vi "utility_panel_multi_axis.vi"() -> (19 "Error Out":errorcluster)   [LabVIEW 2014]
doc: "A Utility Panel that exercises all the primary features of the PMX-4EX-SA controller.\n\nProduced By:\n\n<B>Kod Integrations, LLC</B>\n4835 Marianne Drive\nMount Airy, MD 21771\nhttp://www.kodintegrations.com\nemail: info@kodintegrations.com\nphone: (240) 687-1288"
uses:
  common/controls/motor_status.ctl
  common/controls/complete_motor_state.ctl
  common/controls/single_axis_state.ctl
  common/controls/move_mode.ctl
  common/controls/step_n_loop_motor_status.ctl
  common/controls/jog_pos.ctl
  common/controls/jog_to_strict.ctl
  common/controls/homing_mode.ctl
  common/controls/linear_direction.ctl
  common/controls/axis.ctl
  common/controls/polarity_item.ctl
  common/controls/polarity.ctl
  common/controls/circular_direction.ctl
  common/controls/round_button.ctl
  common/controls/main_test_actions.ctl
  classes/Controller/_Controller.lvclass/_Controller.ctl
  classes/Controller/_Controller.lvclass
  common/controls/multi_axis_read_realtime_actions.ctl
  classes/MultiAxisController/_MultiAxisController.lvclass
  common/controls/counter_type.ctl
  common/controls/motor_enabled_state_axes_group.ctl
  common/controls/movement_item.ctl
  common/controls/digital_output.ctl
  common/controls/step_n_loop_params_write_logic.ctl
  common/controls/step_n_params.ctl
  libraries/common.lvlib
panel:
  in  "pulse_set_u":bool
  in  "pulse_set_z":bool
  in  "pulse_set_y":bool
  in  "pulse_set_x":bool
  in  "pulse_set_val_u":i32
  in  "pulse_set_val_z":i32
  in  "pulse_set_val_y":i32
  in  "pulse_set_val_x":i32
  in  "encoder_set_u":bool
  in  "encoder_set_z":bool
  in  "encoder_set_y":bool
  in  "encoder_set_x":bool
  in  "encoder_set_val_u":i32
  in  "encoder_set_val_z":i32
  in  "encoder_set_val_y":i32
  in  "encoder_set_val_x":i32
  out "U.pulse":i32
  out "Z.pulse":i32
  out "Y.pulse":i32
  out "X.pulse":i32
  in  "exit":bool
  out "response":string
  in  "raw_cmd":string
  in  "write_cmd":bool
  out "U.pos":i32
  out "Z.pos":i32
  out "Y.pos":i32
  out "X.pos":i32
  out "U.SNL_motion_state":T1
  out "U.encoder":i32
  out "U.motion_state":T2
  out "firmware_ver":string
  out "dev_id":string
  out "dev_name":string
  out "Z.SNL_motion_state":T1
  out "Y.SNL_motion_state":T1
  out "X.SNL_motion_state":T1
  out "Z.encoder":i32
  out "Y.encoder":i32
  out "X.encoder":i32
  out "X.motion_state":T2
  out "Y.motion_state":T2
  out "Z.motion_state":T2
  in  "Tab Control":T3(tab)
  in  "goto_interp":bool
  in  "goto_u":bool
  in  "goto_z":bool
  in  "goto_y":bool
  in  "goto_x":bool
  in  "stop_imm_u":bool
  in  "stop_slow_u":bool
  in  "stop_imm_z":bool
  in  "stop_slow_z":bool
  in  "stop_imm_y":bool
  in  "stop_slow_y":bool
  in  "stop_imm_x":bool
  in  "stop_slow_x":bool
  in  "home_dir_u":T4
  in  "home_dir_z":T4
  in  "home_dir_y":T4
  in  "home_dir_x":T4
  in  "jog_dir_u":T4
  in  "jog_dir_z":T4
  in  "jog_dir_y":T4
  in  "jog_dir_x":T4
  in  "mode_u":T5
  in  "home_u":bool
  in  "jog_to_u":T6
  in  "jog_u":T7
  in  "mode_z":T5
  in  "home_z":bool
  in  "jog_to_z":T6
  in  "jog_z":T7
  in  "mode_y":T5
  in  "home_y":bool
  in  "jog_to_y":T6
  in  "jog_y":T7
  in  "mode_x":T5
  in  "home_x":bool
  in  "enabled_u":bool
  in  "enabled_z":bool
  in  "enabled_y":bool
  in  "enabled_x":bool
  in  "jog_to_x":T6
  in  "X.pos_goto":i32
  in  "Y.pos_goto":i32
  in  "Z.pos_goto":i32
  in  "U.pos_goto":i32
  in  "jog_x":T7
  out "sspd_mode_curr":u8=1 min=1 max=7
  in  "t_set_position":bool
  in  "t_position":i32=1
  in  "t_axis":T8
  in  "sspd_set_speed":bool
  in  "sspd_speed":u32=1
  in  "sspd_set_mode":bool
  in  "sspd_mode":u8=1 min=1 max=7
  in  "stop_circ_slow":bool
  in  "stop_circ_imm":bool
  in  "move_circle":bool
  in  "move_arc":bool
  in  "x_coord - arc":i32
  in  "y_coord - arc":i32
  in  "direction - arc":T9
  in  "absolute_angle (degrees) - arc":dbl
  in  "relative_angle (degrees) - arc":dbl
  in  "direction - circle":T9
  in  "y_coord - circle":i32
  in  "x_coord - circle":i32
  in  "stop_arc_slow":bool
  in  "stop_arc_imm":bool
  in  "sspd_axis":T8
  out "step_n_err_range_curr":i32
  out "step_n_tolerance_curr":u32
  out "step_n_ratio_curr":dbl
  out "step_n_max_corr_curr":i32
  in  "set_step_n_params":bool
  in  "step_n_err_range":i32
  in  "step_n_tolerance":u32
  in  "step_n_ratio":dbl
  in  "set_n_correct_attempts":T10
  in  "set_n_err_range?":T10
  in  "set_n_tolerance?":T10
  in  "set_n_ratio?":T10
  in  "step_n_axis":T8
  in  "step_n_max_corr":i32
  in  "enable_disable_step_n":bool
  in  "dig_outs":T11
  out "digital_ins":T12
  out "analog_inputs":T13
  in  "get_non_vol_var":bool
  in  "get_vol_var":bool
  out "non_vol_var_read":string
  out "vol_var_read":string
  in  "set_non_vol_var":bool
  in  "set_vol_var":bool
  in  "non_vol_var_write":i32
  in  "vol_var_write":i32
  in  "non_vol_var_num":u16=50 min=50 max=99
  in  "vol_var_num":u16 max=49
  in  "set_pol_val":bool
  in  "polarity_val":bool
  in  "polarity_option":T14
  out "polarity_out":T15[](array[typedef])
  in  "polarity_axis":T8
  in  "set_device_name":bool
  in  "device_name_id_to_set":i32 min=0 max=99
  out "device_name_to_get":string
  in  "reset_pos":bool
  out "full_state":T16={"X"={"motion_state"=enum."CONST", "other_states"=[]}, "Y"={"motion_state"=enum."CONST", "other_states"=[]}, "Z"={"motion_state"=enum."CONST", "other_states"=[]}, "U"={"motion_state"=enum."CONST", "other_states"=[]}, "buffer_enabled?"=FALSE, "buffer_start"=0, "buffer_end"=0, "avail_buffer"=0, "move_mode"=enum."ABSOLUTE"}
  in  "Error In":errorcluster
  in  "set_speeds":bool
  in  "Z.low_speed":i32
  in  "Y.low_speed":i32
  in  "X.low_speed":i32
  in  "Z.high_speed":i32
  in  "Y.high_speed":i32
  in  "X.high_speed":i32
  out "exit?":bool
  # "Firmware:"
  # "Dev Name:"
  # "Dev ID:"
  # "Positioning and Status"
  # "Encoder\n(Set Value)"
  # "Encoder\n(Read Value)"
  # "Pulse\n(Set Value)"
  # "Pulse\n(Read Value)"
  # "Position"
  # "Current State"
  # "Step N Loop (SNL) State"
  # "(X)"
  # "(Y)"
  # "(Z)"
  # "(U)"
  # "`"
  # "enabled\nstate"
  # "\"Jog To\"\nvalue"
  # "Include?\n(Interpolate)"
  # "Jog\nDirection"
  # "Home\nDirection"
  # "Stop\nSlow"
  # "Stop\nNow!"
  # "axis"
  # "Jog To"
  # "Jog"
  # "Homing Mode"
  # "Home"
  # "(X)"
  # "(Y)"
  # "(Z)"
  # "(U)"
  # "Arc Movements:"
  # "Circular Movements:"
  # "On The Fly Speed (SSPD):"
  # "Axis"
  # "Mode"
  # "Mode (current)"
  # "Speed"
  # "Center X"
  # "Center X"
  # "Center Y"
  # "Center Y"
  # "(mode 1 to 7)"
  # "SET"
  # "SET"
  # "Absolute Angle"
  # "(degrees)"
  # "Direction"
  # "On The Fly Position (T):"
  # "Relative Angle"
  # "(degrees)"
  # "Axis"
  # "Position"
  # "Direction"
  # "SET"
  # "Axis"
  # "Write Values (for chosen Axis)\n(check those to write, then click APPLY)"
  # "Current Values (for chosen Axis)"
  # "Ratio"
  # "Tolerance"
  # "Error Range"
  # "Max Number of Correction Attempts"
  # "Digital Outputs:"
  # "Digital Inputs:"
  # "Analog Inputs:"
  # "Variable ID"
  # "Variable Value (for Write)"
  # "Variable Value (for Read)"
  # "Volatile Variables"
  # "(0-49)"
  # "Non Volatile Variables"
  # "(50-99)"
  # "Axis"
  # "Write Polarity Value"
  # "Current Values (for chosen Axis)"
  # "New Polarity \nValue"
  # "Polarity Type"
  # "Device Name"
  # "SET"
  # "(choose 0 to 99)"
  # "(actual)"
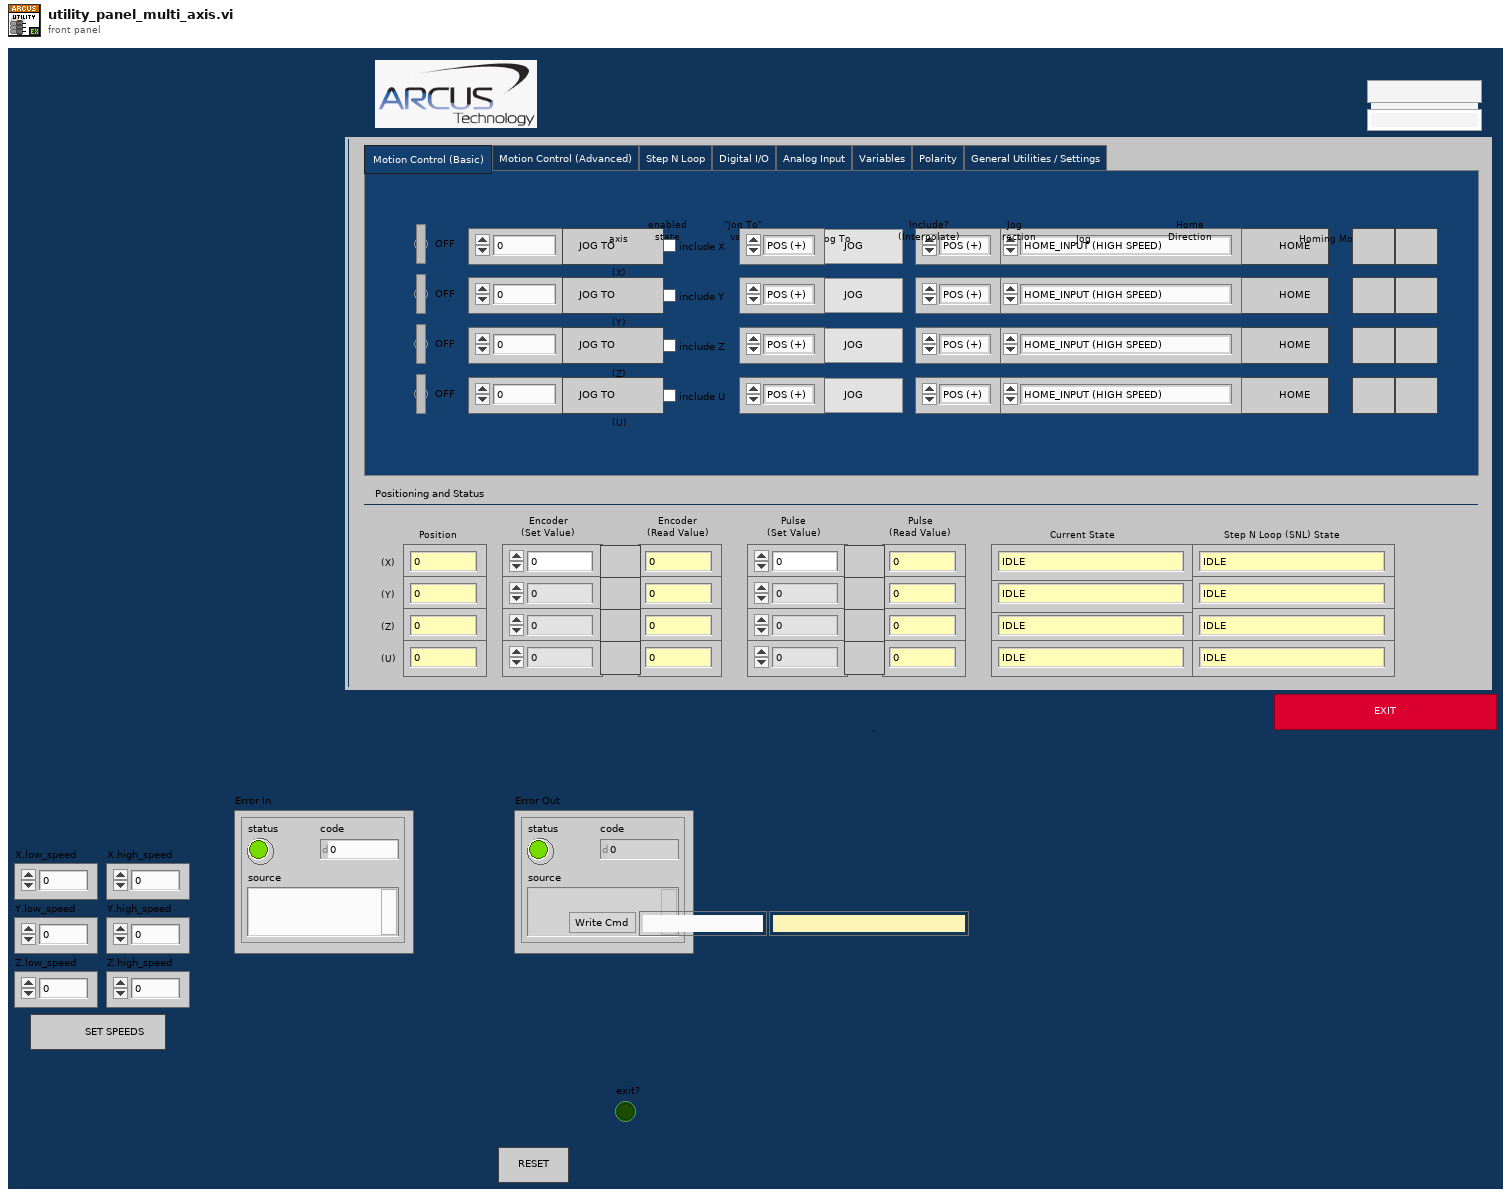
[diagram p1: front panel]
types:
  T1 = typedef "common.lvlib/step_n_loop_motor_status.ctl" = enum16{"IDLE", "MOVING", "CORRECTING", "STOPPING", "ABORTING", "JOGGING", "HOMING", "Z-HOMING", "CORRECT_RANGE_ERR", "CORRECT_ATTEMPT_ERR", "STALL_ERR", "LIMIT_ERR", "NA (SNL NOT ENABLED)", "LIMIT_HOMING"}
  T2 = typedef "common.lvlib/motor_status.ctl" = enum16{"IDLE", "CONST", "ACCEL", "DECEL", "HOME_SWITCH", "-LIMIT_SWITCH", "+LIMIT_SWITCH", "-LIMIT_ERR", "+LIMIT_ERR", "COMM_TIMEOUT", "ALARM_INPUT", "ALARM_ERROR", "TOC_TIMEOUT_STATUS", "LATCH_INPUT_STATUS", "Z_INDEX_STATUS"}
  T3 = enum32{"Motion Control (Basic) ", "Motion Control (Advanced)", "Step N Loop", "Digital I/O", "Analog Input", "Variables", "Polarity", "General Utilities / Settings"}
  T4 = typedef "common.lvlib/linear_direction.ctl" = enum16{"POS (+)", "NEG (-)"}
  T5 = typedef "common.lvlib/homing_mode.ctl" = enum16{"HOME_INPUT (HIGH SPEED)", "LIMIT_INPUT", "HOME_INPUT_&_Z-INDEX", "Z-INDEX", "HOME_INPUT (HIGH_&_LOW_SPEED)"}
  T6 = typedef "common.lvlib/jog_to_strict.ctl" = bool
  T7 = typedef "common.lvlib/jog_pos.ctl" = bool
  T8 = typedef "common.lvlib/axis.ctl" = enum16{"X", "Y", "Z", "U"}
  T9 = typedef "common.lvlib/circular_direction.ctl" = enum16{"CCW", "CW"}
  T10 = typedef "common.lvlib/round_button.ctl" = bool
  T11 = cluster{"Digital Output 1":bool, "Digital Output 2":bool, "Digital Output 3":bool, "Digital Output 4":bool, "Digital Output 5":bool, "Digital Output 6":bool, "Digital Output 7":bool, "Digital Output 8":bool}
  T12 = cluster{"Digital Input 1":bool, "Digital Input 2":bool, "Digital Input 3":bool, "Digital Input 4":bool, "Digital Input 5":bool, "Digital Input 6":bool, "Digital Input 7":bool, "Digital Input 8":bool}
  T13 = cluster{"Analog Input 1":dbl, "Analog Input 2":dbl, "Analog Input 3":dbl, "Analog Input 4":dbl, "Analog Input 5":dbl, "Analog Input 6":dbl, "Analog Input 7":dbl, "Analog Input 8":dbl}
  T14 = typedef "common.lvlib/polarity.ctl" = enum16{"DIRECTION", "LIMIT", "HOME", "DIG_OUT", "DIG_IN", "ENABLE_OUT", "JUMP_ERR", "LATCH", "Z-CHAN_INDEX", "ENCODER_DECODING:1X", "ENCODER_DECODING:2X", "ENCODER_DECODING:4X", "ALARM", "STANDALONE_ERR", "-", "<reserved/nc>"}
  T15 = typedef "common.lvlib/polarity_item.ctl" = cluster{"item":T14, "status":bool}
  T16 = typedef "common.lvlib/complete_motor_state.ctl" = cluster{"X":T17, "Y":T17, "Z":T17, "U":T17, "buffer_enabled?":bool, "buffer_start":i32, "buffer_end":i32, "avail_buffer":i32, "move_mode":T18}
  T17 = typedef "common.lvlib/single_axis_state.ctl" = cluster{"motion_state":T2, "other_states":T2[]}
  T18 = typedef "common.lvlib/move_mode.ctl" = enum16{"ABSOLUTE", "INCREMENTAL"}
  T19 = typedef "common.lvlib/main_test_actions.ctl" = enum16{"-------------------------", "about", "adjust_goto_buttons", "check_model", "close", "connect", "disable_all", "disable_step_n_loop", "enable_all", "enabled_state_change", "enable_step_n_loop", "exit", "get_device_id", "get_device_name", "get_digital_inputs", "get_digital_outputs", "get_firmware_ver", "get_high_speed", "get_high_speed_global", "get_low_speed", "get_low_speed_global", "get_non_volatile_var", "get_on_fly_speed_mode", "get_polarity", "get_product_id", "get_sspd_mode", "get_step_n_params", "get_volatile_var", "goto_x", "goto_y", "goto_z", "goto_u", "goto_interp", "home_x", "home_y", "home_z", "home_u", "init", "init_ui", "jog_x", "jog_y", "jog_z", "jog_u", "lock", "move_arc", "move_circular", "process_events", "run_standalone", "select_device", "stop_standalone", "set_device_name", "set_digital_outputs", "set_encoder_x", "set_encoder_y", "set_encoder_z", "set_encoder_u", "set_high_speed", "set_low_speed", "set_non_volatile_var", "set_on_fly_position", "set_on_fly_speed", "set_on_fly_speed_mode", "set_polarity", "set_pulse_x", "set_pulse_y", "set_pulse_z", "set_pulse_u", "set_step_n_params", "set_volatile_var", "stop_imm_x", "stop_imm_y", "stop_imm_z", "stop_imm_u", "stop_slow_x", "stop_slow_y", "stop_slow_z", "stop_slow_u", "store_perm", "unlock", "wait_til_idle", "zero_counter", "zero_position"}
  T20 = typedef "common.lvlib/models.ctl" = enum16{"<unrecognized>", "ACE-SDC", "ACE-SDE", "ACE-SXC", "ACE-SXE", "DMX-CAN", "DMX-J-SA", "DMX-K-SA", "DMX-UMD", "PMX-2ED-SA", "PMX-2EX-SA", "PMX-4CX-SA", "PMX-4EX-SA"}
  T21 = typedef "common.lvlib/motor_enabled_state_axes_group.ctl" = cluster{"x-axis":bool, "y-axis":bool, "z-axis":bool, "u-axis":bool}
  T22 = typedef "common.lvlib/movement_item.ctl" = cluster{"axis":T8, "target":i32}
  T23 = enum8{"Enabled", "Disabled", "Disabled and Grayed Out"}
  T24 = typedef "common.lvlib/multi_axis_read_realtime_actions.ctl" = enum16{"analog_inputs", "build_processes", "check_status", "encoder_value", "digital_inputs", "motion_state", "position_value", "pulse_value", "snl_motion_state"}
  T25 = typedef "common.lvlib/counter_type.ctl" = enum16{"ENCODER", "PULSE"}
  T26 = typedef "common.lvlib/digital_output_item.ctl" = cluster{"item":T27, "status":bool}
  T27 = typedef "common.lvlib/digital_output.ctl" = enum16{"DIG_OUT_1", "DIG_OUT_2", "DIG_OUT_3", "DIG_OUT_4", "DIG_OUT_5", "DIG_OUT_6", "DIG_OUT_7", "DIG_OUT_8"}
  T28 = cluster{"[0]":bool, "[1]":bool, "[2]":bool, "[3]":bool, "[4]":bool, "[5]":bool, "[6]":bool, "[7]":bool}
  T29 = typedef "common.lvlib/step_n_params.ctl" = cluster{"step_N_loop_ratio":dbl, "tolerance (encoder counts)":u32, "error_range":i32, "max_num_correction_attempts":i32, "enabled?":bool}
  T30 = typedef "common.lvlib/step_n_loop_params_write_logic.ctl" = cluster{"set_ratio?":bool, "set_tolerance?":bool, "set_err_range?":bool, "set_correct_attempts?":bool}
  T31 = typedef "common.lvlib/counter_values.ctl" = cluster{"X":i32, "Y":i32, "Z":i32, "U":i32}
  T32 = typedef "common.lvlib/digital_input_item.ctl" = cluster{"item":T33, "status":bool}
  T33 = typedef "common.lvlib/digital_input.ctl" = enum16{"DIG_IN_1", "DIG_IN_2", "DIG_IN_3", "DIG_IN_4", "DIG_IN_5", "DIG_IN_6", "DIG_IN_7", "DIG_IN_8", "NEG_LIMIT", "HOME", "POS_LIMIT"}
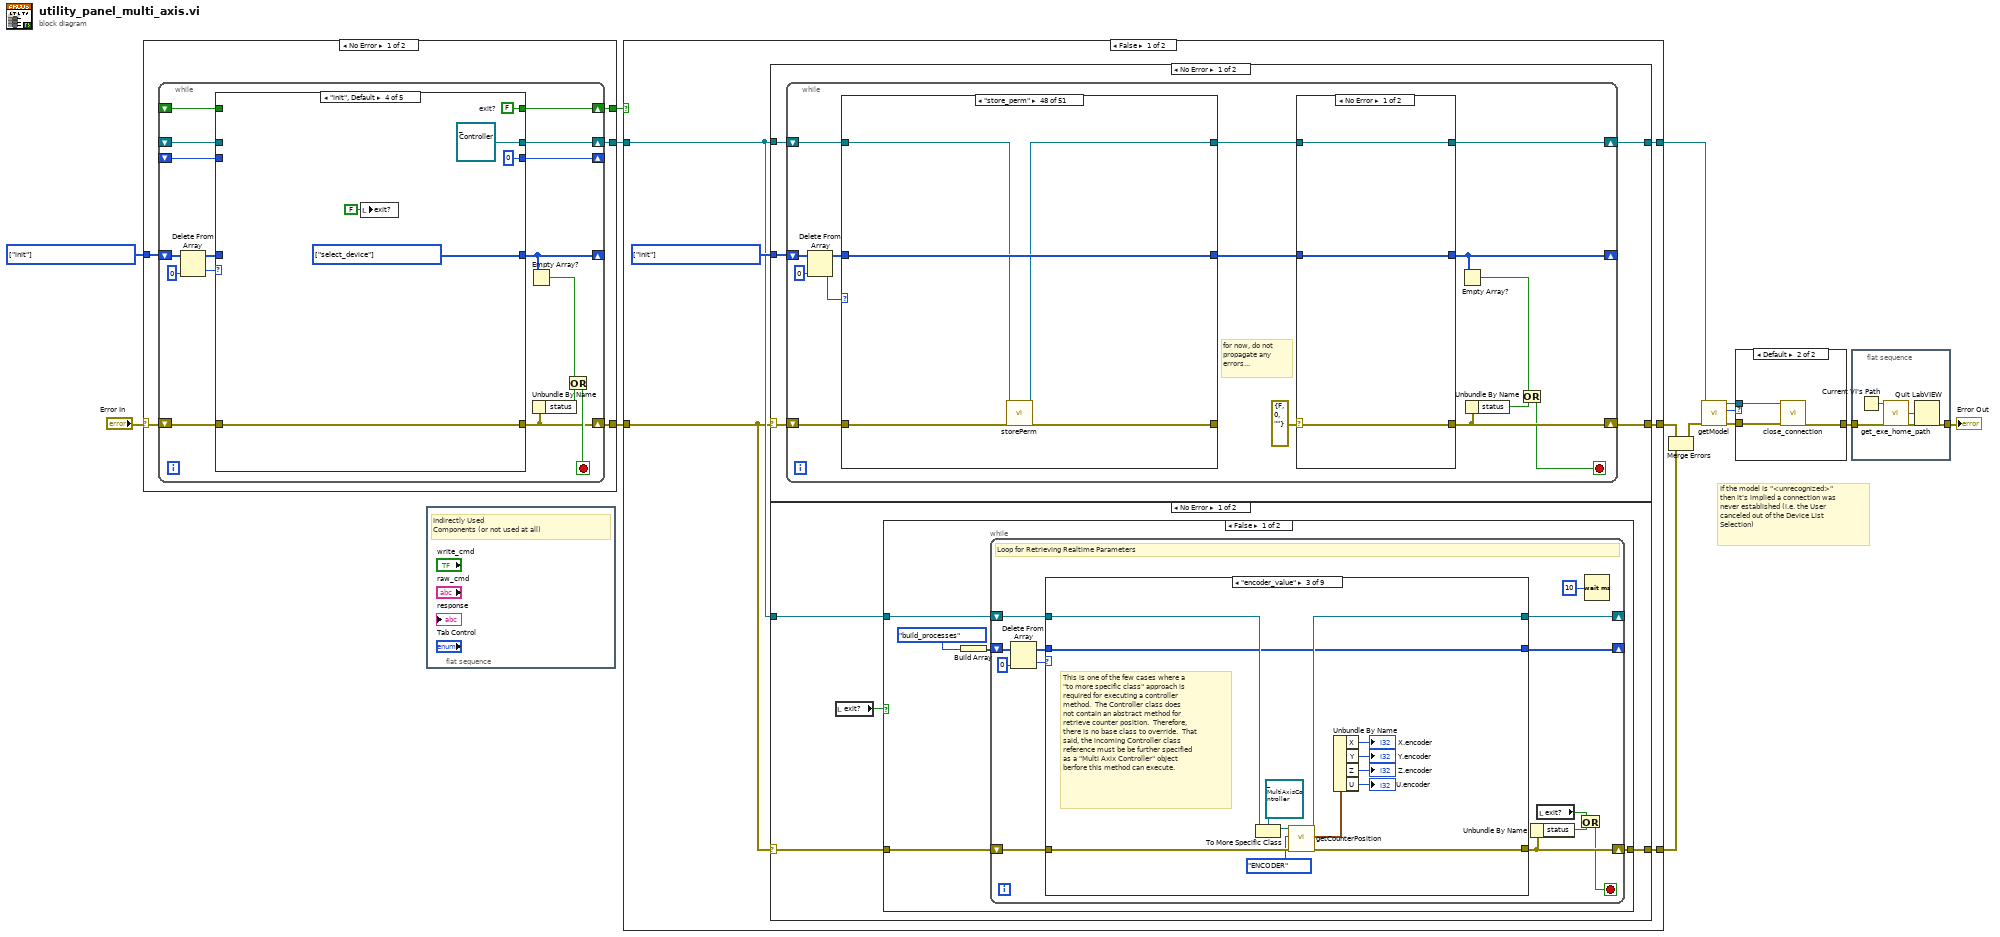
[diagram p0: block diagram]
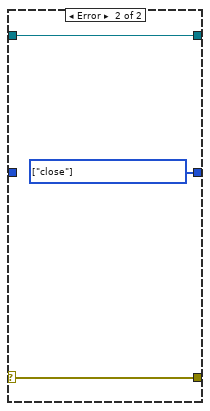
[diagram p3: hidden frame]
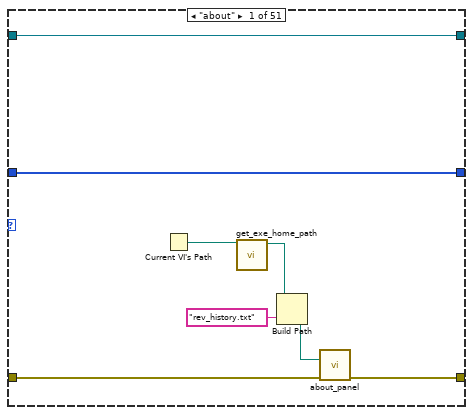
[diagram p4: hidden frame]
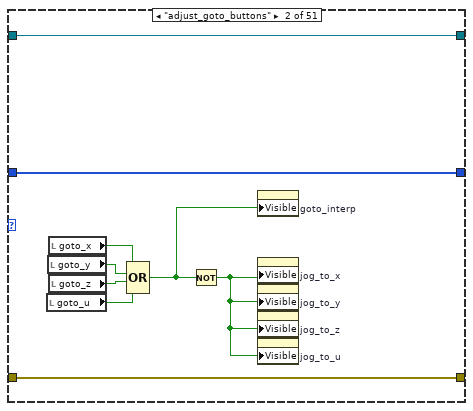
[diagram p5: hidden frame]
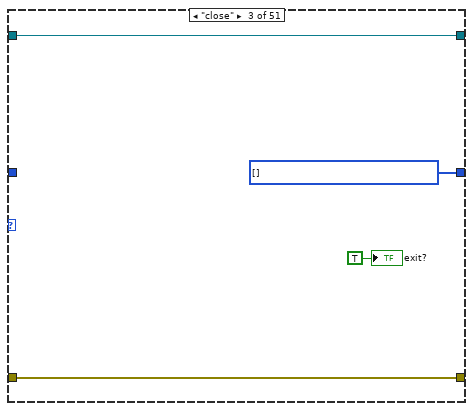
[diagram p6: hidden frame]
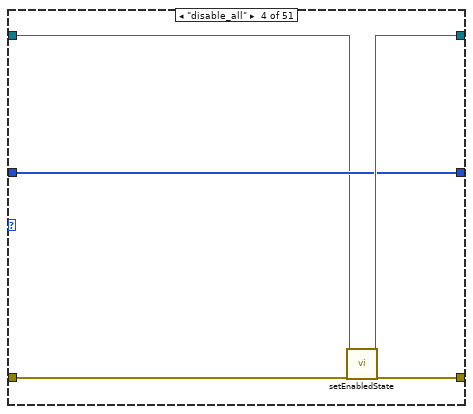
[diagram p7: hidden frame]
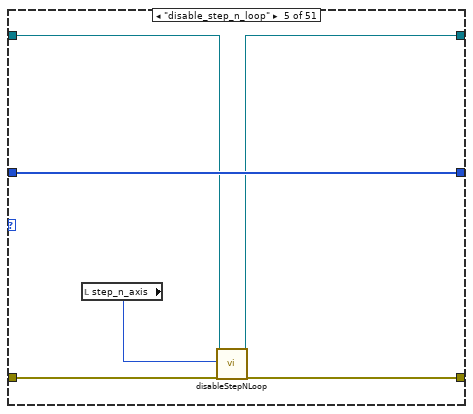
[diagram p8: hidden frame]
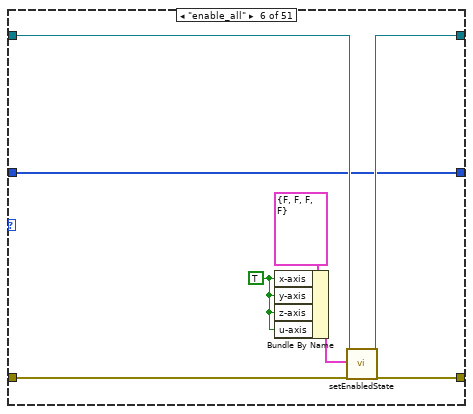
[diagram p9: hidden frame]
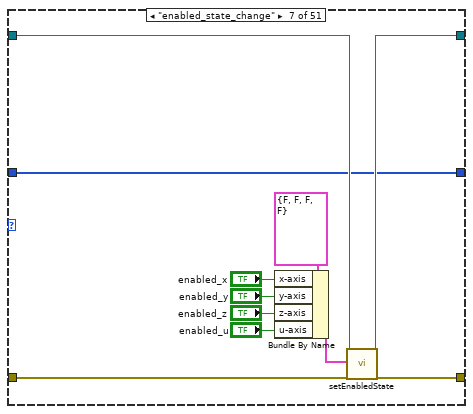
[diagram p10: hidden frame]
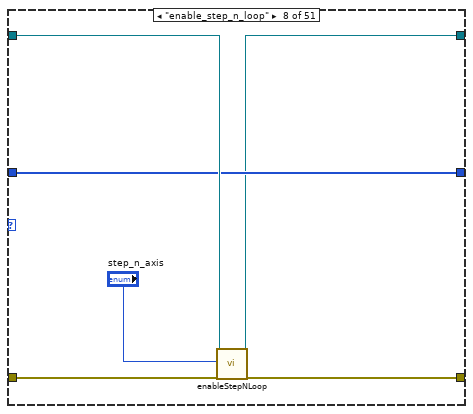
[diagram p11: hidden frame]
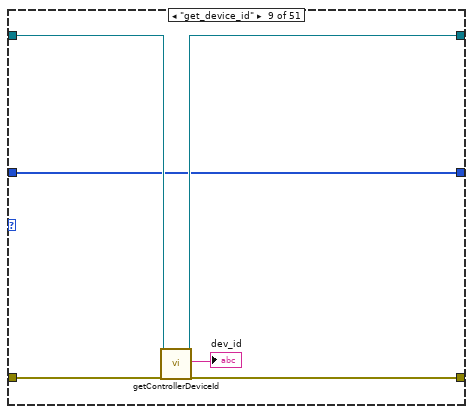
[diagram p12: hidden frame]
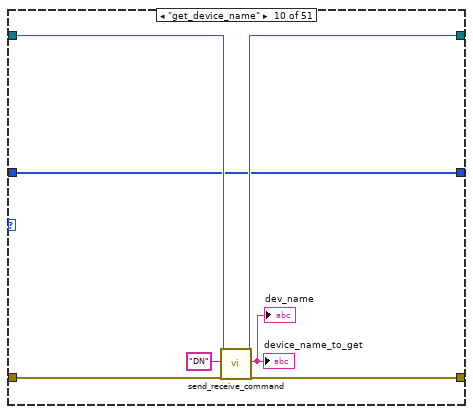
[diagram p13: hidden frame]
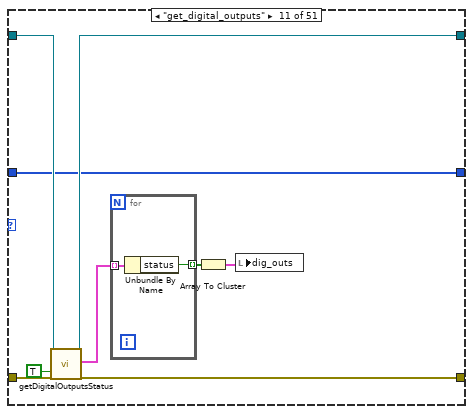
[diagram p14: hidden frame]
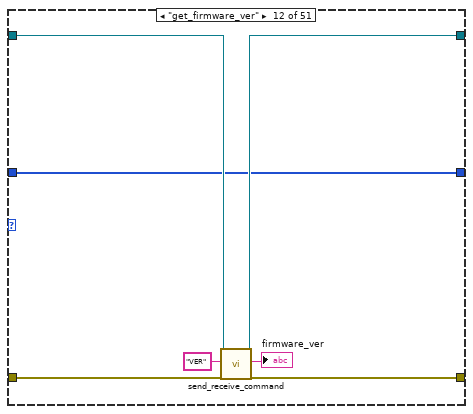
[diagram p15: hidden frame]
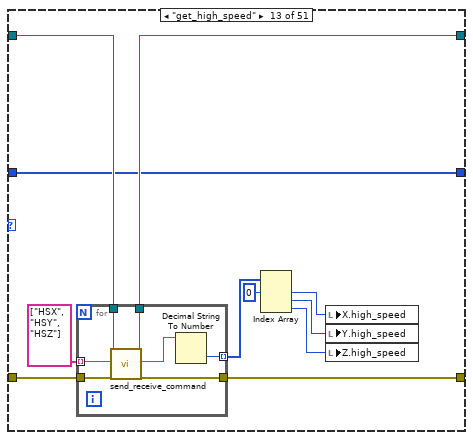
[diagram p16: hidden frame]
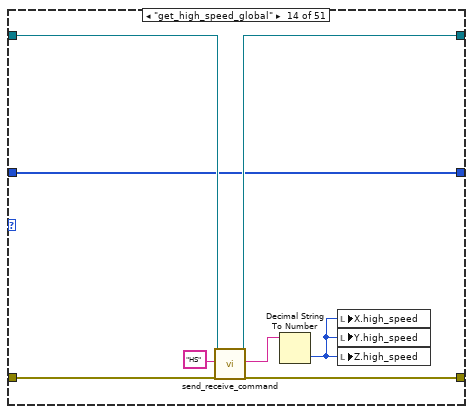
[diagram p17: hidden frame]
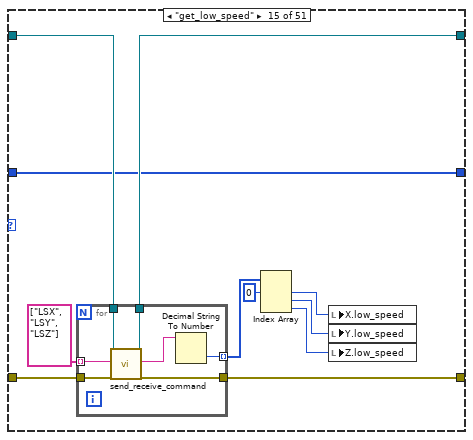
[diagram p18: hidden frame]
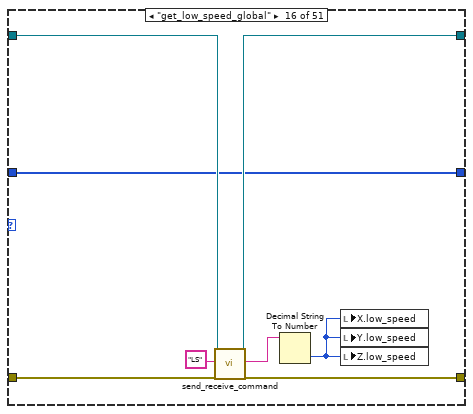
[diagram p19: hidden frame]
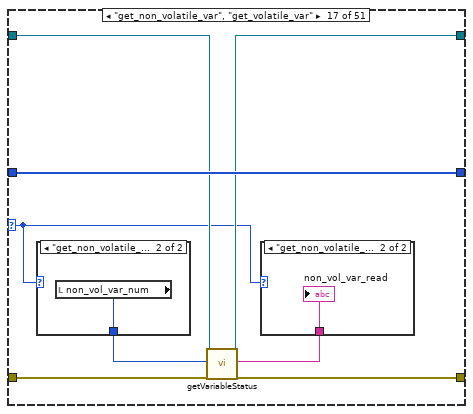
[diagram p20: hidden frame]
diagram:
  w12 = T19[] [enum."init"] items=["-------------------------", "about", "adjust_goto_buttons", "check_model", "close", "connect", "disable_all", "disable_step_n_loop", "enable_all", "enabled_state_change", "enable_step_n_loop", "exit", "get_device_id", "get_device_name", "get_digital_inputs", "get_digital_outputs", "get_firmware_ver", "get_high_speed", "get_high_speed_global", "get_low_speed", "get_low_speed_global", "get_non_volatile_var", "get_on_fly_speed_mode", "get_polarity", "get_product_id", "get_sspd_mode", "get_step_n_params", "get_volatile_var", "goto_x", "goto_y", "goto_z", "goto_u", "goto_interp", "home_x", "home_y", "home_z", "home_u", "init", "init_ui", "jog_x", "jog_y", "jog_z", "jog_u", "lock", "move_arc", "move_circular", "process_events", "run_standalone", "select_device", "stop_standalone", "set_device_name", "set_digital_outputs", "set_encoder_x", "set_encoder_y", "set_encoder_z", "set_encoder_u", "set_high_speed", "set_low_speed", "set_non_volatile_var", "set_on_fly_position", "set_on_fly_speed", "set_on_fly_speed_mode", "set_polarity", "set_pulse_x", "set_pulse_y", "set_pulse_z", "set_pulse_u", "set_step_n_params", "set_volatile_var", "stop_imm_x", "stop_imm_y", "stop_imm_z", "stop_imm_u", "stop_slow_x", "stop_slow_y", "stop_slow_z", "stop_slow_u", "store_perm", "unlock", "wait_til_idle", "zero_counter", "zero_position"]
  # "If the model is \"<unrecognized>\"\nthen it's implied a connection was\nnever established (i.e. the User\ncanceled out of the Device List\nSelection)"
  n1 = case shown="No Error" "Error In" {
    selector: "Error In" -> [w16 w84]
    tunnel: [w19 refnum<class "_Controller.lvclass"> refnum ("reference (out)")] -> w10
    tunnel: w12 -> [w18 _]
    tunnel: [w17 w84] -> w9
    tunnel: [w15 w82] -> w8
    frame No Error {
      n2 = while {
        shift-right: [w29] -> _
        shift-left: w18 -> [w35]
        shift-right: [w26] -> w17
        shift-left: w16 -> [w27]
        shift-right: [w24] -> w19
        shift-left: _ -> [w25]
        shift-right: [w23] -> _
        shift-left: _ -> [w22]
        shift-right: [w21] -> w15
        shift-left: _ -> [w20]
        stop <- w31 stop-if-true
        n3 = Delete From Array(array=w35, index=0) -> (deleted portion=w30:T19, array with subset deleted=w28:T19[])  [unwired: 1 in]
        n4 = case shown="\"init\", Default" w30 {
          tunnel: [w41 w54 w62 w69 w76] -> w29
          tunnel: w28 -> [w40 w54 _ _ _]
          tunnel: w27 -> [w43 w57 w60 w66 w77]
          tunnel: [w42 w56 w60 w66 w75] -> w26
          tunnel: w25 -> [w39 _ w63 _ w72]
          tunnel: [w38 w58 w63 refnum<class "_Controller.lvclass"> refnum ("reference (out)") w72] -> w24
          tunnel: [w37 w55 w61 0 ("index") w71] -> w23
          tunnel: w22 -> [w37 w55 w61 _ _]
          tunnel: [w36 w53 w59 w65 w70] -> w21
          tunnel: w20 -> [w36 w53 _ _ w70]
          frame "check_model" {
            n5 = call "getModel.vi"("error in (no error)"=w43, "reference (in)"=w39) -> ("error out"=w44:errorcluster, "model"=w45:T20, "reference (out)"=w38:refnum<class "_Controller.lvclass">)  [unwired: 7 in]
            n6 = case shown="Default" w45 {
              selector: w45 -> [w47 _]
              tunnel: [w50 w52] -> w42
              tunnel: w44 -> [w50 w52]
              tunnel: [w46 w51] -> w41
              tunnel: w40 -> [_ w51]
              frame Default {
                w46 = T19[] [enum."exit"] items=["-------------------------", "about", "adjust_goto_buttons", "check_model", "close", "connect", "disable_all", "disable_step_n_loop", "enable_all", "enabled_state_change", "enable_step_n_loop", "exit", "get_device_id", "get_device_name", "get_digital_inputs", "get_digital_outputs", "get_firmware_ver", "get_high_speed", "get_high_speed_global", "get_low_speed", "get_low_speed_global", "get_non_volatile_var", "get_on_fly_speed_mode", "get_polarity", "get_product_id", "get_sspd_mode", "get_step_n_params", "get_volatile_var", "goto_x", "goto_y", "goto_z", "goto_u", "goto_interp", "home_x", "home_y", "home_z", "home_u", "init", "init_ui", "jog_x", "jog_y", "jog_z", "jog_u", "lock", "move_arc", "move_circular", "process_events", "run_standalone", "select_device", "stop_standalone", "set_device_name", "set_digital_outputs", "set_encoder_x", "set_encoder_y", "set_encoder_z", "set_encoder_u", "set_high_speed", "set_low_speed", "set_non_volatile_var", "set_on_fly_position", "set_on_fly_speed", "set_on_fly_speed_mode", "set_polarity", "set_pulse_x", "set_pulse_y", "set_pulse_z", "set_pulse_u", "set_step_n_params", "set_volatile_var", "stop_imm_x", "stop_imm_y", "stop_imm_z", "stop_imm_u", "stop_slow_x", "stop_slow_y", "stop_slow_z", "stop_slow_u", "store_perm", "unlock", "wait_til_idle", "zero_counter", "zero_position"]
                n7 = Format Into String(format string="This Control Panel is intended for Multi Axis applications only, with primary focus on the PMX-4EX-SA.  The attached model '%s' is not 100 percent supported in this tool.  Please refer to the example section for a variety of sample codes to suit your needs.\n\nThe application will now close.", w47) -> (resulting string=w48:string)  [unwired: 2 in, 1 out]
                n8 = One Button Dialog(message=w48) -> ()  [unwired: 1 in, 1 out]
              }
              frame "PMX-4EX-SA" {
                # "fully supported"
              }
            }
          }
          frame "connect" {
            n9 = call "initialize.vi"("device_index (in) [0=def]"=w55, "error in (no error)"=w57) -> ("reference (out)"=w58:refnum<class "_Controller.lvclass">, "error out"=w56:errorcluster)  [unwired: 16 in]
          }
          frame "exit" {
            w59 = TRUE  # exit?
            w62 = T19[] [] items=["-------------------------", "about", "adjust_goto_buttons", "check_model", "close", "connect", "disable_all", "disable_step_n_loop", "enable_all", "enabled_state_change", "enable_step_n_loop", "exit", "get_device_id", "get_device_name", "get_digital_inputs", "get_digital_outputs", "get_firmware_ver", "get_high_speed", "get_high_speed_global", "get_low_speed", "get_low_speed_global", "get_non_volatile_var", "get_on_fly_speed_mode", "get_polarity", "get_product_id", "get_sspd_mode", "get_step_n_params", "get_volatile_var", "goto_x", "goto_y", "goto_z", "goto_u", "goto_interp", "home_x", "home_y", "home_z", "home_u", "init", "init_ui", "jog_x", "jog_y", "jog_z", "jog_u", "lock", "move_arc", "move_circular", "process_events", "run_standalone", "select_device", "stop_standalone", "set_device_name", "set_digital_outputs", "set_encoder_x", "set_encoder_y", "set_encoder_z", "set_encoder_u", "set_high_speed", "set_low_speed", "set_non_volatile_var", "set_on_fly_position", "set_on_fly_speed", "set_on_fly_speed_mode", "set_polarity", "set_pulse_x", "set_pulse_y", "set_pulse_z", "set_pulse_u", "set_step_n_params", "set_volatile_var", "stop_imm_x", "stop_imm_y", "stop_imm_z", "stop_imm_u", "stop_slow_x", "stop_slow_y", "stop_slow_z", "stop_slow_u", "store_perm", "unlock", "wait_til_idle", "zero_counter", "zero_position"]
          }
          frame "init", Default {
            w65 = FALSE  # exit?
            w69 = T19[] [enum."select_device"] items=["-------------------------", "about", "adjust_goto_buttons", "check_model", "close", "connect", "disable_all", "disable_step_n_loop", "enable_all", "enabled_state_change", "enable_step_n_loop", "exit", "get_device_id", "get_device_name", "get_digital_inputs", "get_digital_outputs", "get_firmware_ver", "get_high_speed", "get_high_speed_global", "get_low_speed", "get_low_speed_global", "get_non_volatile_var", "get_on_fly_speed_mode", "get_polarity", "get_product_id", "get_sspd_mode", "get_step_n_params", "get_volatile_var", "goto_x", "goto_y", "goto_z", "goto_u", "goto_interp", "home_x", "home_y", "home_z", "home_u", "init", "init_ui", "jog_x", "jog_y", "jog_z", "jog_u", "lock", "move_arc", "move_circular", "process_events", "run_standalone", "select_device", "stop_standalone", "set_device_name", "set_digital_outputs", "set_encoder_x", "set_encoder_y", "set_encoder_z", "set_encoder_u", "set_high_speed", "set_low_speed", "set_non_volatile_var", "set_on_fly_position", "set_on_fly_speed", "set_on_fly_speed_mode", "set_polarity", "set_pulse_x", "set_pulse_y", "set_pulse_z", "set_pulse_u", "set_step_n_params", "set_volatile_var", "stop_imm_x", "stop_imm_y", "stop_imm_z", "stop_imm_u", "stop_slow_x", "stop_slow_y", "stop_slow_z", "stop_slow_u", "store_perm", "unlock", "wait_til_idle", "zero_counter", "zero_position"]
            n10 = local write "exit?"(FALSE ("exit?")) -> ()
          }
          frame "select_device" {
            n11 = call "device_selector_panel.vi"("error in (no error)"=w77) -> ("index"=w71:i32, "cancel?"=w73:bool, "error out"=w74:errorcluster)  [unwired: 10 in, 2 out]
            n12 = case shown="True" w73 {
              tunnel: [w79 w81] -> w76
              tunnel: w74 -> [w78 w80]
              tunnel: [w78 w80] -> w75
              frame False {
                w79 = T19[] [enum."connect", enum."check_model"] items=["-------------------------", "about", "adjust_goto_buttons", "check_model", "close", "connect", "disable_all", "disable_step_n_loop", "enable_all", "enabled_state_change", "enable_step_n_loop", "exit", "get_device_id", "get_device_name", "get_digital_inputs", "get_digital_outputs", "get_firmware_ver", "get_high_speed", "get_high_speed_global", "get_low_speed", "get_low_speed_global", "get_non_volatile_var", "get_on_fly_speed_mode", "get_polarity", "get_product_id", "get_sspd_mode", "get_step_n_params", "get_volatile_var", "goto_x", "goto_y", "goto_z", "goto_u", "goto_interp", "home_x", "home_y", "home_z", "home_u", "init", "init_ui", "jog_x", "jog_y", "jog_z", "jog_u", "lock", "move_arc", "move_circular", "process_events", "run_standalone", "select_device", "stop_standalone", "set_device_name", "set_digital_outputs", "set_encoder_x", "set_encoder_y", "set_encoder_z", "set_encoder_u", "set_high_speed", "set_low_speed", "set_non_volatile_var", "set_on_fly_position", "set_on_fly_speed", "set_on_fly_speed_mode", "set_polarity", "set_pulse_x", "set_pulse_y", "set_pulse_z", "set_pulse_u", "set_step_n_params", "set_volatile_var", "stop_imm_x", "stop_imm_y", "stop_imm_z", "stop_imm_u", "stop_slow_x", "stop_slow_y", "stop_slow_z", "stop_slow_u", "store_perm", "unlock", "wait_til_idle", "zero_counter", "zero_position"]
              }
              frame True {
                w81 = T19[] [enum."exit"] items=["-------------------------", "about", "adjust_goto_buttons", "check_model", "close", "connect", "disable_all", "disable_step_n_loop", "enable_all", "enabled_state_change", "enable_step_n_loop", "exit", "get_device_id", "get_device_name", "get_digital_inputs", "get_digital_outputs", "get_firmware_ver", "get_high_speed", "get_high_speed_global", "get_low_speed", "get_low_speed_global", "get_non_volatile_var", "get_on_fly_speed_mode", "get_polarity", "get_product_id", "get_sspd_mode", "get_step_n_params", "get_volatile_var", "goto_x", "goto_y", "goto_z", "goto_u", "goto_interp", "home_x", "home_y", "home_z", "home_u", "init", "init_ui", "jog_x", "jog_y", "jog_z", "jog_u", "lock", "move_arc", "move_circular", "process_events", "run_standalone", "select_device", "stop_standalone", "set_device_name", "set_digital_outputs", "set_encoder_x", "set_encoder_y", "set_encoder_z", "set_encoder_u", "set_high_speed", "set_low_speed", "set_non_volatile_var", "set_on_fly_position", "set_on_fly_speed", "set_on_fly_speed_mode", "set_polarity", "set_pulse_x", "set_pulse_y", "set_pulse_z", "set_pulse_u", "set_step_n_params", "set_volatile_var", "stop_imm_x", "stop_imm_y", "stop_imm_z", "stop_imm_u", "stop_slow_x", "stop_slow_y", "stop_slow_z", "stop_slow_u", "store_perm", "unlock", "wait_til_idle", "zero_counter", "zero_position"]
              }
            }
          }
        }
        n13 = Empty Array?(array=w29) -> (empty?=w33:bool)
        n14 = Unbundle By Name(w26) -> ("status"=w32:bool)
        n15 = Or(x=w33, y=w32) -> (x .or. y?=w31:bool)
      }
    }
    frame Error {
      w82 = TRUE  # exit?
    }
  }
  n16 = flat-sequence {
    frame #0 {
      # "Indirectly Used \nComponents (or not used at all)"
    }
  }
  n17 = case shown="False" w8 {
    tunnel: [w90 w984] -> w6
    tunnel: [w89 w983] -> w14
    tunnel: [w88 w983] -> w13
    tunnel: w10 -> [w86 w984]
    tunnel: w9 -> [w85 w983]
    frame False {
      w87 = T19[] [enum."init"] items=["-------------------------", "about", "adjust_goto_buttons", "check_model", "close", "connect", "disable_all", "disable_step_n_loop", "enable_all", "enabled_state_change", "enable_step_n_loop", "exit", "get_device_id", "get_device_name", "get_digital_inputs", "get_digital_outputs", "get_firmware_ver", "get_high_speed", "get_high_speed_global", "get_low_speed", "get_low_speed_global", "get_non_volatile_var", "get_on_fly_speed_mode", "get_polarity", "get_product_id", "get_sspd_mode", "get_step_n_params", "get_volatile_var", "goto_x", "goto_y", "goto_z", "goto_u", "goto_interp", "home_x", "home_y", "home_z", "home_u", "init", "init_ui", "jog_x", "jog_y", "jog_z", "jog_u", "lock", "move_arc", "move_circular", "process_events", "run_standalone", "select_device", "stop_standalone", "set_device_name", "set_digital_outputs", "set_encoder_x", "set_encoder_y", "set_encoder_z", "set_encoder_u", "set_high_speed", "set_low_speed", "set_non_volatile_var", "set_on_fly_position", "set_on_fly_speed", "set_on_fly_speed_mode", "set_polarity", "set_pulse_x", "set_pulse_y", "set_pulse_z", "set_pulse_u", "set_step_n_params", "set_volatile_var", "stop_imm_x", "stop_imm_y", "stop_imm_z", "stop_imm_u", "stop_slow_x", "stop_slow_y", "stop_slow_z", "stop_slow_u", "store_perm", "unlock", "wait_til_idle", "zero_counter", "zero_position"]
      n18 = case shown="No Error" w85 {
        selector: w85 -> [w91 w827]
        tunnel: [w95 w826] -> w90
        tunnel: w86 -> [w94 w826]
        tunnel: w87 -> [w93 _]
        tunnel: [w92 w827] -> w89
        frame No Error {
          n19 = while {
            shift-right: [w102] -> _
            shift-left: w93 -> [w110]
            shift-right: [w100] -> w92
            shift-left: w91 -> [w106]
            shift-right: [w101] -> w95
            shift-left: w94 -> [w105]
            stop <- w97 stop-if-true
            # "for now, do not\npropagate any\nerrors..."
            n20 = Delete From Array(array=w110, index=0) -> (deleted portion=w108:T19, array with subset deleted=w107:T19[])  [unwired: 1 in]
            n21 = case shown="\"store_perm\"" w108 {
              selector: w108 -> [_ _ _ _ _ _ _ _ _ _ _ _ _ _ _ _ w258 _ _ _ _ w309 _ w355 _ _ w386 _ _ _ _ _ _ _ w617 _ _ _ _ _ _ _ w712 _ _ w757 w768 _ _ _ _]
              tunnel: [w119 w133 w135 w142 w145 w155 w166 w170 w176 w182 w192 w199 w213 w228 w239 w254 w261 w274 w284 w288 w301 w312 w339 w357 w375 w383 w388 w407 w418 w428 w560 w568 w581 w608 w619 w642 w659 w670 w680 w687 w694 w700 w714 w744 w748 w759 w770 w780 w785 w807 w818] -> w103
              tunnel: [w118 w132 w137 w139 w148 w150 w161 w171 w175 w181 w188 w198 w205 w226 w231 w252 w264 w273 w281 w287 w302 w314 w325 w356 w374 w379 w387 w406 w417 w426 w562 w566 w580 w602 w618 w638 w652 w676 w677 w686 w693 w702 w713 w743 w755 w758 w769 w782 w783 w805 w816] -> w104
              tunnel: w107 -> [w118 w132 _ w139 w148 w150 w161 w171 w175 w181 w188 w198 w205 w226 w231 w252 w264 w273 w281 w287 w302 w314 w325 w356 _ w380 w387 w406 w417 w425 w562 w566 w580 w602 w618 w638 w652 w676 w677 w686 w693 w702 w713 w743 w755 w758 w769 w782 w783 w805 w816]
              tunnel: w106 -> [w121 w131 w136 w141 w147 w154 w165 w173 w179 w185 w195 w203 w215 w230 w241 w256 w263 w278 w285 w291 w304 w311 w338 w360 w373 w382 w391 w412 w423 w427 w564 w570 w579 w607 w622 w644 w661 w675 w683 w690 w698 w709 w717 w747 w754 w762 w773 w779 w787 w809 w820]
              tunnel: [w120 w131 w136 w140 w143 w153 w164 w169 w178 w184 w194 w202 w212 w227 w238 w253 w260 w277 w283 w290 w300 w310 w337 w359 w373 w382 w390 w405 w416 w424 w559 w567 w582 w606 w621 w641 w658 w669 w682 w689 w697 w701 w716 w746 w749 w761 w772 w778 w784 w806 w817] -> _
              tunnel: w105 -> [w119 w133 w135 w138 w146 w156 w167 w172 w177 w183 w193 w200 w214 w229 w240 w255 w262 w275 w286 w289 w303 w313 w340 w358 w375 w383 w389 w411 w422 w428 w563 w569 w576 w609 w620 w643 w660 w671 w681 w688 w695 w710 w715 w745 w752 w760 w771 w781 w786 w808 w819]
              frame "about" {
                n22 = Current VI's Path() -> (path=w117:path)
                n23 = call "get_exe_home_path.vi"("home_path"=w117) -> ("actual_home_path"=w122:path)  [unwired: 6 in, 1 out]
                n24 = Build Path(base path=w122, name or relative path="rev_history.txt") -> (appended path=w123:path)
                n25 = call "about_panel.vi"("rev_history_filepath"=w123, "error in (no error)"=w121) -> ("error out"=w120:errorcluster)  [unwired: 13 in]
              }
              frame "adjust_goto_buttons" {
                n26 = local read "goto_u"() -> (w129:bool)
                n27 = local read "goto_y"() -> (w128:bool)
                n28 = local read "goto_x"() -> (w130:bool)
                n29 = local read "goto_z"() -> (w127:bool)
                n30 = Compound Arithmetic op=OR(w130, w128, w127, w129) -> (w126:bool)
                n31 = Not(x=w126) -> (.not. x?=w125:bool)
                n32 = property on="goto_interp" class="Bool"("Visible"=w126) -> ()  [unwired: 2 in, 2 out]
                n33 = property on="jog_to_x" class="Bool"("Visible"=w125) -> ()  [unwired: 2 in, 2 out]
                n34 = property on="jog_to_y" class="Bool"("Visible"=w125) -> ()  [unwired: 2 in, 2 out]
                n35 = property on="jog_to_z" class="Bool"("Visible"=w125) -> ()  [unwired: 2 in, 2 out]
                n36 = property on="jog_to_u" class="Bool"("Visible"=w125) -> ()  [unwired: 2 in, 2 out]
              }
              frame "close" {
                w137 = T19[] [] items=["-------------------------", "about", "adjust_goto_buttons", "check_model", "close", "connect", "disable_all", "disable_step_n_loop", "enable_all", "enabled_state_change", "enable_step_n_loop", "exit", "get_device_id", "get_device_name", "get_digital_inputs", "get_digital_outputs", "get_firmware_ver", "get_high_speed", "get_high_speed_global", "get_low_speed", "get_low_speed_global", "get_non_volatile_var", "get_on_fly_speed_mode", "get_polarity", "get_product_id", "get_sspd_mode", "get_step_n_params", "get_volatile_var", "goto_x", "goto_y", "goto_z", "goto_u", "goto_interp", "home_x", "home_y", "home_z", "home_u", "init", "init_ui", "jog_x", "jog_y", "jog_z", "jog_u", "lock", "move_arc", "move_circular", "process_events", "run_standalone", "select_device", "stop_standalone", "set_device_name", "set_digital_outputs", "set_encoder_x", "set_encoder_y", "set_encoder_z", "set_encoder_u", "set_high_speed", "set_low_speed", "set_non_volatile_var", "set_on_fly_position", "set_on_fly_speed", "set_on_fly_speed_mode", "set_polarity", "set_pulse_x", "set_pulse_y", "set_pulse_z", "set_pulse_u", "set_step_n_params", "set_volatile_var", "stop_imm_x", "stop_imm_y", "stop_imm_z", "stop_imm_u", "stop_slow_x", "stop_slow_y", "stop_slow_z", "stop_slow_u", "store_perm", "unlock", "wait_til_idle", "zero_counter", "zero_position"]
                "exit?" <- TRUE ("exit?")
              }
              frame "disable_all" {
                n37 = call-dynamic "setEnabledState.vi"("Controller in"=w138, "error in (no error)"=w141) -> ("Controller out"=w142:refnum<class "_Controller.lvclass">, "error out"=w140:errorcluster)  [unwired: 14 in, 2 out]
              }
              frame "disable_step_n_loop" {
                n38 = local read "step_n_axis"() -> (w144:T8)
                n39 = call-dynamic "disableStepNLoop.vi"("Controller in"=w146, "axis (for multi-axis applications only - otherwise ignored)"=w144, "error in (no error)"=w147) -> ("Controller out"=w145:refnum<class "_Controller.lvclass">, "error out"=w143:errorcluster)  [unwired: 13 in, 2 out]
              }
              frame "enable_all" {
                w149 = TRUE ("x-axis")
                n40 = Bundle By Name(cluster=T21 {"x-axis"=FALSE, "y-axis"=FALSE, "z-axis"=FALSE, "u-axis"=FALSE} ("axes_states (for multi-axis applications only)"), "x-axis"=w149, "y-axis"=w149, "z-axis"=w149, "u-axis"=w149) -> (w151:T21)
                n41 = call-dynamic "setEnabledState.vi"("Controller in"=w156, "axes_states (for multi-axis applications only) - (def = DISABLED)"=w151, "error in (no error)"=w154) -> ("Controller out"=w155:refnum<class "_Controller.lvclass">, "error out"=w153:errorcluster)  [unwired: 13 in, 2 out]
              }
              frame "enabled_state_change" {
                n42 = Bundle By Name(cluster=T21 {"x-axis"=FALSE, "y-axis"=FALSE, "z-axis"=FALSE, "u-axis"=FALSE} ("axes_states (for multi-axis applications only)"), "x-axis"="enabled_x", "y-axis"="enabled_y", "z-axis"="enabled_z", "u-axis"="enabled_u") -> (w162:T21)
                n43 = call-dynamic "setEnabledState.vi"("Controller in"=w167, "axes_states (for multi-axis applications only) - (def = DISABLED)"=w162, "error in (no error)"=w165) -> ("Controller out"=w166:refnum<class "_Controller.lvclass">, "error out"=w164:errorcluster)  [unwired: 13 in, 2 out]
              }
              frame "enable_step_n_loop" {
                n44 = call-dynamic "enableStepNLoop.vi"("Controller in"=w172, "axis (for multi-axis applications only - otherwise ignored)"="step_n_axis", "error in (no error)"=w173) -> ("Controller out"=w170:refnum<class "_Controller.lvclass">, "error out"=w169:errorcluster)  [unwired: 13 in, 2 out]
              }
              frame "get_device_id" {
                n45 = call "getControllerDeviceId.vi"("reference (in)"=w177, "error in (no error)"=w179) -> ("reference (out)"=w176:refnum<class "_Controller.lvclass">, "device_id (out)"=→"dev_id":string, "error out"=w178:errorcluster)  [unwired: 15 in]
              }
              frame "get_device_name" {
                n46 = call "send_receive_command.vi"("reference (in)"=w183, "ASCII Command (in)"="DN", "error in (no error)"=w185) -> ("reference (out)"=w182:refnum<class "_Controller.lvclass">, "response (out)"=→"device_name_to_get" →"dev_name":string, "error out"=w184:errorcluster)  [unwired: 12 in, 2 out]
              }
              frame "get_digital_outputs" {
                n47 = call "getDigitalOutputsStatus.vi"("Controller in"=w193, "get_all? (def=F)"=TRUE, "error in (no error)"=w195) -> ("Controller out"=w192:refnum<class "_Controller.lvclass">, "do_items"=w191:T26[], "error out"=w194:errorcluster)  [unwired: 12 in, 2 out]
                n48 = for {
                  tunnel: w191 -> [w197] mode=indexing
                  tunnel: [w196] -> w190 mode=indexing
                  n49 = Unbundle By Name(w197) -> ("status"=w196:bool)
                }
                n50 = Array To Cluster(array=w190) -> (cluster=w189:T28)
                n51 = local write "dig_outs"(w189) -> ()
              }
              frame "get_firmware_ver" {
                n52 = call "send_receive_command.vi"("reference (in)"=w200, "ASCII Command (in)"="VER", "error in (no error)"=w203) -> ("reference (out)"=w199:refnum<class "_Controller.lvclass">, "response (out)"=→"firmware_ver":string, "error out"=w202:errorcluster)  [unwired: 12 in, 2 out]
              }
              frame "get_high_speed" {
                n53 = for {
                  tunnel: w215 -> [w222]
                  tunnel: w214 -> [w221]
                  tunnel: [w220] -> w213
                  tunnel: [w219] -> w212
                  tunnel: string[] ["HSX", "HSY", "HSZ"] -> [w218] mode=indexing
                  tunnel: [w216] -> w209 mode=indexing
                  n54 = call "send_receive_command.vi"("reference (in)"=w221, "ASCII Command (in)"=w218, "error in (no error)"=w222) -> ("reference (out)"=w220:refnum<class "_Controller.lvclass">, "response (out)"=w217:string, "error out"=w219:errorcluster)  [unwired: 12 in, 2 out]
                  n55 = Decimal String To Number(string=w217) -> (number=w216:i32)  [unwired: 2 in, 1 out]
                }
                n56 = Index Array(array=w209, index #1=0 ("index")) -> (element #1=w208:i32, element #2=w207:i32, element #3=w206:i32)  [unwired: 2 in]
                n57 = local write "X.high_speed"(w208) -> ()
                n58 = local write "Y.high_speed"(w207) -> ()
                n59 = local write "Z.high_speed"(w206) -> ()
              }
              frame "get_high_speed_global" {
                n60 = call "send_receive_command.vi"("reference (in)"=w229, "ASCII Command (in)"="HS", "error in (no error)"=w230) -> ("reference (out)"=w228:refnum<class "_Controller.lvclass">, "response (out)"=w225:string, "error out"=w227:errorcluster)  [unwired: 12 in, 2 out]
                n61 = Decimal String To Number(string=w225) -> (number=w224:i32)  [unwired: 2 in, 1 out]
                n62 = local write "X.high_speed"(w224) -> ()
                n63 = local write "Y.high_speed"(w224) -> ()
                n64 = local write "Z.high_speed"(w224) -> ()
              }
              frame "get_low_speed" {
                n65 = for {
                  tunnel: w241 -> [w248]
                  tunnel: w240 -> [w247]
                  tunnel: [w246] -> w239
                  tunnel: [w245] -> w238
                  tunnel: string[] ["LSX", "LSY", "LSZ"] -> [w244] mode=indexing
                  tunnel: [w242] -> w235 mode=indexing
                  n66 = call "send_receive_command.vi"("reference (in)"=w247, "ASCII Command (in)"=w244, "error in (no error)"=w248) -> ("reference (out)"=w246:refnum<class "_Controller.lvclass">, "response (out)"=w243:string, "error out"=w245:errorcluster)  [unwired: 12 in, 2 out]
                  n67 = Decimal String To Number(string=w243) -> (number=w242:i32)  [unwired: 2 in, 1 out]
                }
                n68 = Index Array(array=w235, index #1=0 ("index")) -> (element #1=w234:i32, element #2=w233:i32, element #3=w232:i32)  [unwired: 2 in]
                n69 = local write "X.low_speed"(w234) -> ()
                n70 = local write "Y.low_speed"(w233) -> ()
                n71 = local write "Z.low_speed"(w232) -> ()
              }
              frame "get_low_speed_global" {
                n72 = call "send_receive_command.vi"("reference (in)"=w255, "ASCII Command (in)"="LS", "error in (no error)"=w256) -> ("reference (out)"=w254:refnum<class "_Controller.lvclass">, "response (out)"=w251:string, "error out"=w253:errorcluster)  [unwired: 12 in, 2 out]
                n73 = Decimal String To Number(string=w251) -> (number=w250:i32)  [unwired: 2 in, 1 out]
                n74 = local write "X.low_speed"(w250) -> ()
                n75 = local write "Y.low_speed"(w250) -> ()
                n76 = local write "Z.low_speed"(w250) -> ()
              }
              frame "get_non_volatile_var", "get_volatile_var" {
                n77 = case shown="\"get_non_volatile_var\"" w258 {
                  tunnel: [w267 w268] -> w259
                  frame "get_volatile_var", Default {
                    n78 = local read "vol_var_num"() -> (w267:u16)
                  }
                  frame "get_non_volatile_var" {
                    n79 = local read "non_vol_var_num"() -> (w268:u16)
                  }
                }
                n80 = call-dynamic "getVariableStatus.vi"("Controller in"=w262, "var_number"=w259, "error in (no error)"=w263) -> ("Controller out"=w261:refnum<class "_Controller.lvclass">, "var_value"=w257:string, "error out"=w260:errorcluster)  [unwired: 14 in]
                n81 = case shown="\"get_non_volatile_var\"" w258 {
                  tunnel: w257 -> [w265 w266]
                  frame "get_volatile_var", Default {
                    "vol_var_read" <- w265
                  }
                  frame "get_non_volatile_var" {
                    "non_vol_var_read" <- w266
                  }
                }
              }
              frame "get_on_fly_speed_mode" {
                n82 = local read "sspd_axis"() -> (w272:T8)
                n83 = Format Into String(format string="SSPDM%s", w272) -> (resulting string=w276:string)  [unwired: 2 in, 1 out]
                n84 = call "send_receive_command.vi"("reference (in)"=w275, "ASCII Command (in)"=w276, "error in (no error)"=w278) -> ("reference (out)"=w274:refnum<class "_Controller.lvclass">, "response (out)"=w271:string, "error out"=w277:errorcluster)  [unwired: 12 in, 2 out]
                n85 = Decimal String To Number(string=w271) -> (number=w269:i32)  [unwired: 2 in, 1 out]
                n86 = To Unsigned Byte Integer(number=w269) -> (unsigned 8bit integer=→"sspd_mode_curr":u8)
              }
              frame "get_polarity" {
                n87 = local read "polarity_axis"() -> (w282:T8)
                n88 = call-dynamic "getPolarity.vi"("Controller in"=w286, "axis (def=X)"=w282, "error in (no error)"=w285) -> ("Controller out"=w284:refnum<class "_Controller.lvclass">, "polarity_items (out)"=→"polarity_out":T15[], "error out"=w283:errorcluster)  [unwired: 14 in]
              }
              frame "get_product_id" {
                n89 = call "send_receive_command.vi"("reference (in)"=w289, "ASCII Command (in)"="ID", "error in (no error)"=w291) -> ("reference (out)"=w288:refnum<class "_Controller.lvclass">, "error out"=w290:errorcluster)  [unwired: 12 in, 3 out]
              }
              frame "get_step_n_params" {
                n90 = local read "step_n_axis"() -> (w299:T8)
                n91 = call-dynamic "getStepNLoopParams.vi"("Controller in"=w303, "axis (only applicable to multi-axis applications)"=w299, "error in (no error)"=w304) -> ("Controller out"=w301:refnum<class "_Controller.lvclass">, "step_n_params"=w298:T29, "error out"=w300:errorcluster)  [unwired: 14 in]
                n92 = Unbundle By Name(w298) -> ("step_N_loop_ratio"=→"step_n_ratio_curr":dbl, "tolerance (encoder counts)"=→"step_n_tolerance_curr":u32, "error_range"=→"step_n_err_range_curr":i32, "max_num_correction_attempts"=→"step_n_max_corr_curr":i32, "enabled?"=w293:bool)
                n93 = local write "enable_disable_step_n"(w293) -> ()
              }
              frame "goto_x".."goto_u" {
                n94 = case shown="\"goto_x\", Default" w309 {
                  tunnel: [T22 {"axis"=enum."X", "target"=0} ("item") T22 {"axis"=enum."Y", "target"=0} ("item") T22 {"axis"=enum."Z", "target"=0} ("item") T22 {"axis"=enum."U", "target"=0} ("item")] -> w308
                  tunnel: [w315 w317 w319 w321] -> w307
                  frame "goto_x", Default {
                    n95 = local read "X.pos_goto"() -> (w315:i32)
                  }
                  frame "goto_y" {
                    n96 = local read "Y.pos_goto"() -> (w317:i32)
                  }
                  frame "goto_z" {
                    n97 = local read "Z.pos_goto"() -> (w319:i32)
                  }
                  frame "goto_u" {
                    n98 = local read "U.pos_goto"() -> (w321:i32)
                  }
                }
                n99 = Bundle By Name(cluster=w308, "target"=w307) -> (w306:T22)
                n100 = Build Array(w306) -> (w305:T22[])
                n101 = call-dynamic "moveToPosition.vi"("Controller in"=w313, "target(s) (in)"=w305, "error in (no error)"=w311) -> ("Controller out"=w312:refnum<class "_Controller.lvclass">, "error out"=w310:errorcluster)  [unwired: 13 in, 2 out]
              }
              frame "goto_interp" {
                n102 = Build Array("X.pos_goto", "Y.pos_goto", "Z.pos_goto", "U.pos_goto") -> (w328:i32[])
                n103 = Build Array("goto_x", "goto_y", "goto_z", "goto_u") -> (w329:bool[])
                n104 = for {
                  shift-right: [w341] -> w326
                  shift-left: T22[] [] ("target(s) (in)") -> [w342]
                  tunnel: w329 -> [w345] mode=indexing
                  tunnel: w328 -> [w344] mode=indexing
                  tunnel: T22[] [{"axis"=enum."X", "target"=0}, {"axis"=enum."Y", "target"=0}, {"axis"=enum."Z", "target"=0}, {"axis"=enum."U", "target"=0}] ("target(s) (in)") -> [w343] mode=indexing
                  n105 = case shown="True" w345 {
                    tunnel: w344 -> [_ w350]
                    tunnel: w343 -> [_ w351]
                    tunnel: w342 -> [w346 w349]
                    tunnel: [w346 w347] -> w341
                    frame False {
                    }
                    frame True {
                      n106 = Bundle By Name(cluster=w351, "target"=w350) -> (w348:T22)
                      n107 = Build Array (concatenate)(w349, w348) -> (w347:T22[])
                    }
                  }
                }
                n108 = call-dynamic "moveToPosition.vi"("Controller in"=w340, "target(s) (in)"=w326, "error in (no error)"=w338) -> ("Controller out"=w339:refnum<class "_Controller.lvclass">, "error out"=w337:errorcluster)  [unwired: 13 in, 2 out]
              }
              frame "home_x".."home_u" {
                n109 = case shown="\"home_x\", Default" w355 {
                  tunnel: [axis."X" ("axis (for multi-axis applications only)") axis."Y" ("axis (for multi-axis applications only)") axis."Z" ("axis (for multi-axis applications only)") axis."U" ("axis (for multi-axis applications only)")] -> w354
                  tunnel: ["home_dir_x" "home_dir_y" "home_dir_z" "home_dir_u"] -> w353
                  tunnel: ["mode_x" "mode_y" "mode_z" "mode_u"] -> w352
                  frame "home_x", Default {
                  }
                  frame "home_y" {
                  }
                  frame "home_z" {
                  }
                  frame "home_u" {
                  }
                }
                n110 = call-dynamic "goToHome.vi"("Controller in"=w358, "axis (for multi-axis applications only)"=w354, "dir"=w353, "mode (for multi-axis applications only)"=w352, "error in (no error)"=w360) -> ("Controller out"=w357:refnum<class "_Controller.lvclass">, "error out"=w359:errorcluster)  [unwired: 11 in, 2 out]
              }
              frame "init", Default {
                w374 = T19[] [enum."init_ui", enum."get_firmware_ver", enum."get_device_id", enum."get_device_name", enum."get_polarity", enum."process_events"] items=["-------------------------", "about", "adjust_goto_buttons", "check_model", "close", "connect", "disable_all", "disable_step_n_loop", "enable_all", "enabled_state_change", "enable_step_n_loop", "exit", "get_device_id", "get_device_name", "get_digital_inputs", "get_digital_outputs", "get_firmware_ver", "get_high_speed", "get_high_speed_global", "get_low_speed", "get_low_speed_global", "get_non_volatile_var", "get_on_fly_speed_mode", "get_polarity", "get_product_id", "get_sspd_mode", "get_step_n_params", "get_volatile_var", "goto_x", "goto_y", "goto_z", "goto_u", "goto_interp", "home_x", "home_y", "home_z", "home_u", "init", "init_ui", "jog_x", "jog_y", "jog_z", "jog_u", "lock", "move_arc", "move_circular", "process_events", "run_standalone", "select_device", "stop_standalone", "set_device_name", "set_digital_outputs", "set_encoder_x", "set_encoder_y", "set_encoder_z", "set_encoder_u", "set_high_speed", "set_low_speed", "set_non_volatile_var", "set_on_fly_position", "set_on_fly_speed", "set_on_fly_speed_mode", "set_polarity", "set_pulse_x", "set_pulse_y", "set_pulse_z", "set_pulse_u", "set_step_n_params", "set_volatile_var", "stop_imm_x", "stop_imm_y", "stop_imm_z", "stop_imm_u", "stop_slow_x", "stop_slow_y", "stop_slow_z", "stop_slow_u", "store_perm", "unlock", "wait_til_idle", "zero_counter", "zero_position"]
              }
              frame "init_ui" {
                w381 = T19[] [enum."enabled_state_change", enum."adjust_goto_buttons"] items=["-------------------------", "about", "adjust_goto_buttons", "check_model", "close", "connect", "disable_all", "disable_step_n_loop", "enable_all", "enabled_state_change", "enable_step_n_loop", "exit", "get_device_id", "get_device_name", "get_digital_inputs", "get_digital_outputs", "get_firmware_ver", "get_high_speed", "get_high_speed_global", "get_low_speed", "get_low_speed_global", "get_non_volatile_var", "get_on_fly_speed_mode", "get_polarity", "get_product_id", "get_sspd_mode", "get_step_n_params", "get_volatile_var", "goto_x", "goto_y", "goto_z", "goto_u", "goto_interp", "home_x", "home_y", "home_z", "home_u", "init", "init_ui", "jog_x", "jog_y", "jog_z", "jog_u", "lock", "move_arc", "move_circular", "process_events", "run_standalone", "select_device", "stop_standalone", "set_device_name", "set_digital_outputs", "set_encoder_x", "set_encoder_y", "set_encoder_z", "set_encoder_u", "set_high_speed", "set_low_speed", "set_non_volatile_var", "set_on_fly_position", "set_on_fly_speed", "set_on_fly_speed_mode", "set_polarity", "set_pulse_x", "set_pulse_y", "set_pulse_z", "set_pulse_u", "set_step_n_params", "set_volatile_var", "stop_imm_x", "stop_imm_y", "stop_imm_z", "stop_imm_u", "stop_slow_x", "stop_slow_y", "stop_slow_z", "stop_slow_u", "store_perm", "unlock", "wait_til_idle", "zero_counter", "zero_position"]
                w376 = FALSE ("enabled_x")
                n111 = local write "enabled_x"(w376) -> ()
                n112 = local write "enabled_y"(w376) -> ()
                n113 = local write "enabled_z"(w376) -> ()
                n114 = local write "enabled_u"(w376) -> ()
                n115 = local write "goto_x"(w376) -> ()
                n116 = local write "goto_y"(w376) -> ()
                n117 = local write "goto_z"(w376) -> ()
                n118 = local write "goto_u"(w376) -> ()
                n119 = property on="goto_interp" class="Bool"("Visible"=w376) -> ()  [unwired: 2 in, 2 out]
                n120 = property on="Tab Control" class="TabCtl (strict)"("DisabledEnum"=T23."Enabled" ("Disabled"), "Value"=T3."Motion Control (Basic) " ("Tab Control")) -> ()  [unwired: 2 in, 2 out]
                n121 = Build Array (concatenate)(w381, w380) -> (w379:T19[])
              }
              frame "jog_x".."jog_u" {
                n122 = case shown="\"jog_x\", Default" w386 {
                  tunnel: [axis."X" ("axis (for multi-axis applications only)") axis."Y" ("axis (for multi-axis applications only)") axis."Z" ("axis (for multi-axis applications only)") axis."U" ("axis (for multi-axis applications only)")] -> w385
                  tunnel: ["jog_dir_x" "jog_dir_y" "jog_dir_z" "jog_dir_u"] -> w384
                  frame "jog_x", Default {
                  }
                  frame "jog_y" {
                  }
                  frame "jog_z" {
                  }
                  frame "jog_u" {
                  }
                }
                n123 = call-dynamic "jogMotor.vi"("Controller in"=w389, "axis (for multi-axis applications only)"=w385, "dir"=w384, "error in (no error)"=w391) -> ("Controller out"=w388:refnum<class "_Controller.lvclass">, "error out"=w390:errorcluster)  [unwired: 12 in, 2 out]
              }
              frame "move_arc" {
                n124 = To More Specific Class(target class=refnum<class "_MultiAxisController.lvclass"> refnum ("classes.lvlib:_MultiAxisController.lvclass"), reference=w411, error in=w412) -> (specific class reference=w408:refnum<class "_MultiAxisController.lvclass">, error out=w409:errorcluster)
                n125 = call-dynamic "moveArc.vi"("MultiAxisController in"=w408, "x_coord"="x_coord - arc", "y_coord"="y_coord - arc", "direction"="direction - arc", "error in (no error)"=w409, "absolute_angle (degrees)"="absolute_angle (degrees) - arc", "relative_angle (degrees)"="relative_angle (degrees) - arc") -> ("MultiAxisController out"=w407:refnum<class "_MultiAxisController.lvclass">, "error out"=w405:errorcluster)  [unwired: 9 in, 2 out]
              }
              frame "move_circular" {
                n126 = To More Specific Class(target class=refnum<class "_MultiAxisController.lvclass"> refnum ("classes.lvlib:_MultiAxisController.lvclass"), reference=w422, error in=w423) -> (specific class reference=w419:refnum<class "_MultiAxisController.lvclass">, error out=w420:errorcluster)
                n127 = call-dynamic "moveCircular.vi"("MultiAxisController in"=w419, "x_coord"="x_coord - circle", "y_coord"="y_coord - circle", "direction"="direction - circle", "error in (no error)"=w420) -> ("MultiAxisController out"=w418:refnum<class "_MultiAxisController.lvclass">, "error out"=w416:errorcluster)  [unwired: 11 in, 2 out]
              }
              frame "process_events" {
                n128 = event shown="[52] Menu Selection (User)" {
                  selector: _ -> [_ _ _ _ _ _ _ _ _ _ _ _ _ _ _ _ _ _ _ _ _ _ _ _ _ _ _ _ _ _ _ _ _ _ _ _ _ _ _ _ _ _ _ _ _ _ _ _ _ _ _ _ _]
                  dyn-events: _ -> [_ _ _ _ _ _ _ _ _ _ _ _ _ _ _ _ _ _ _ _ _ _ _ _ _ _ _ _ _ _ _ _ _ _ _ _ _ _ _ _ _ _ _ _ _ _ _ _ _ _ _ _ _]
                  timeout: _ -> [_ _ _ _ _ _ _ _ _ _ _ _ _ _ _ _ _ _ _ _ _ _ _ _ _ _ _ _ _ _ _ _ _ _ _ _ _ _ _ _ _ _ _ _ _ _ _ _ _ _ _ _ _]
                  tunnel: w427 -> [w429 w431 w433 w435 w437 w439 w441 w443 w445 w447 w449 w451 w453 w455 w457 w459 w461 w463 w465 w467 w469 w471 w473 w475 w477 w479 w481 w483 w485 w487 w489 w491 w493 w495 w497 w499 w501 w503 w505 w507 w509 w511 w514 w519 w531 w536 w538 w540 w542 w544 w546 w548 w554]
                  tunnel: [w430 w432 w434 w436 w438 w440 w442 w444 w446 w448 w450 w452 w454 w456 w458 w460 w462 w464 w466 w468 w470 w472 w474 w476 w478 w480 w482 w484 w486 w488 w490 w492 w494 w496 w498 w500 w502 w504 w506 w508 w510 w512 w515 w520 w532 w537 w539 w541 w543 w545 w547 w549 w550] -> w426
                  tunnel: w425 -> [w430 _ _ _ _ _ _ _ _ _ _ _ _ _ _ _ _ _ _ _ _ _ _ _ _ _ _ _ _ _ _ _ _ _ _ _ _ _ _ _ _ _ _ _ _ _ _ _ _ _ _ _ _]
                  tunnel: [w429 w431 w433 w435 w437 w439 w441 w443 w445 w447 w449 w451 w453 w455 w457 w459 w461 w463 w465 w467 w469 w471 w473 w475 w477 w479 w481 w483 w485 w487 w489 w491 w493 w495 w497 w499 w501 w503 w505 w507 w509 w511 w514 w519 w531 w536 w538 w540 w542 w544 w546 w548 w553] -> w424
                  event Timeout {
                    n129 = event-data() -> ()  [unwired: 1 in, 3 out]
                  }
                  event "set_speeds": Value Change {
                    w432 = T19[] [enum."set_low_speed", enum."set_high_speed", enum."process_events"] items=["-------------------------", "about", "adjust_goto_buttons", "check_model", "close", "connect", "disable_all", "disable_step_n_loop", "enable_all", "enabled_state_change", "enable_step_n_loop", "exit", "get_device_id", "get_device_name", "get_digital_inputs", "get_digital_outputs", "get_firmware_ver", "get_high_speed", "get_high_speed_global", "get_low_speed", "get_low_speed_global", "get_non_volatile_var", "get_on_fly_speed_mode", "get_polarity", "get_product_id", "get_sspd_mode", "get_step_n_params", "get_volatile_var", "goto_x", "goto_y", "goto_z", "goto_u", "goto_interp", "home_x", "home_y", "home_z", "home_u", "init", "init_ui", "jog_x", "jog_y", "jog_z", "jog_u", "lock", "move_arc", "move_circular", "process_events", "run_standalone", "select_device", "stop_standalone", "set_device_name", "set_digital_outputs", "set_encoder_x", "set_encoder_y", "set_encoder_z", "set_encoder_u", "set_high_speed", "set_low_speed", "set_non_volatile_var", "set_on_fly_position", "set_on_fly_speed", "set_on_fly_speed_mode", "set_polarity", "set_pulse_x", "set_pulse_y", "set_pulse_z", "set_pulse_u", "set_step_n_params", "set_volatile_var", "stop_imm_x", "stop_imm_y", "stop_imm_z", "stop_imm_u", "stop_slow_x", "stop_slow_y", "stop_slow_z", "stop_slow_u", "store_perm", "unlock", "wait_til_idle", "zero_counter", "zero_position"]
                    n130 = event-data() -> ()  [unwired: 1 in, 6 out]
                  }
                  event "reset_pos": Value Change {
                    w434 = T19[] [enum."zero_position", enum."process_events"] items=["-------------------------", "about", "adjust_goto_buttons", "check_model", "close", "connect", "disable_all", "disable_step_n_loop", "enable_all", "enabled_state_change", "enable_step_n_loop", "exit", "get_device_id", "get_device_name", "get_digital_inputs", "get_digital_outputs", "get_firmware_ver", "get_high_speed", "get_high_speed_global", "get_low_speed", "get_low_speed_global", "get_non_volatile_var", "get_on_fly_speed_mode", "get_polarity", "get_product_id", "get_sspd_mode", "get_step_n_params", "get_volatile_var", "goto_x", "goto_y", "goto_z", "goto_u", "goto_interp", "home_x", "home_y", "home_z", "home_u", "init", "init_ui", "jog_x", "jog_y", "jog_z", "jog_u", "lock", "move_arc", "move_circular", "process_events", "run_standalone", "select_device", "stop_standalone", "set_device_name", "set_digital_outputs", "set_encoder_x", "set_encoder_y", "set_encoder_z", "set_encoder_u", "set_high_speed", "set_low_speed", "set_non_volatile_var", "set_on_fly_position", "set_on_fly_speed", "set_on_fly_speed_mode", "set_polarity", "set_pulse_x", "set_pulse_y", "set_pulse_z", "set_pulse_u", "set_step_n_params", "set_volatile_var", "stop_imm_x", "stop_imm_y", "stop_imm_z", "stop_imm_u", "stop_slow_x", "stop_slow_y", "stop_slow_z", "stop_slow_u", "store_perm", "unlock", "wait_til_idle", "zero_counter", "zero_position"]
                    n131 = event-data() -> ()  [unwired: 1 in, 6 out]
                  }
                  event "exit": Value Change {
                    w436 = T19[] [enum."disable_all", enum."close"] items=["-------------------------", "about", "adjust_goto_buttons", "check_model", "close", "connect", "disable_all", "disable_step_n_loop", "enable_all", "enabled_state_change", "enable_step_n_loop", "exit", "get_device_id", "get_device_name", "get_digital_inputs", "get_digital_outputs", "get_firmware_ver", "get_high_speed", "get_high_speed_global", "get_low_speed", "get_low_speed_global", "get_non_volatile_var", "get_on_fly_speed_mode", "get_polarity", "get_product_id", "get_sspd_mode", "get_step_n_params", "get_volatile_var", "goto_x", "goto_y", "goto_z", "goto_u", "goto_interp", "home_x", "home_y", "home_z", "home_u", "init", "init_ui", "jog_x", "jog_y", "jog_z", "jog_u", "lock", "move_arc", "move_circular", "process_events", "run_standalone", "select_device", "stop_standalone", "set_device_name", "set_digital_outputs", "set_encoder_x", "set_encoder_y", "set_encoder_z", "set_encoder_u", "set_high_speed", "set_low_speed", "set_non_volatile_var", "set_on_fly_position", "set_on_fly_speed", "set_on_fly_speed_mode", "set_polarity", "set_pulse_x", "set_pulse_y", "set_pulse_z", "set_pulse_u", "set_step_n_params", "set_volatile_var", "stop_imm_x", "stop_imm_y", "stop_imm_z", "stop_imm_u", "stop_slow_x", "stop_slow_y", "stop_slow_z", "stop_slow_u", "store_perm", "unlock", "wait_til_idle", "zero_counter", "zero_position"]
                    n132 = event-data() -> ()  [unwired: 1 in, 6 out]
                  }
                  event Value Change {
                    w438 = T19[] [enum."goto_x", enum."process_events"] items=["-------------------------", "about", "adjust_goto_buttons", "check_model", "close", "connect", "disable_all", "disable_step_n_loop", "enable_all", "enabled_state_change", "enable_step_n_loop", "exit", "get_device_id", "get_device_name", "get_digital_inputs", "get_digital_outputs", "get_firmware_ver", "get_high_speed", "get_high_speed_global", "get_low_speed", "get_low_speed_global", "get_non_volatile_var", "get_on_fly_speed_mode", "get_polarity", "get_product_id", "get_sspd_mode", "get_step_n_params", "get_volatile_var", "goto_x", "goto_y", "goto_z", "goto_u", "goto_interp", "home_x", "home_y", "home_z", "home_u", "init", "init_ui", "jog_x", "jog_y", "jog_z", "jog_u", "lock", "move_arc", "move_circular", "process_events", "run_standalone", "select_device", "stop_standalone", "set_device_name", "set_digital_outputs", "set_encoder_x", "set_encoder_y", "set_encoder_z", "set_encoder_u", "set_high_speed", "set_low_speed", "set_non_volatile_var", "set_on_fly_position", "set_on_fly_speed", "set_on_fly_speed_mode", "set_polarity", "set_pulse_x", "set_pulse_y", "set_pulse_z", "set_pulse_u", "set_step_n_params", "set_volatile_var", "stop_imm_x", "stop_imm_y", "stop_imm_z", "stop_imm_u", "stop_slow_x", "stop_slow_y", "stop_slow_z", "stop_slow_u", "store_perm", "unlock", "wait_til_idle", "zero_counter", "zero_position"]
                    n133 = event-data() -> ()  [unwired: 1 in, 6 out]
                  }
                  event "enabled_x", "enabled_y", "enabled_z", "enabled_u": Value Change {
                    w440 = T19[] [enum."enabled_state_change", enum."process_events"] items=["-------------------------", "about", "adjust_goto_buttons", "check_model", "close", "connect", "disable_all", "disable_step_n_loop", "enable_all", "enabled_state_change", "enable_step_n_loop", "exit", "get_device_id", "get_device_name", "get_digital_inputs", "get_digital_outputs", "get_firmware_ver", "get_high_speed", "get_high_speed_global", "get_low_speed", "get_low_speed_global", "get_non_volatile_var", "get_on_fly_speed_mode", "get_polarity", "get_product_id", "get_sspd_mode", "get_step_n_params", "get_volatile_var", "goto_x", "goto_y", "goto_z", "goto_u", "goto_interp", "home_x", "home_y", "home_z", "home_u", "init", "init_ui", "jog_x", "jog_y", "jog_z", "jog_u", "lock", "move_arc", "move_circular", "process_events", "run_standalone", "select_device", "stop_standalone", "set_device_name", "set_digital_outputs", "set_encoder_x", "set_encoder_y", "set_encoder_z", "set_encoder_u", "set_high_speed", "set_low_speed", "set_non_volatile_var", "set_on_fly_position", "set_on_fly_speed", "set_on_fly_speed_mode", "set_polarity", "set_pulse_x", "set_pulse_y", "set_pulse_z", "set_pulse_u", "set_step_n_params", "set_volatile_var", "stop_imm_x", "stop_imm_y", "stop_imm_z", "stop_imm_u", "stop_slow_x", "stop_slow_y", "stop_slow_z", "stop_slow_u", "store_perm", "unlock", "wait_til_idle", "zero_counter", "zero_position"]
                    n134 = event-data() -> ()  [unwired: 1 in, 6 out]
                  }
                  event "set_vol_var": Value Change {
                    w442 = T19[] [enum."set_volatile_var", enum."process_events"] items=["-------------------------", "about", "adjust_goto_buttons", "check_model", "close", "connect", "disable_all", "disable_step_n_loop", "enable_all", "enabled_state_change", "enable_step_n_loop", "exit", "get_device_id", "get_device_name", "get_digital_inputs", "get_digital_outputs", "get_firmware_ver", "get_high_speed", "get_high_speed_global", "get_low_speed", "get_low_speed_global", "get_non_volatile_var", "get_on_fly_speed_mode", "get_polarity", "get_product_id", "get_sspd_mode", "get_step_n_params", "get_volatile_var", "goto_x", "goto_y", "goto_z", "goto_u", "goto_interp", "home_x", "home_y", "home_z", "home_u", "init", "init_ui", "jog_x", "jog_y", "jog_z", "jog_u", "lock", "move_arc", "move_circular", "process_events", "run_standalone", "select_device", "stop_standalone", "set_device_name", "set_digital_outputs", "set_encoder_x", "set_encoder_y", "set_encoder_z", "set_encoder_u", "set_high_speed", "set_low_speed", "set_non_volatile_var", "set_on_fly_position", "set_on_fly_speed", "set_on_fly_speed_mode", "set_polarity", "set_pulse_x", "set_pulse_y", "set_pulse_z", "set_pulse_u", "set_step_n_params", "set_volatile_var", "stop_imm_x", "stop_imm_y", "stop_imm_z", "stop_imm_u", "stop_slow_x", "stop_slow_y", "stop_slow_z", "stop_slow_u", "store_perm", "unlock", "wait_til_idle", "zero_counter", "zero_position"]
                    n135 = event-data() -> ()  [unwired: 1 in, 6 out]
                  }
                  event "set_non_vol_var": Value Change {
                    w444 = T19[] [enum."set_non_volatile_var", enum."store_perm", enum."process_events"] items=["-------------------------", "about", "adjust_goto_buttons", "check_model", "close", "connect", "disable_all", "disable_step_n_loop", "enable_all", "enabled_state_change", "enable_step_n_loop", "exit", "get_device_id", "get_device_name", "get_digital_inputs", "get_digital_outputs", "get_firmware_ver", "get_high_speed", "get_high_speed_global", "get_low_speed", "get_low_speed_global", "get_non_volatile_var", "get_on_fly_speed_mode", "get_polarity", "get_product_id", "get_sspd_mode", "get_step_n_params", "get_volatile_var", "goto_x", "goto_y", "goto_z", "goto_u", "goto_interp", "home_x", "home_y", "home_z", "home_u", "init", "init_ui", "jog_x", "jog_y", "jog_z", "jog_u", "lock", "move_arc", "move_circular", "process_events", "run_standalone", "select_device", "stop_standalone", "set_device_name", "set_digital_outputs", "set_encoder_x", "set_encoder_y", "set_encoder_z", "set_encoder_u", "set_high_speed", "set_low_speed", "set_non_volatile_var", "set_on_fly_position", "set_on_fly_speed", "set_on_fly_speed_mode", "set_polarity", "set_pulse_x", "set_pulse_y", "set_pulse_z", "set_pulse_u", "set_step_n_params", "set_volatile_var", "stop_imm_x", "stop_imm_y", "stop_imm_z", "stop_imm_u", "stop_slow_x", "stop_slow_y", "stop_slow_z", "stop_slow_u", "store_perm", "unlock", "wait_til_idle", "zero_counter", "zero_position"]
                    n136 = event-data() -> ()  [unwired: 1 in, 6 out]
                  }
                  event "get_non_vol_var": Value Change {
                    w446 = T19[] [enum."get_non_volatile_var", enum."process_events"] items=["-------------------------", "about", "adjust_goto_buttons", "check_model", "close", "connect", "disable_all", "disable_step_n_loop", "enable_all", "enabled_state_change", "enable_step_n_loop", "exit", "get_device_id", "get_device_name", "get_digital_inputs", "get_digital_outputs", "get_firmware_ver", "get_high_speed", "get_high_speed_global", "get_low_speed", "get_low_speed_global", "get_non_volatile_var", "get_on_fly_speed_mode", "get_polarity", "get_product_id", "get_sspd_mode", "get_step_n_params", "get_volatile_var", "goto_x", "goto_y", "goto_z", "goto_u", "goto_interp", "home_x", "home_y", "home_z", "home_u", "init", "init_ui", "jog_x", "jog_y", "jog_z", "jog_u", "lock", "move_arc", "move_circular", "process_events", "run_standalone", "select_device", "stop_standalone", "set_device_name", "set_digital_outputs", "set_encoder_x", "set_encoder_y", "set_encoder_z", "set_encoder_u", "set_high_speed", "set_low_speed", "set_non_volatile_var", "set_on_fly_position", "set_on_fly_speed", "set_on_fly_speed_mode", "set_polarity", "set_pulse_x", "set_pulse_y", "set_pulse_z", "set_pulse_u", "set_step_n_params", "set_volatile_var", "stop_imm_x", "stop_imm_y", "stop_imm_z", "stop_imm_u", "stop_slow_x", "stop_slow_y", "stop_slow_z", "stop_slow_u", "store_perm", "unlock", "wait_til_idle", "zero_counter", "zero_position"]
                    n137 = event-data() -> ()  [unwired: 1 in, 6 out]
                  }
                  event "get_vol_var": Value Change {
                    w448 = T19[] [enum."get_volatile_var", enum."process_events"] items=["-------------------------", "about", "adjust_goto_buttons", "check_model", "close", "connect", "disable_all", "disable_step_n_loop", "enable_all", "enabled_state_change", "enable_step_n_loop", "exit", "get_device_id", "get_device_name", "get_digital_inputs", "get_digital_outputs", "get_firmware_ver", "get_high_speed", "get_high_speed_global", "get_low_speed", "get_low_speed_global", "get_non_volatile_var", "get_on_fly_speed_mode", "get_polarity", "get_product_id", "get_sspd_mode", "get_step_n_params", "get_volatile_var", "goto_x", "goto_y", "goto_z", "goto_u", "goto_interp", "home_x", "home_y", "home_z", "home_u", "init", "init_ui", "jog_x", "jog_y", "jog_z", "jog_u", "lock", "move_arc", "move_circular", "process_events", "run_standalone", "select_device", "stop_standalone", "set_device_name", "set_digital_outputs", "set_encoder_x", "set_encoder_y", "set_encoder_z", "set_encoder_u", "set_high_speed", "set_low_speed", "set_non_volatile_var", "set_on_fly_position", "set_on_fly_speed", "set_on_fly_speed_mode", "set_polarity", "set_pulse_x", "set_pulse_y", "set_pulse_z", "set_pulse_u", "set_step_n_params", "set_volatile_var", "stop_imm_x", "stop_imm_y", "stop_imm_z", "stop_imm_u", "stop_slow_x", "stop_slow_y", "stop_slow_z", "stop_slow_u", "store_perm", "unlock", "wait_til_idle", "zero_counter", "zero_position"]
                    n138 = event-data() -> ()  [unwired: 1 in, 6 out]
                  }
                  event Value Change {
                    w450 = T19[] [enum."goto_y", enum."process_events"] items=["-------------------------", "about", "adjust_goto_buttons", "check_model", "close", "connect", "disable_all", "disable_step_n_loop", "enable_all", "enabled_state_change", "enable_step_n_loop", "exit", "get_device_id", "get_device_name", "get_digital_inputs", "get_digital_outputs", "get_firmware_ver", "get_high_speed", "get_high_speed_global", "get_low_speed", "get_low_speed_global", "get_non_volatile_var", "get_on_fly_speed_mode", "get_polarity", "get_product_id", "get_sspd_mode", "get_step_n_params", "get_volatile_var", "goto_x", "goto_y", "goto_z", "goto_u", "goto_interp", "home_x", "home_y", "home_z", "home_u", "init", "init_ui", "jog_x", "jog_y", "jog_z", "jog_u", "lock", "move_arc", "move_circular", "process_events", "run_standalone", "select_device", "stop_standalone", "set_device_name", "set_digital_outputs", "set_encoder_x", "set_encoder_y", "set_encoder_z", "set_encoder_u", "set_high_speed", "set_low_speed", "set_non_volatile_var", "set_on_fly_position", "set_on_fly_speed", "set_on_fly_speed_mode", "set_polarity", "set_pulse_x", "set_pulse_y", "set_pulse_z", "set_pulse_u", "set_step_n_params", "set_volatile_var", "stop_imm_x", "stop_imm_y", "stop_imm_z", "stop_imm_u", "stop_slow_x", "stop_slow_y", "stop_slow_z", "stop_slow_u", "store_perm", "unlock", "wait_til_idle", "zero_counter", "zero_position"]
                    n139 = event-data() -> ()  [unwired: 1 in, 6 out]
                  }
                  event Value Change {
                    w452 = T19[] [enum."goto_z", enum."process_events"] items=["-------------------------", "about", "adjust_goto_buttons", "check_model", "close", "connect", "disable_all", "disable_step_n_loop", "enable_all", "enabled_state_change", "enable_step_n_loop", "exit", "get_device_id", "get_device_name", "get_digital_inputs", "get_digital_outputs", "get_firmware_ver", "get_high_speed", "get_high_speed_global", "get_low_speed", "get_low_speed_global", "get_non_volatile_var", "get_on_fly_speed_mode", "get_polarity", "get_product_id", "get_sspd_mode", "get_step_n_params", "get_volatile_var", "goto_x", "goto_y", "goto_z", "goto_u", "goto_interp", "home_x", "home_y", "home_z", "home_u", "init", "init_ui", "jog_x", "jog_y", "jog_z", "jog_u", "lock", "move_arc", "move_circular", "process_events", "run_standalone", "select_device", "stop_standalone", "set_device_name", "set_digital_outputs", "set_encoder_x", "set_encoder_y", "set_encoder_z", "set_encoder_u", "set_high_speed", "set_low_speed", "set_non_volatile_var", "set_on_fly_position", "set_on_fly_speed", "set_on_fly_speed_mode", "set_polarity", "set_pulse_x", "set_pulse_y", "set_pulse_z", "set_pulse_u", "set_step_n_params", "set_volatile_var", "stop_imm_x", "stop_imm_y", "stop_imm_z", "stop_imm_u", "stop_slow_x", "stop_slow_y", "stop_slow_z", "stop_slow_u", "store_perm", "unlock", "wait_til_idle", "zero_counter", "zero_position"]
                    n140 = event-data() -> ()  [unwired: 1 in, 6 out]
                  }
                  event Value Change {
                    w454 = T19[] [enum."goto_u", enum."process_events"] items=["-------------------------", "about", "adjust_goto_buttons", "check_model", "close", "connect", "disable_all", "disable_step_n_loop", "enable_all", "enabled_state_change", "enable_step_n_loop", "exit", "get_device_id", "get_device_name", "get_digital_inputs", "get_digital_outputs", "get_firmware_ver", "get_high_speed", "get_high_speed_global", "get_low_speed", "get_low_speed_global", "get_non_volatile_var", "get_on_fly_speed_mode", "get_polarity", "get_product_id", "get_sspd_mode", "get_step_n_params", "get_volatile_var", "goto_x", "goto_y", "goto_z", "goto_u", "goto_interp", "home_x", "home_y", "home_z", "home_u", "init", "init_ui", "jog_x", "jog_y", "jog_z", "jog_u", "lock", "move_arc", "move_circular", "process_events", "run_standalone", "select_device", "stop_standalone", "set_device_name", "set_digital_outputs", "set_encoder_x", "set_encoder_y", "set_encoder_z", "set_encoder_u", "set_high_speed", "set_low_speed", "set_non_volatile_var", "set_on_fly_position", "set_on_fly_speed", "set_on_fly_speed_mode", "set_polarity", "set_pulse_x", "set_pulse_y", "set_pulse_z", "set_pulse_u", "set_step_n_params", "set_volatile_var", "stop_imm_x", "stop_imm_y", "stop_imm_z", "stop_imm_u", "stop_slow_x", "stop_slow_y", "stop_slow_z", "stop_slow_u", "store_perm", "unlock", "wait_til_idle", "zero_counter", "zero_position"]
                    n141 = event-data() -> ()  [unwired: 1 in, 6 out]
                  }
                  event Value Change {
                    w456 = T19[] [enum."jog_x", enum."process_events"] items=["-------------------------", "about", "adjust_goto_buttons", "check_model", "close", "connect", "disable_all", "disable_step_n_loop", "enable_all", "enabled_state_change", "enable_step_n_loop", "exit", "get_device_id", "get_device_name", "get_digital_inputs", "get_digital_outputs", "get_firmware_ver", "get_high_speed", "get_high_speed_global", "get_low_speed", "get_low_speed_global", "get_non_volatile_var", "get_on_fly_speed_mode", "get_polarity", "get_product_id", "get_sspd_mode", "get_step_n_params", "get_volatile_var", "goto_x", "goto_y", "goto_z", "goto_u", "goto_interp", "home_x", "home_y", "home_z", "home_u", "init", "init_ui", "jog_x", "jog_y", "jog_z", "jog_u", "lock", "move_arc", "move_circular", "process_events", "run_standalone", "select_device", "stop_standalone", "set_device_name", "set_digital_outputs", "set_encoder_x", "set_encoder_y", "set_encoder_z", "set_encoder_u", "set_high_speed", "set_low_speed", "set_non_volatile_var", "set_on_fly_position", "set_on_fly_speed", "set_on_fly_speed_mode", "set_polarity", "set_pulse_x", "set_pulse_y", "set_pulse_z", "set_pulse_u", "set_step_n_params", "set_volatile_var", "stop_imm_x", "stop_imm_y", "stop_imm_z", "stop_imm_u", "stop_slow_x", "stop_slow_y", "stop_slow_z", "stop_slow_u", "store_perm", "unlock", "wait_til_idle", "zero_counter", "zero_position"]
                    n142 = event-data() -> ()  [unwired: 1 in, 6 out]
                  }
                  event Value Change {
                    w458 = T19[] [enum."jog_y", enum."process_events"] items=["-------------------------", "about", "adjust_goto_buttons", "check_model", "close", "connect", "disable_all", "disable_step_n_loop", "enable_all", "enabled_state_change", "enable_step_n_loop", "exit", "get_device_id", "get_device_name", "get_digital_inputs", "get_digital_outputs", "get_firmware_ver", "get_high_speed", "get_high_speed_global", "get_low_speed", "get_low_speed_global", "get_non_volatile_var", "get_on_fly_speed_mode", "get_polarity", "get_product_id", "get_sspd_mode", "get_step_n_params", "get_volatile_var", "goto_x", "goto_y", "goto_z", "goto_u", "goto_interp", "home_x", "home_y", "home_z", "home_u", "init", "init_ui", "jog_x", "jog_y", "jog_z", "jog_u", "lock", "move_arc", "move_circular", "process_events", "run_standalone", "select_device", "stop_standalone", "set_device_name", "set_digital_outputs", "set_encoder_x", "set_encoder_y", "set_encoder_z", "set_encoder_u", "set_high_speed", "set_low_speed", "set_non_volatile_var", "set_on_fly_position", "set_on_fly_speed", "set_on_fly_speed_mode", "set_polarity", "set_pulse_x", "set_pulse_y", "set_pulse_z", "set_pulse_u", "set_step_n_params", "set_volatile_var", "stop_imm_x", "stop_imm_y", "stop_imm_z", "stop_imm_u", "stop_slow_x", "stop_slow_y", "stop_slow_z", "stop_slow_u", "store_perm", "unlock", "wait_til_idle", "zero_counter", "zero_position"]
                    n143 = event-data() -> ()  [unwired: 1 in, 6 out]
                  }
                  event Value Change {
                    w460 = T19[] [enum."jog_z", enum."process_events"] items=["-------------------------", "about", "adjust_goto_buttons", "check_model", "close", "connect", "disable_all", "disable_step_n_loop", "enable_all", "enabled_state_change", "enable_step_n_loop", "exit", "get_device_id", "get_device_name", "get_digital_inputs", "get_digital_outputs", "get_firmware_ver", "get_high_speed", "get_high_speed_global", "get_low_speed", "get_low_speed_global", "get_non_volatile_var", "get_on_fly_speed_mode", "get_polarity", "get_product_id", "get_sspd_mode", "get_step_n_params", "get_volatile_var", "goto_x", "goto_y", "goto_z", "goto_u", "goto_interp", "home_x", "home_y", "home_z", "home_u", "init", "init_ui", "jog_x", "jog_y", "jog_z", "jog_u", "lock", "move_arc", "move_circular", "process_events", "run_standalone", "select_device", "stop_standalone", "set_device_name", "set_digital_outputs", "set_encoder_x", "set_encoder_y", "set_encoder_z", "set_encoder_u", "set_high_speed", "set_low_speed", "set_non_volatile_var", "set_on_fly_position", "set_on_fly_speed", "set_on_fly_speed_mode", "set_polarity", "set_pulse_x", "set_pulse_y", "set_pulse_z", "set_pulse_u", "set_step_n_params", "set_volatile_var", "stop_imm_x", "stop_imm_y", "stop_imm_z", "stop_imm_u", "stop_slow_x", "stop_slow_y", "stop_slow_z", "stop_slow_u", "store_perm", "unlock", "wait_til_idle", "zero_counter", "zero_position"]
                    n144 = event-data() -> ()  [unwired: 1 in, 6 out]
                  }
                  event Value Change {
                    w462 = T19[] [enum."jog_u", enum."process_events"] items=["-------------------------", "about", "adjust_goto_buttons", "check_model", "close", "connect", "disable_all", "disable_step_n_loop", "enable_all", "enabled_state_change", "enable_step_n_loop", "exit", "get_device_id", "get_device_name", "get_digital_inputs", "get_digital_outputs", "get_firmware_ver", "get_high_speed", "get_high_speed_global", "get_low_speed", "get_low_speed_global", "get_non_volatile_var", "get_on_fly_speed_mode", "get_polarity", "get_product_id", "get_sspd_mode", "get_step_n_params", "get_volatile_var", "goto_x", "goto_y", "goto_z", "goto_u", "goto_interp", "home_x", "home_y", "home_z", "home_u", "init", "init_ui", "jog_x", "jog_y", "jog_z", "jog_u", "lock", "move_arc", "move_circular", "process_events", "run_standalone", "select_device", "stop_standalone", "set_device_name", "set_digital_outputs", "set_encoder_x", "set_encoder_y", "set_encoder_z", "set_encoder_u", "set_high_speed", "set_low_speed", "set_non_volatile_var", "set_on_fly_position", "set_on_fly_speed", "set_on_fly_speed_mode", "set_polarity", "set_pulse_x", "set_pulse_y", "set_pulse_z", "set_pulse_u", "set_step_n_params", "set_volatile_var", "stop_imm_x", "stop_imm_y", "stop_imm_z", "stop_imm_u", "stop_slow_x", "stop_slow_y", "stop_slow_z", "stop_slow_u", "store_perm", "unlock", "wait_til_idle", "zero_counter", "zero_position"]
                    n145 = event-data() -> ()  [unwired: 1 in, 6 out]
                  }
                  event "home_x": Value Change {
                    w464 = T19[] [enum."home_x", enum."process_events"] items=["-------------------------", "about", "adjust_goto_buttons", "check_model", "close", "connect", "disable_all", "disable_step_n_loop", "enable_all", "enabled_state_change", "enable_step_n_loop", "exit", "get_device_id", "get_device_name", "get_digital_inputs", "get_digital_outputs", "get_firmware_ver", "get_high_speed", "get_high_speed_global", "get_low_speed", "get_low_speed_global", "get_non_volatile_var", "get_on_fly_speed_mode", "get_polarity", "get_product_id", "get_sspd_mode", "get_step_n_params", "get_volatile_var", "goto_x", "goto_y", "goto_z", "goto_u", "goto_interp", "home_x", "home_y", "home_z", "home_u", "init", "init_ui", "jog_x", "jog_y", "jog_z", "jog_u", "lock", "move_arc", "move_circular", "process_events", "run_standalone", "select_device", "stop_standalone", "set_device_name", "set_digital_outputs", "set_encoder_x", "set_encoder_y", "set_encoder_z", "set_encoder_u", "set_high_speed", "set_low_speed", "set_non_volatile_var", "set_on_fly_position", "set_on_fly_speed", "set_on_fly_speed_mode", "set_polarity", "set_pulse_x", "set_pulse_y", "set_pulse_z", "set_pulse_u", "set_step_n_params", "set_volatile_var", "stop_imm_x", "stop_imm_y", "stop_imm_z", "stop_imm_u", "stop_slow_x", "stop_slow_y", "stop_slow_z", "stop_slow_u", "store_perm", "unlock", "wait_til_idle", "zero_counter", "zero_position"]
                    n146 = event-data() -> ()  [unwired: 1 in, 6 out]
                  }
                  event "home_y": Value Change {
                    w466 = T19[] [enum."home_y", enum."process_events"] items=["-------------------------", "about", "adjust_goto_buttons", "check_model", "close", "connect", "disable_all", "disable_step_n_loop", "enable_all", "enabled_state_change", "enable_step_n_loop", "exit", "get_device_id", "get_device_name", "get_digital_inputs", "get_digital_outputs", "get_firmware_ver", "get_high_speed", "get_high_speed_global", "get_low_speed", "get_low_speed_global", "get_non_volatile_var", "get_on_fly_speed_mode", "get_polarity", "get_product_id", "get_sspd_mode", "get_step_n_params", "get_volatile_var", "goto_x", "goto_y", "goto_z", "goto_u", "goto_interp", "home_x", "home_y", "home_z", "home_u", "init", "init_ui", "jog_x", "jog_y", "jog_z", "jog_u", "lock", "move_arc", "move_circular", "process_events", "run_standalone", "select_device", "stop_standalone", "set_device_name", "set_digital_outputs", "set_encoder_x", "set_encoder_y", "set_encoder_z", "set_encoder_u", "set_high_speed", "set_low_speed", "set_non_volatile_var", "set_on_fly_position", "set_on_fly_speed", "set_on_fly_speed_mode", "set_polarity", "set_pulse_x", "set_pulse_y", "set_pulse_z", "set_pulse_u", "set_step_n_params", "set_volatile_var", "stop_imm_x", "stop_imm_y", "stop_imm_z", "stop_imm_u", "stop_slow_x", "stop_slow_y", "stop_slow_z", "stop_slow_u", "store_perm", "unlock", "wait_til_idle", "zero_counter", "zero_position"]
                    n147 = event-data() -> ()  [unwired: 1 in, 6 out]
                  }
                  event "home_z": Value Change {
                    w468 = T19[] [enum."home_z", enum."process_events"] items=["-------------------------", "about", "adjust_goto_buttons", "check_model", "close", "connect", "disable_all", "disable_step_n_loop", "enable_all", "enabled_state_change", "enable_step_n_loop", "exit", "get_device_id", "get_device_name", "get_digital_inputs", "get_digital_outputs", "get_firmware_ver", "get_high_speed", "get_high_speed_global", "get_low_speed", "get_low_speed_global", "get_non_volatile_var", "get_on_fly_speed_mode", "get_polarity", "get_product_id", "get_sspd_mode", "get_step_n_params", "get_volatile_var", "goto_x", "goto_y", "goto_z", "goto_u", "goto_interp", "home_x", "home_y", "home_z", "home_u", "init", "init_ui", "jog_x", "jog_y", "jog_z", "jog_u", "lock", "move_arc", "move_circular", "process_events", "run_standalone", "select_device", "stop_standalone", "set_device_name", "set_digital_outputs", "set_encoder_x", "set_encoder_y", "set_encoder_z", "set_encoder_u", "set_high_speed", "set_low_speed", "set_non_volatile_var", "set_on_fly_position", "set_on_fly_speed", "set_on_fly_speed_mode", "set_polarity", "set_pulse_x", "set_pulse_y", "set_pulse_z", "set_pulse_u", "set_step_n_params", "set_volatile_var", "stop_imm_x", "stop_imm_y", "stop_imm_z", "stop_imm_u", "stop_slow_x", "stop_slow_y", "stop_slow_z", "stop_slow_u", "store_perm", "unlock", "wait_til_idle", "zero_counter", "zero_position"]
                    n148 = event-data() -> ()  [unwired: 1 in, 6 out]
                  }
                  event "home_u": Value Change {
                    w470 = T19[] [enum."home_u", enum."process_events"] items=["-------------------------", "about", "adjust_goto_buttons", "check_model", "close", "connect", "disable_all", "disable_step_n_loop", "enable_all", "enabled_state_change", "enable_step_n_loop", "exit", "get_device_id", "get_device_name", "get_digital_inputs", "get_digital_outputs", "get_firmware_ver", "get_high_speed", "get_high_speed_global", "get_low_speed", "get_low_speed_global", "get_non_volatile_var", "get_on_fly_speed_mode", "get_polarity", "get_product_id", "get_sspd_mode", "get_step_n_params", "get_volatile_var", "goto_x", "goto_y", "goto_z", "goto_u", "goto_interp", "home_x", "home_y", "home_z", "home_u", "init", "init_ui", "jog_x", "jog_y", "jog_z", "jog_u", "lock", "move_arc", "move_circular", "process_events", "run_standalone", "select_device", "stop_standalone", "set_device_name", "set_digital_outputs", "set_encoder_x", "set_encoder_y", "set_encoder_z", "set_encoder_u", "set_high_speed", "set_low_speed", "set_non_volatile_var", "set_on_fly_position", "set_on_fly_speed", "set_on_fly_speed_mode", "set_polarity", "set_pulse_x", "set_pulse_y", "set_pulse_z", "set_pulse_u", "set_step_n_params", "set_volatile_var", "stop_imm_x", "stop_imm_y", "stop_imm_z", "stop_imm_u", "stop_slow_x", "stop_slow_y", "stop_slow_z", "stop_slow_u", "store_perm", "unlock", "wait_til_idle", "zero_counter", "zero_position"]
                    n149 = event-data() -> ()  [unwired: 1 in, 6 out]
                  }
                  event "stop_imm_x", "stop_arc_imm", "stop_circ_imm": Value Change {
                    w472 = T19[] [enum."stop_imm_x", enum."process_events"] items=["-------------------------", "about", "adjust_goto_buttons", "check_model", "close", "connect", "disable_all", "disable_step_n_loop", "enable_all", "enabled_state_change", "enable_step_n_loop", "exit", "get_device_id", "get_device_name", "get_digital_inputs", "get_digital_outputs", "get_firmware_ver", "get_high_speed", "get_high_speed_global", "get_low_speed", "get_low_speed_global", "get_non_volatile_var", "get_on_fly_speed_mode", "get_polarity", "get_product_id", "get_sspd_mode", "get_step_n_params", "get_volatile_var", "goto_x", "goto_y", "goto_z", "goto_u", "goto_interp", "home_x", "home_y", "home_z", "home_u", "init", "init_ui", "jog_x", "jog_y", "jog_z", "jog_u", "lock", "move_arc", "move_circular", "process_events", "run_standalone", "select_device", "stop_standalone", "set_device_name", "set_digital_outputs", "set_encoder_x", "set_encoder_y", "set_encoder_z", "set_encoder_u", "set_high_speed", "set_low_speed", "set_non_volatile_var", "set_on_fly_position", "set_on_fly_speed", "set_on_fly_speed_mode", "set_polarity", "set_pulse_x", "set_pulse_y", "set_pulse_z", "set_pulse_u", "set_step_n_params", "set_volatile_var", "stop_imm_x", "stop_imm_y", "stop_imm_z", "stop_imm_u", "stop_slow_x", "stop_slow_y", "stop_slow_z", "stop_slow_u", "store_perm", "unlock", "wait_til_idle", "zero_counter", "zero_position"]
                    n150 = event-data() -> ()  [unwired: 1 in, 6 out]
                  }
                  event "stop_imm_y": Value Change {
                    w474 = T19[] [enum."stop_imm_y", enum."process_events"] items=["-------------------------", "about", "adjust_goto_buttons", "check_model", "close", "connect", "disable_all", "disable_step_n_loop", "enable_all", "enabled_state_change", "enable_step_n_loop", "exit", "get_device_id", "get_device_name", "get_digital_inputs", "get_digital_outputs", "get_firmware_ver", "get_high_speed", "get_high_speed_global", "get_low_speed", "get_low_speed_global", "get_non_volatile_var", "get_on_fly_speed_mode", "get_polarity", "get_product_id", "get_sspd_mode", "get_step_n_params", "get_volatile_var", "goto_x", "goto_y", "goto_z", "goto_u", "goto_interp", "home_x", "home_y", "home_z", "home_u", "init", "init_ui", "jog_x", "jog_y", "jog_z", "jog_u", "lock", "move_arc", "move_circular", "process_events", "run_standalone", "select_device", "stop_standalone", "set_device_name", "set_digital_outputs", "set_encoder_x", "set_encoder_y", "set_encoder_z", "set_encoder_u", "set_high_speed", "set_low_speed", "set_non_volatile_var", "set_on_fly_position", "set_on_fly_speed", "set_on_fly_speed_mode", "set_polarity", "set_pulse_x", "set_pulse_y", "set_pulse_z", "set_pulse_u", "set_step_n_params", "set_volatile_var", "stop_imm_x", "stop_imm_y", "stop_imm_z", "stop_imm_u", "stop_slow_x", "stop_slow_y", "stop_slow_z", "stop_slow_u", "store_perm", "unlock", "wait_til_idle", "zero_counter", "zero_position"]
                    n151 = event-data() -> ()  [unwired: 1 in, 6 out]
                  }
                  event "stop_imm_z": Value Change {
                    w476 = T19[] [enum."stop_imm_z", enum."process_events"] items=["-------------------------", "about", "adjust_goto_buttons", "check_model", "close", "connect", "disable_all", "disable_step_n_loop", "enable_all", "enabled_state_change", "enable_step_n_loop", "exit", "get_device_id", "get_device_name", "get_digital_inputs", "get_digital_outputs", "get_firmware_ver", "get_high_speed", "get_high_speed_global", "get_low_speed", "get_low_speed_global", "get_non_volatile_var", "get_on_fly_speed_mode", "get_polarity", "get_product_id", "get_sspd_mode", "get_step_n_params", "get_volatile_var", "goto_x", "goto_y", "goto_z", "goto_u", "goto_interp", "home_x", "home_y", "home_z", "home_u", "init", "init_ui", "jog_x", "jog_y", "jog_z", "jog_u", "lock", "move_arc", "move_circular", "process_events", "run_standalone", "select_device", "stop_standalone", "set_device_name", "set_digital_outputs", "set_encoder_x", "set_encoder_y", "set_encoder_z", "set_encoder_u", "set_high_speed", "set_low_speed", "set_non_volatile_var", "set_on_fly_position", "set_on_fly_speed", "set_on_fly_speed_mode", "set_polarity", "set_pulse_x", "set_pulse_y", "set_pulse_z", "set_pulse_u", "set_step_n_params", "set_volatile_var", "stop_imm_x", "stop_imm_y", "stop_imm_z", "stop_imm_u", "stop_slow_x", "stop_slow_y", "stop_slow_z", "stop_slow_u", "store_perm", "unlock", "wait_til_idle", "zero_counter", "zero_position"]
                    n152 = event-data() -> ()  [unwired: 1 in, 6 out]
                  }
                  event "stop_imm_u": Value Change {
                    w478 = T19[] [enum."stop_imm_u", enum."process_events"] items=["-------------------------", "about", "adjust_goto_buttons", "check_model", "close", "connect", "disable_all", "disable_step_n_loop", "enable_all", "enabled_state_change", "enable_step_n_loop", "exit", "get_device_id", "get_device_name", "get_digital_inputs", "get_digital_outputs", "get_firmware_ver", "get_high_speed", "get_high_speed_global", "get_low_speed", "get_low_speed_global", "get_non_volatile_var", "get_on_fly_speed_mode", "get_polarity", "get_product_id", "get_sspd_mode", "get_step_n_params", "get_volatile_var", "goto_x", "goto_y", "goto_z", "goto_u", "goto_interp", "home_x", "home_y", "home_z", "home_u", "init", "init_ui", "jog_x", "jog_y", "jog_z", "jog_u", "lock", "move_arc", "move_circular", "process_events", "run_standalone", "select_device", "stop_standalone", "set_device_name", "set_digital_outputs", "set_encoder_x", "set_encoder_y", "set_encoder_z", "set_encoder_u", "set_high_speed", "set_low_speed", "set_non_volatile_var", "set_on_fly_position", "set_on_fly_speed", "set_on_fly_speed_mode", "set_polarity", "set_pulse_x", "set_pulse_y", "set_pulse_z", "set_pulse_u", "set_step_n_params", "set_volatile_var", "stop_imm_x", "stop_imm_y", "stop_imm_z", "stop_imm_u", "stop_slow_x", "stop_slow_y", "stop_slow_z", "stop_slow_u", "store_perm", "unlock", "wait_til_idle", "zero_counter", "zero_position"]
                    n153 = event-data() -> ()  [unwired: 1 in, 6 out]
                  }
                  event "stop_slow_x", "stop_arc_slow", "stop_circ_slow": Value Change {
                    w480 = T19[] [enum."stop_slow_x", enum."process_events"] items=["-------------------------", "about", "adjust_goto_buttons", "check_model", "close", "connect", "disable_all", "disable_step_n_loop", "enable_all", "enabled_state_change", "enable_step_n_loop", "exit", "get_device_id", "get_device_name", "get_digital_inputs", "get_digital_outputs", "get_firmware_ver", "get_high_speed", "get_high_speed_global", "get_low_speed", "get_low_speed_global", "get_non_volatile_var", "get_on_fly_speed_mode", "get_polarity", "get_product_id", "get_sspd_mode", "get_step_n_params", "get_volatile_var", "goto_x", "goto_y", "goto_z", "goto_u", "goto_interp", "home_x", "home_y", "home_z", "home_u", "init", "init_ui", "jog_x", "jog_y", "jog_z", "jog_u", "lock", "move_arc", "move_circular", "process_events", "run_standalone", "select_device", "stop_standalone", "set_device_name", "set_digital_outputs", "set_encoder_x", "set_encoder_y", "set_encoder_z", "set_encoder_u", "set_high_speed", "set_low_speed", "set_non_volatile_var", "set_on_fly_position", "set_on_fly_speed", "set_on_fly_speed_mode", "set_polarity", "set_pulse_x", "set_pulse_y", "set_pulse_z", "set_pulse_u", "set_step_n_params", "set_volatile_var", "stop_imm_x", "stop_imm_y", "stop_imm_z", "stop_imm_u", "stop_slow_x", "stop_slow_y", "stop_slow_z", "stop_slow_u", "store_perm", "unlock", "wait_til_idle", "zero_counter", "zero_position"]
                    n154 = event-data() -> ()  [unwired: 1 in, 6 out]
                  }
                  event "stop_slow_y": Value Change {
                    w482 = T19[] [enum."stop_slow_y", enum."process_events"] items=["-------------------------", "about", "adjust_goto_buttons", "check_model", "close", "connect", "disable_all", "disable_step_n_loop", "enable_all", "enabled_state_change", "enable_step_n_loop", "exit", "get_device_id", "get_device_name", "get_digital_inputs", "get_digital_outputs", "get_firmware_ver", "get_high_speed", "get_high_speed_global", "get_low_speed", "get_low_speed_global", "get_non_volatile_var", "get_on_fly_speed_mode", "get_polarity", "get_product_id", "get_sspd_mode", "get_step_n_params", "get_volatile_var", "goto_x", "goto_y", "goto_z", "goto_u", "goto_interp", "home_x", "home_y", "home_z", "home_u", "init", "init_ui", "jog_x", "jog_y", "jog_z", "jog_u", "lock", "move_arc", "move_circular", "process_events", "run_standalone", "select_device", "stop_standalone", "set_device_name", "set_digital_outputs", "set_encoder_x", "set_encoder_y", "set_encoder_z", "set_encoder_u", "set_high_speed", "set_low_speed", "set_non_volatile_var", "set_on_fly_position", "set_on_fly_speed", "set_on_fly_speed_mode", "set_polarity", "set_pulse_x", "set_pulse_y", "set_pulse_z", "set_pulse_u", "set_step_n_params", "set_volatile_var", "stop_imm_x", "stop_imm_y", "stop_imm_z", "stop_imm_u", "stop_slow_x", "stop_slow_y", "stop_slow_z", "stop_slow_u", "store_perm", "unlock", "wait_til_idle", "zero_counter", "zero_position"]
                    n155 = event-data() -> ()  [unwired: 1 in, 6 out]
                  }
                  event "stop_slow_z": Value Change {
                    w484 = T19[] [enum."stop_slow_z", enum."process_events"] items=["-------------------------", "about", "adjust_goto_buttons", "check_model", "close", "connect", "disable_all", "disable_step_n_loop", "enable_all", "enabled_state_change", "enable_step_n_loop", "exit", "get_device_id", "get_device_name", "get_digital_inputs", "get_digital_outputs", "get_firmware_ver", "get_high_speed", "get_high_speed_global", "get_low_speed", "get_low_speed_global", "get_non_volatile_var", "get_on_fly_speed_mode", "get_polarity", "get_product_id", "get_sspd_mode", "get_step_n_params", "get_volatile_var", "goto_x", "goto_y", "goto_z", "goto_u", "goto_interp", "home_x", "home_y", "home_z", "home_u", "init", "init_ui", "jog_x", "jog_y", "jog_z", "jog_u", "lock", "move_arc", "move_circular", "process_events", "run_standalone", "select_device", "stop_standalone", "set_device_name", "set_digital_outputs", "set_encoder_x", "set_encoder_y", "set_encoder_z", "set_encoder_u", "set_high_speed", "set_low_speed", "set_non_volatile_var", "set_on_fly_position", "set_on_fly_speed", "set_on_fly_speed_mode", "set_polarity", "set_pulse_x", "set_pulse_y", "set_pulse_z", "set_pulse_u", "set_step_n_params", "set_volatile_var", "stop_imm_x", "stop_imm_y", "stop_imm_z", "stop_imm_u", "stop_slow_x", "stop_slow_y", "stop_slow_z", "stop_slow_u", "store_perm", "unlock", "wait_til_idle", "zero_counter", "zero_position"]
                    n156 = event-data() -> ()  [unwired: 1 in, 6 out]
                  }
                  event "stop_slow_u": Value Change {
                    w486 = T19[] [enum."stop_slow_u", enum."process_events"] items=["-------------------------", "about", "adjust_goto_buttons", "check_model", "close", "connect", "disable_all", "disable_step_n_loop", "enable_all", "enabled_state_change", "enable_step_n_loop", "exit", "get_device_id", "get_device_name", "get_digital_inputs", "get_digital_outputs", "get_firmware_ver", "get_high_speed", "get_high_speed_global", "get_low_speed", "get_low_speed_global", "get_non_volatile_var", "get_on_fly_speed_mode", "get_polarity", "get_product_id", "get_sspd_mode", "get_step_n_params", "get_volatile_var", "goto_x", "goto_y", "goto_z", "goto_u", "goto_interp", "home_x", "home_y", "home_z", "home_u", "init", "init_ui", "jog_x", "jog_y", "jog_z", "jog_u", "lock", "move_arc", "move_circular", "process_events", "run_standalone", "select_device", "stop_standalone", "set_device_name", "set_digital_outputs", "set_encoder_x", "set_encoder_y", "set_encoder_z", "set_encoder_u", "set_high_speed", "set_low_speed", "set_non_volatile_var", "set_on_fly_position", "set_on_fly_speed", "set_on_fly_speed_mode", "set_polarity", "set_pulse_x", "set_pulse_y", "set_pulse_z", "set_pulse_u", "set_step_n_params", "set_volatile_var", "stop_imm_x", "stop_imm_y", "stop_imm_z", "stop_imm_u", "stop_slow_x", "stop_slow_y", "stop_slow_z", "stop_slow_u", "store_perm", "unlock", "wait_til_idle", "zero_counter", "zero_position"]
                    n157 = event-data() -> ()  [unwired: 1 in, 6 out]
                  }
                  event "pulse_set_x": Value Change {
                    w488 = T19[] [enum."set_pulse_x", enum."process_events"] items=["-------------------------", "about", "adjust_goto_buttons", "check_model", "close", "connect", "disable_all", "disable_step_n_loop", "enable_all", "enabled_state_change", "enable_step_n_loop", "exit", "get_device_id", "get_device_name", "get_digital_inputs", "get_digital_outputs", "get_firmware_ver", "get_high_speed", "get_high_speed_global", "get_low_speed", "get_low_speed_global", "get_non_volatile_var", "get_on_fly_speed_mode", "get_polarity", "get_product_id", "get_sspd_mode", "get_step_n_params", "get_volatile_var", "goto_x", "goto_y", "goto_z", "goto_u", "goto_interp", "home_x", "home_y", "home_z", "home_u", "init", "init_ui", "jog_x", "jog_y", "jog_z", "jog_u", "lock", "move_arc", "move_circular", "process_events", "run_standalone", "select_device", "stop_standalone", "set_device_name", "set_digital_outputs", "set_encoder_x", "set_encoder_y", "set_encoder_z", "set_encoder_u", "set_high_speed", "set_low_speed", "set_non_volatile_var", "set_on_fly_position", "set_on_fly_speed", "set_on_fly_speed_mode", "set_polarity", "set_pulse_x", "set_pulse_y", "set_pulse_z", "set_pulse_u", "set_step_n_params", "set_volatile_var", "stop_imm_x", "stop_imm_y", "stop_imm_z", "stop_imm_u", "stop_slow_x", "stop_slow_y", "stop_slow_z", "stop_slow_u", "store_perm", "unlock", "wait_til_idle", "zero_counter", "zero_position"]
                    n158 = event-data() -> ()  [unwired: 1 in, 6 out]
                  }
                  event "pulse_set_y": Value Change {
                    w490 = T19[] [enum."set_pulse_y", enum."process_events"] items=["-------------------------", "about", "adjust_goto_buttons", "check_model", "close", "connect", "disable_all", "disable_step_n_loop", "enable_all", "enabled_state_change", "enable_step_n_loop", "exit", "get_device_id", "get_device_name", "get_digital_inputs", "get_digital_outputs", "get_firmware_ver", "get_high_speed", "get_high_speed_global", "get_low_speed", "get_low_speed_global", "get_non_volatile_var", "get_on_fly_speed_mode", "get_polarity", "get_product_id", "get_sspd_mode", "get_step_n_params", "get_volatile_var", "goto_x", "goto_y", "goto_z", "goto_u", "goto_interp", "home_x", "home_y", "home_z", "home_u", "init", "init_ui", "jog_x", "jog_y", "jog_z", "jog_u", "lock", "move_arc", "move_circular", "process_events", "run_standalone", "select_device", "stop_standalone", "set_device_name", "set_digital_outputs", "set_encoder_x", "set_encoder_y", "set_encoder_z", "set_encoder_u", "set_high_speed", "set_low_speed", "set_non_volatile_var", "set_on_fly_position", "set_on_fly_speed", "set_on_fly_speed_mode", "set_polarity", "set_pulse_x", "set_pulse_y", "set_pulse_z", "set_pulse_u", "set_step_n_params", "set_volatile_var", "stop_imm_x", "stop_imm_y", "stop_imm_z", "stop_imm_u", "stop_slow_x", "stop_slow_y", "stop_slow_z", "stop_slow_u", "store_perm", "unlock", "wait_til_idle", "zero_counter", "zero_position"]
                    n159 = event-data() -> ()  [unwired: 1 in, 6 out]
                  }
                  event "pulse_set_z": Value Change {
                    w492 = T19[] [enum."set_pulse_z", enum."process_events"] items=["-------------------------", "about", "adjust_goto_buttons", "check_model", "close", "connect", "disable_all", "disable_step_n_loop", "enable_all", "enabled_state_change", "enable_step_n_loop", "exit", "get_device_id", "get_device_name", "get_digital_inputs", "get_digital_outputs", "get_firmware_ver", "get_high_speed", "get_high_speed_global", "get_low_speed", "get_low_speed_global", "get_non_volatile_var", "get_on_fly_speed_mode", "get_polarity", "get_product_id", "get_sspd_mode", "get_step_n_params", "get_volatile_var", "goto_x", "goto_y", "goto_z", "goto_u", "goto_interp", "home_x", "home_y", "home_z", "home_u", "init", "init_ui", "jog_x", "jog_y", "jog_z", "jog_u", "lock", "move_arc", "move_circular", "process_events", "run_standalone", "select_device", "stop_standalone", "set_device_name", "set_digital_outputs", "set_encoder_x", "set_encoder_y", "set_encoder_z", "set_encoder_u", "set_high_speed", "set_low_speed", "set_non_volatile_var", "set_on_fly_position", "set_on_fly_speed", "set_on_fly_speed_mode", "set_polarity", "set_pulse_x", "set_pulse_y", "set_pulse_z", "set_pulse_u", "set_step_n_params", "set_volatile_var", "stop_imm_x", "stop_imm_y", "stop_imm_z", "stop_imm_u", "stop_slow_x", "stop_slow_y", "stop_slow_z", "stop_slow_u", "store_perm", "unlock", "wait_til_idle", "zero_counter", "zero_position"]
                    n160 = event-data() -> ()  [unwired: 1 in, 6 out]
                  }
                  event "pulse_set_u": Value Change {
                    w494 = T19[] [enum."set_pulse_u", enum."process_events"] items=["-------------------------", "about", "adjust_goto_buttons", "check_model", "close", "connect", "disable_all", "disable_step_n_loop", "enable_all", "enabled_state_change", "enable_step_n_loop", "exit", "get_device_id", "get_device_name", "get_digital_inputs", "get_digital_outputs", "get_firmware_ver", "get_high_speed", "get_high_speed_global", "get_low_speed", "get_low_speed_global", "get_non_volatile_var", "get_on_fly_speed_mode", "get_polarity", "get_product_id", "get_sspd_mode", "get_step_n_params", "get_volatile_var", "goto_x", "goto_y", "goto_z", "goto_u", "goto_interp", "home_x", "home_y", "home_z", "home_u", "init", "init_ui", "jog_x", "jog_y", "jog_z", "jog_u", "lock", "move_arc", "move_circular", "process_events", "run_standalone", "select_device", "stop_standalone", "set_device_name", "set_digital_outputs", "set_encoder_x", "set_encoder_y", "set_encoder_z", "set_encoder_u", "set_high_speed", "set_low_speed", "set_non_volatile_var", "set_on_fly_position", "set_on_fly_speed", "set_on_fly_speed_mode", "set_polarity", "set_pulse_x", "set_pulse_y", "set_pulse_z", "set_pulse_u", "set_step_n_params", "set_volatile_var", "stop_imm_x", "stop_imm_y", "stop_imm_z", "stop_imm_u", "stop_slow_x", "stop_slow_y", "stop_slow_z", "stop_slow_u", "store_perm", "unlock", "wait_til_idle", "zero_counter", "zero_position"]
                    n161 = event-data() -> ()  [unwired: 1 in, 6 out]
                  }
                  event "encoder_set_x": Value Change {
                    w496 = T19[] [enum."set_encoder_x", enum."process_events"] items=["-------------------------", "about", "adjust_goto_buttons", "check_model", "close", "connect", "disable_all", "disable_step_n_loop", "enable_all", "enabled_state_change", "enable_step_n_loop", "exit", "get_device_id", "get_device_name", "get_digital_inputs", "get_digital_outputs", "get_firmware_ver", "get_high_speed", "get_high_speed_global", "get_low_speed", "get_low_speed_global", "get_non_volatile_var", "get_on_fly_speed_mode", "get_polarity", "get_product_id", "get_sspd_mode", "get_step_n_params", "get_volatile_var", "goto_x", "goto_y", "goto_z", "goto_u", "goto_interp", "home_x", "home_y", "home_z", "home_u", "init", "init_ui", "jog_x", "jog_y", "jog_z", "jog_u", "lock", "move_arc", "move_circular", "process_events", "run_standalone", "select_device", "stop_standalone", "set_device_name", "set_digital_outputs", "set_encoder_x", "set_encoder_y", "set_encoder_z", "set_encoder_u", "set_high_speed", "set_low_speed", "set_non_volatile_var", "set_on_fly_position", "set_on_fly_speed", "set_on_fly_speed_mode", "set_polarity", "set_pulse_x", "set_pulse_y", "set_pulse_z", "set_pulse_u", "set_step_n_params", "set_volatile_var", "stop_imm_x", "stop_imm_y", "stop_imm_z", "stop_imm_u", "stop_slow_x", "stop_slow_y", "stop_slow_z", "stop_slow_u", "store_perm", "unlock", "wait_til_idle", "zero_counter", "zero_position"]
                    n162 = event-data() -> ()  [unwired: 1 in, 6 out]
                  }
                  event "encoder_set_y": Value Change {
                    w498 = T19[] [enum."set_encoder_y", enum."process_events"] items=["-------------------------", "about", "adjust_goto_buttons", "check_model", "close", "connect", "disable_all", "disable_step_n_loop", "enable_all", "enabled_state_change", "enable_step_n_loop", "exit", "get_device_id", "get_device_name", "get_digital_inputs", "get_digital_outputs", "get_firmware_ver", "get_high_speed", "get_high_speed_global", "get_low_speed", "get_low_speed_global", "get_non_volatile_var", "get_on_fly_speed_mode", "get_polarity", "get_product_id", "get_sspd_mode", "get_step_n_params", "get_volatile_var", "goto_x", "goto_y", "goto_z", "goto_u", "goto_interp", "home_x", "home_y", "home_z", "home_u", "init", "init_ui", "jog_x", "jog_y", "jog_z", "jog_u", "lock", "move_arc", "move_circular", "process_events", "run_standalone", "select_device", "stop_standalone", "set_device_name", "set_digital_outputs", "set_encoder_x", "set_encoder_y", "set_encoder_z", "set_encoder_u", "set_high_speed", "set_low_speed", "set_non_volatile_var", "set_on_fly_position", "set_on_fly_speed", "set_on_fly_speed_mode", "set_polarity", "set_pulse_x", "set_pulse_y", "set_pulse_z", "set_pulse_u", "set_step_n_params", "set_volatile_var", "stop_imm_x", "stop_imm_y", "stop_imm_z", "stop_imm_u", "stop_slow_x", "stop_slow_y", "stop_slow_z", "stop_slow_u", "store_perm", "unlock", "wait_til_idle", "zero_counter", "zero_position"]
                    n163 = event-data() -> ()  [unwired: 1 in, 6 out]
                  }
                  event "encoder_set_z": Value Change {
                    w500 = T19[] [enum."set_encoder_z", enum."process_events"] items=["-------------------------", "about", "adjust_goto_buttons", "check_model", "close", "connect", "disable_all", "disable_step_n_loop", "enable_all", "enabled_state_change", "enable_step_n_loop", "exit", "get_device_id", "get_device_name", "get_digital_inputs", "get_digital_outputs", "get_firmware_ver", "get_high_speed", "get_high_speed_global", "get_low_speed", "get_low_speed_global", "get_non_volatile_var", "get_on_fly_speed_mode", "get_polarity", "get_product_id", "get_sspd_mode", "get_step_n_params", "get_volatile_var", "goto_x", "goto_y", "goto_z", "goto_u", "goto_interp", "home_x", "home_y", "home_z", "home_u", "init", "init_ui", "jog_x", "jog_y", "jog_z", "jog_u", "lock", "move_arc", "move_circular", "process_events", "run_standalone", "select_device", "stop_standalone", "set_device_name", "set_digital_outputs", "set_encoder_x", "set_encoder_y", "set_encoder_z", "set_encoder_u", "set_high_speed", "set_low_speed", "set_non_volatile_var", "set_on_fly_position", "set_on_fly_speed", "set_on_fly_speed_mode", "set_polarity", "set_pulse_x", "set_pulse_y", "set_pulse_z", "set_pulse_u", "set_step_n_params", "set_volatile_var", "stop_imm_x", "stop_imm_y", "stop_imm_z", "stop_imm_u", "stop_slow_x", "stop_slow_y", "stop_slow_z", "stop_slow_u", "store_perm", "unlock", "wait_til_idle", "zero_counter", "zero_position"]
                    n164 = event-data() -> ()  [unwired: 1 in, 6 out]
                  }
                  event "encoder_set_u": Value Change {
                    w502 = T19[] [enum."set_encoder_u", enum."process_events"] items=["-------------------------", "about", "adjust_goto_buttons", "check_model", "close", "connect", "disable_all", "disable_step_n_loop", "enable_all", "enabled_state_change", "enable_step_n_loop", "exit", "get_device_id", "get_device_name", "get_digital_inputs", "get_digital_outputs", "get_firmware_ver", "get_high_speed", "get_high_speed_global", "get_low_speed", "get_low_speed_global", "get_non_volatile_var", "get_on_fly_speed_mode", "get_polarity", "get_product_id", "get_sspd_mode", "get_step_n_params", "get_volatile_var", "goto_x", "goto_y", "goto_z", "goto_u", "goto_interp", "home_x", "home_y", "home_z", "home_u", "init", "init_ui", "jog_x", "jog_y", "jog_z", "jog_u", "lock", "move_arc", "move_circular", "process_events", "run_standalone", "select_device", "stop_standalone", "set_device_name", "set_digital_outputs", "set_encoder_x", "set_encoder_y", "set_encoder_z", "set_encoder_u", "set_high_speed", "set_low_speed", "set_non_volatile_var", "set_on_fly_position", "set_on_fly_speed", "set_on_fly_speed_mode", "set_polarity", "set_pulse_x", "set_pulse_y", "set_pulse_z", "set_pulse_u", "set_step_n_params", "set_volatile_var", "stop_imm_x", "stop_imm_y", "stop_imm_z", "stop_imm_u", "stop_slow_x", "stop_slow_y", "stop_slow_z", "stop_slow_u", "store_perm", "unlock", "wait_til_idle", "zero_counter", "zero_position"]
                    n165 = event-data() -> ()  [unwired: 1 in, 6 out]
                  }
                  event "set_device_name": Value Change {
                    w504 = T19[] [enum."set_device_name", enum."store_perm", enum."get_device_name", enum."process_events"] items=["-------------------------", "about", "adjust_goto_buttons", "check_model", "close", "connect", "disable_all", "disable_step_n_loop", "enable_all", "enabled_state_change", "enable_step_n_loop", "exit", "get_device_id", "get_device_name", "get_digital_inputs", "get_digital_outputs", "get_firmware_ver", "get_high_speed", "get_high_speed_global", "get_low_speed", "get_low_speed_global", "get_non_volatile_var", "get_on_fly_speed_mode", "get_polarity", "get_product_id", "get_sspd_mode", "get_step_n_params", "get_volatile_var", "goto_x", "goto_y", "goto_z", "goto_u", "goto_interp", "home_x", "home_y", "home_z", "home_u", "init", "init_ui", "jog_x", "jog_y", "jog_z", "jog_u", "lock", "move_arc", "move_circular", "process_events", "run_standalone", "select_device", "stop_standalone", "set_device_name", "set_digital_outputs", "set_encoder_x", "set_encoder_y", "set_encoder_z", "set_encoder_u", "set_high_speed", "set_low_speed", "set_non_volatile_var", "set_on_fly_position", "set_on_fly_speed", "set_on_fly_speed_mode", "set_polarity", "set_pulse_x", "set_pulse_y", "set_pulse_z", "set_pulse_u", "set_step_n_params", "set_volatile_var", "stop_imm_x", "stop_imm_y", "stop_imm_z", "stop_imm_u", "stop_slow_x", "stop_slow_y", "stop_slow_z", "stop_slow_u", "store_perm", "unlock", "wait_til_idle", "zero_counter", "zero_position"]
                    n166 = event-data() -> ()  [unwired: 1 in, 6 out]
                  }
                  event "set_pol_val": Value Change {
                    w506 = T19[] [enum."set_polarity", enum."store_perm", enum."get_polarity", enum."process_events"] items=["-------------------------", "about", "adjust_goto_buttons", "check_model", "close", "connect", "disable_all", "disable_step_n_loop", "enable_all", "enabled_state_change", "enable_step_n_loop", "exit", "get_device_id", "get_device_name", "get_digital_inputs", "get_digital_outputs", "get_firmware_ver", "get_high_speed", "get_high_speed_global", "get_low_speed", "get_low_speed_global", "get_non_volatile_var", "get_on_fly_speed_mode", "get_polarity", "get_product_id", "get_sspd_mode", "get_step_n_params", "get_volatile_var", "goto_x", "goto_y", "goto_z", "goto_u", "goto_interp", "home_x", "home_y", "home_z", "home_u", "init", "init_ui", "jog_x", "jog_y", "jog_z", "jog_u", "lock", "move_arc", "move_circular", "process_events", "run_standalone", "select_device", "stop_standalone", "set_device_name", "set_digital_outputs", "set_encoder_x", "set_encoder_y", "set_encoder_z", "set_encoder_u", "set_high_speed", "set_low_speed", "set_non_volatile_var", "set_on_fly_position", "set_on_fly_speed", "set_on_fly_speed_mode", "set_polarity", "set_pulse_x", "set_pulse_y", "set_pulse_z", "set_pulse_u", "set_step_n_params", "set_volatile_var", "stop_imm_x", "stop_imm_y", "stop_imm_z", "stop_imm_u", "stop_slow_x", "stop_slow_y", "stop_slow_z", "stop_slow_u", "store_perm", "unlock", "wait_til_idle", "zero_counter", "zero_position"]
                    n167 = event-data() -> ()  [unwired: 1 in, 6 out]
                  }
                  event Value Change {
                    w508 = T19[] [enum."get_polarity", enum."process_events"] items=["-------------------------", "about", "adjust_goto_buttons", "check_model", "close", "connect", "disable_all", "disable_step_n_loop", "enable_all", "enabled_state_change", "enable_step_n_loop", "exit", "get_device_id", "get_device_name", "get_digital_inputs", "get_digital_outputs", "get_firmware_ver", "get_high_speed", "get_high_speed_global", "get_low_speed", "get_low_speed_global", "get_non_volatile_var", "get_on_fly_speed_mode", "get_polarity", "get_product_id", "get_sspd_mode", "get_step_n_params", "get_volatile_var", "goto_x", "goto_y", "goto_z", "goto_u", "goto_interp", "home_x", "home_y", "home_z", "home_u", "init", "init_ui", "jog_x", "jog_y", "jog_z", "jog_u", "lock", "move_arc", "move_circular", "process_events", "run_standalone", "select_device", "stop_standalone", "set_device_name", "set_digital_outputs", "set_encoder_x", "set_encoder_y", "set_encoder_z", "set_encoder_u", "set_high_speed", "set_low_speed", "set_non_volatile_var", "set_on_fly_position", "set_on_fly_speed", "set_on_fly_speed_mode", "set_polarity", "set_pulse_x", "set_pulse_y", "set_pulse_z", "set_pulse_u", "set_step_n_params", "set_volatile_var", "stop_imm_x", "stop_imm_y", "stop_imm_z", "stop_imm_u", "stop_slow_x", "stop_slow_y", "stop_slow_z", "stop_slow_u", "store_perm", "unlock", "wait_til_idle", "zero_counter", "zero_position"]
                    n168 = event-data() -> ()  [unwired: 1 in, 6 out]
                  }
                  event "move_arc": Value Change {
                    w510 = T19[] [enum."move_arc", enum."process_events"] items=["-------------------------", "about", "adjust_goto_buttons", "check_model", "close", "connect", "disable_all", "disable_step_n_loop", "enable_all", "enabled_state_change", "enable_step_n_loop", "exit", "get_device_id", "get_device_name", "get_digital_inputs", "get_digital_outputs", "get_firmware_ver", "get_high_speed", "get_high_speed_global", "get_low_speed", "get_low_speed_global", "get_non_volatile_var", "get_on_fly_speed_mode", "get_polarity", "get_product_id", "get_sspd_mode", "get_step_n_params", "get_volatile_var", "goto_x", "goto_y", "goto_z", "goto_u", "goto_interp", "home_x", "home_y", "home_z", "home_u", "init", "init_ui", "jog_x", "jog_y", "jog_z", "jog_u", "lock", "move_arc", "move_circular", "process_events", "run_standalone", "select_device", "stop_standalone", "set_device_name", "set_digital_outputs", "set_encoder_x", "set_encoder_y", "set_encoder_z", "set_encoder_u", "set_high_speed", "set_low_speed", "set_non_volatile_var", "set_on_fly_position", "set_on_fly_speed", "set_on_fly_speed_mode", "set_polarity", "set_pulse_x", "set_pulse_y", "set_pulse_z", "set_pulse_u", "set_step_n_params", "set_volatile_var", "stop_imm_x", "stop_imm_y", "stop_imm_z", "stop_imm_u", "stop_slow_x", "stop_slow_y", "stop_slow_z", "stop_slow_u", "store_perm", "unlock", "wait_til_idle", "zero_counter", "zero_position"]
                    n169 = event-data() -> ()  [unwired: 1 in, 6 out]
                  }
                  event "move_circle": Value Change {
                    w512 = T19[] [enum."move_circular", enum."process_events"] items=["-------------------------", "about", "adjust_goto_buttons", "check_model", "close", "connect", "disable_all", "disable_step_n_loop", "enable_all", "enabled_state_change", "enable_step_n_loop", "exit", "get_device_id", "get_device_name", "get_digital_inputs", "get_digital_outputs", "get_firmware_ver", "get_high_speed", "get_high_speed_global", "get_low_speed", "get_low_speed_global", "get_non_volatile_var", "get_on_fly_speed_mode", "get_polarity", "get_product_id", "get_sspd_mode", "get_step_n_params", "get_volatile_var", "goto_x", "goto_y", "goto_z", "goto_u", "goto_interp", "home_x", "home_y", "home_z", "home_u", "init", "init_ui", "jog_x", "jog_y", "jog_z", "jog_u", "lock", "move_arc", "move_circular", "process_events", "run_standalone", "select_device", "stop_standalone", "set_device_name", "set_digital_outputs", "set_encoder_x", "set_encoder_y", "set_encoder_z", "set_encoder_u", "set_high_speed", "set_low_speed", "set_non_volatile_var", "set_on_fly_position", "set_on_fly_speed", "set_on_fly_speed_mode", "set_polarity", "set_pulse_x", "set_pulse_y", "set_pulse_z", "set_pulse_u", "set_step_n_params", "set_volatile_var", "stop_imm_x", "stop_imm_y", "stop_imm_z", "stop_imm_u", "stop_slow_x", "stop_slow_y", "stop_slow_z", "stop_slow_u", "store_perm", "unlock", "wait_til_idle", "zero_counter", "zero_position"]
                    n170 = event-data() -> ()  [unwired: 1 in, 6 out]
                  }
                  event "enable_disable_step_n": Value Change {
                    n171 = event-data() -> ("NewVal"=w513:bool)  [unwired: 1 in, 5 out]
                    n172 = case shown="False" w513 {
                      tunnel: [w516 w517] -> w515
                      frame False {
                        w516 = T19[] [enum."disable_step_n_loop", enum."store_perm", enum."process_events"] items=["-------------------------", "about", "adjust_goto_buttons", "check_model", "close", "connect", "disable_all", "disable_step_n_loop", "enable_all", "enabled_state_change", "enable_step_n_loop", "exit", "get_device_id", "get_device_name", "get_digital_inputs", "get_digital_outputs", "get_firmware_ver", "get_high_speed", "get_high_speed_global", "get_low_speed", "get_low_speed_global", "get_non_volatile_var", "get_on_fly_speed_mode", "get_polarity", "get_product_id", "get_sspd_mode", "get_step_n_params", "get_volatile_var", "goto_x", "goto_y", "goto_z", "goto_u", "goto_interp", "home_x", "home_y", "home_z", "home_u", "init", "init_ui", "jog_x", "jog_y", "jog_z", "jog_u", "lock", "move_arc", "move_circular", "process_events", "run_standalone", "select_device", "stop_standalone", "set_device_name", "set_digital_outputs", "set_encoder_x", "set_encoder_y", "set_encoder_z", "set_encoder_u", "set_high_speed", "set_low_speed", "set_non_volatile_var", "set_on_fly_position", "set_on_fly_speed", "set_on_fly_speed_mode", "set_polarity", "set_pulse_x", "set_pulse_y", "set_pulse_z", "set_pulse_u", "set_step_n_params", "set_volatile_var", "stop_imm_x", "stop_imm_y", "stop_imm_z", "stop_imm_u", "stop_slow_x", "stop_slow_y", "stop_slow_z", "stop_slow_u", "store_perm", "unlock", "wait_til_idle", "zero_counter", "zero_position"]
                      }
                      frame True {
                        w517 = T19[] [enum."enable_step_n_loop", enum."store_perm", enum."process_events"] items=["-------------------------", "about", "adjust_goto_buttons", "check_model", "close", "connect", "disable_all", "disable_step_n_loop", "enable_all", "enabled_state_change", "enable_step_n_loop", "exit", "get_device_id", "get_device_name", "get_digital_inputs", "get_digital_outputs", "get_firmware_ver", "get_high_speed", "get_high_speed_global", "get_low_speed", "get_low_speed_global", "get_non_volatile_var", "get_on_fly_speed_mode", "get_polarity", "get_product_id", "get_sspd_mode", "get_step_n_params", "get_volatile_var", "goto_x", "goto_y", "goto_z", "goto_u", "goto_interp", "home_x", "home_y", "home_z", "home_u", "init", "init_ui", "jog_x", "jog_y", "jog_z", "jog_u", "lock", "move_arc", "move_circular", "process_events", "run_standalone", "select_device", "stop_standalone", "set_device_name", "set_digital_outputs", "set_encoder_x", "set_encoder_y", "set_encoder_z", "set_encoder_u", "set_high_speed", "set_low_speed", "set_non_volatile_var", "set_on_fly_position", "set_on_fly_speed", "set_on_fly_speed_mode", "set_polarity", "set_pulse_x", "set_pulse_y", "set_pulse_z", "set_pulse_u", "set_step_n_params", "set_volatile_var", "stop_imm_x", "stop_imm_y", "stop_imm_z", "stop_imm_u", "stop_slow_x", "stop_slow_y", "stop_slow_z", "stop_slow_u", "store_perm", "unlock", "wait_til_idle", "zero_counter", "zero_position"]
                      }
                    }
                  }
                  event "Tab Control": Value Change {
                    n173 = event-data() -> ("NewVal"=w518:T3)  [unwired: 1 in, 5 out]
                    n174 = case shown="\"Digital I/O\"" w518 {
                      tunnel: [w521 w522 w523 w524 w525] -> w520
                      frame "Step N Loop" {
                        w521 = T19[] [enum."get_step_n_params", enum."process_events"] items=["-------------------------", "about", "adjust_goto_buttons", "check_model", "close", "connect", "disable_all", "disable_step_n_loop", "enable_all", "enabled_state_change", "enable_step_n_loop", "exit", "get_device_id", "get_device_name", "get_digital_inputs", "get_digital_outputs", "get_firmware_ver", "get_high_speed", "get_high_speed_global", "get_low_speed", "get_low_speed_global", "get_non_volatile_var", "get_on_fly_speed_mode", "get_polarity", "get_product_id", "get_sspd_mode", "get_step_n_params", "get_volatile_var", "goto_x", "goto_y", "goto_z", "goto_u", "goto_interp", "home_x", "home_y", "home_z", "home_u", "init", "init_ui", "jog_x", "jog_y", "jog_z", "jog_u", "lock", "move_arc", "move_circular", "process_events", "run_standalone", "select_device", "stop_standalone", "set_device_name", "set_digital_outputs", "set_encoder_x", "set_encoder_y", "set_encoder_z", "set_encoder_u", "set_high_speed", "set_low_speed", "set_non_volatile_var", "set_on_fly_position", "set_on_fly_speed", "set_on_fly_speed_mode", "set_polarity", "set_pulse_x", "set_pulse_y", "set_pulse_z", "set_pulse_u", "set_step_n_params", "set_volatile_var", "stop_imm_x", "stop_imm_y", "stop_imm_z", "stop_imm_u", "stop_slow_x", "stop_slow_y", "stop_slow_z", "stop_slow_u", "store_perm", "unlock", "wait_til_idle", "zero_counter", "zero_position"]
                      }
                      frame "Polarity" {
                        w522 = T19[] [enum."get_polarity", enum."process_events"] items=["-------------------------", "about", "adjust_goto_buttons", "check_model", "close", "connect", "disable_all", "disable_step_n_loop", "enable_all", "enabled_state_change", "enable_step_n_loop", "exit", "get_device_id", "get_device_name", "get_digital_inputs", "get_digital_outputs", "get_firmware_ver", "get_high_speed", "get_high_speed_global", "get_low_speed", "get_low_speed_global", "get_non_volatile_var", "get_on_fly_speed_mode", "get_polarity", "get_product_id", "get_sspd_mode", "get_step_n_params", "get_volatile_var", "goto_x", "goto_y", "goto_z", "goto_u", "goto_interp", "home_x", "home_y", "home_z", "home_u", "init", "init_ui", "jog_x", "jog_y", "jog_z", "jog_u", "lock", "move_arc", "move_circular", "process_events", "run_standalone", "select_device", "stop_standalone", "set_device_name", "set_digital_outputs", "set_encoder_x", "set_encoder_y", "set_encoder_z", "set_encoder_u", "set_high_speed", "set_low_speed", "set_non_volatile_var", "set_on_fly_position", "set_on_fly_speed", "set_on_fly_speed_mode", "set_polarity", "set_pulse_x", "set_pulse_y", "set_pulse_z", "set_pulse_u", "set_step_n_params", "set_volatile_var", "stop_imm_x", "stop_imm_y", "stop_imm_z", "stop_imm_u", "stop_slow_x", "stop_slow_y", "stop_slow_z", "stop_slow_u", "store_perm", "unlock", "wait_til_idle", "zero_counter", "zero_position"]
                      }
                      frame "Motion Control (Advanced)" {
                        w523 = T19[] [enum."get_on_fly_speed_mode", enum."process_events"] items=["-------------------------", "about", "adjust_goto_buttons", "check_model", "close", "connect", "disable_all", "disable_step_n_loop", "enable_all", "enabled_state_change", "enable_step_n_loop", "exit", "get_device_id", "get_device_name", "get_digital_inputs", "get_digital_outputs", "get_firmware_ver", "get_high_speed", "get_high_speed_global", "get_low_speed", "get_low_speed_global", "get_non_volatile_var", "get_on_fly_speed_mode", "get_polarity", "get_product_id", "get_sspd_mode", "get_step_n_params", "get_volatile_var", "goto_x", "goto_y", "goto_z", "goto_u", "goto_interp", "home_x", "home_y", "home_z", "home_u", "init", "init_ui", "jog_x", "jog_y", "jog_z", "jog_u", "lock", "move_arc", "move_circular", "process_events", "run_standalone", "select_device", "stop_standalone", "set_device_name", "set_digital_outputs", "set_encoder_x", "set_encoder_y", "set_encoder_z", "set_encoder_u", "set_high_speed", "set_low_speed", "set_non_volatile_var", "set_on_fly_position", "set_on_fly_speed", "set_on_fly_speed_mode", "set_polarity", "set_pulse_x", "set_pulse_y", "set_pulse_z", "set_pulse_u", "set_step_n_params", "set_volatile_var", "stop_imm_x", "stop_imm_y", "stop_imm_z", "stop_imm_u", "stop_slow_x", "stop_slow_y", "stop_slow_z", "stop_slow_u", "store_perm", "unlock", "wait_til_idle", "zero_counter", "zero_position"]
                      }
                      frame "Digital I/O" {
                        w524 = T19[] [enum."get_digital_outputs", enum."process_events"] items=["-------------------------", "about", "adjust_goto_buttons", "check_model", "close", "connect", "disable_all", "disable_step_n_loop", "enable_all", "enabled_state_change", "enable_step_n_loop", "exit", "get_device_id", "get_device_name", "get_digital_inputs", "get_digital_outputs", "get_firmware_ver", "get_high_speed", "get_high_speed_global", "get_low_speed", "get_low_speed_global", "get_non_volatile_var", "get_on_fly_speed_mode", "get_polarity", "get_product_id", "get_sspd_mode", "get_step_n_params", "get_volatile_var", "goto_x", "goto_y", "goto_z", "goto_u", "goto_interp", "home_x", "home_y", "home_z", "home_u", "init", "init_ui", "jog_x", "jog_y", "jog_z", "jog_u", "lock", "move_arc", "move_circular", "process_events", "run_standalone", "select_device", "stop_standalone", "set_device_name", "set_digital_outputs", "set_encoder_x", "set_encoder_y", "set_encoder_z", "set_encoder_u", "set_high_speed", "set_low_speed", "set_non_volatile_var", "set_on_fly_position", "set_on_fly_speed", "set_on_fly_speed_mode", "set_polarity", "set_pulse_x", "set_pulse_y", "set_pulse_z", "set_pulse_u", "set_step_n_params", "set_volatile_var", "stop_imm_x", "stop_imm_y", "stop_imm_z", "stop_imm_u", "stop_slow_x", "stop_slow_y", "stop_slow_z", "stop_slow_u", "store_perm", "unlock", "wait_til_idle", "zero_counter", "zero_position"]
                      }
                      frame Default {
                        w525 = T19[] [enum."process_events"] items=["-------------------------", "about", "adjust_goto_buttons", "check_model", "close", "connect", "disable_all", "disable_step_n_loop", "enable_all", "enabled_state_change", "enable_step_n_loop", "exit", "get_device_id", "get_device_name", "get_digital_inputs", "get_digital_outputs", "get_firmware_ver", "get_high_speed", "get_high_speed_global", "get_low_speed", "get_low_speed_global", "get_non_volatile_var", "get_on_fly_speed_mode", "get_polarity", "get_product_id", "get_sspd_mode", "get_step_n_params", "get_volatile_var", "goto_x", "goto_y", "goto_z", "goto_u", "goto_interp", "home_x", "home_y", "home_z", "home_u", "init", "init_ui", "jog_x", "jog_y", "jog_z", "jog_u", "lock", "move_arc", "move_circular", "process_events", "run_standalone", "select_device", "stop_standalone", "set_device_name", "set_digital_outputs", "set_encoder_x", "set_encoder_y", "set_encoder_z", "set_encoder_u", "set_high_speed", "set_low_speed", "set_non_volatile_var", "set_on_fly_position", "set_on_fly_speed", "set_on_fly_speed_mode", "set_polarity", "set_pulse_x", "set_pulse_y", "set_pulse_z", "set_pulse_u", "set_step_n_params", "set_volatile_var", "stop_imm_x", "stop_imm_y", "stop_imm_z", "stop_imm_u", "stop_slow_x", "stop_slow_y", "stop_slow_z", "stop_slow_u", "store_perm", "unlock", "wait_til_idle", "zero_counter", "zero_position"]
                      }
                    }
                  }
                  event "set_step_n_params": Value Change {
                    n175 = event-data() -> ()  [unwired: 1 in, 6 out]
                    n176 = local read "set_n_correct_attempts"() -> (w528:T10)
                    n177 = local read "set_n_tolerance?"() -> (w529:T10)
                    n178 = local read "set_n_err_range?"() -> (w530:T10)
                    n179 = local read "set_n_ratio?"() -> (w527:T10)
                    n180 = Compound Arithmetic op=OR(w527, w529, w530, w528) -> (w526:T10)
                    n181 = case shown="False" w526 {
                      tunnel: [w533 w535] -> w532
                      frame True {
                        w533 = T19[] [enum."set_step_n_params", enum."get_step_n_params", enum."store_perm", enum."process_events"] items=["-------------------------", "about", "adjust_goto_buttons", "check_model", "close", "connect", "disable_all", "disable_step_n_loop", "enable_all", "enabled_state_change", "enable_step_n_loop", "exit", "get_device_id", "get_device_name", "get_digital_inputs", "get_digital_outputs", "get_firmware_ver", "get_high_speed", "get_high_speed_global", "get_low_speed", "get_low_speed_global", "get_non_volatile_var", "get_on_fly_speed_mode", "get_polarity", "get_product_id", "get_sspd_mode", "get_step_n_params", "get_volatile_var", "goto_x", "goto_y", "goto_z", "goto_u", "goto_interp", "home_x", "home_y", "home_z", "home_u", "init", "init_ui", "jog_x", "jog_y", "jog_z", "jog_u", "lock", "move_arc", "move_circular", "process_events", "run_standalone", "select_device", "stop_standalone", "set_device_name", "set_digital_outputs", "set_encoder_x", "set_encoder_y", "set_encoder_z", "set_encoder_u", "set_high_speed", "set_low_speed", "set_non_volatile_var", "set_on_fly_position", "set_on_fly_speed", "set_on_fly_speed_mode", "set_polarity", "set_pulse_x", "set_pulse_y", "set_pulse_z", "set_pulse_u", "set_step_n_params", "set_volatile_var", "stop_imm_x", "stop_imm_y", "stop_imm_z", "stop_imm_u", "stop_slow_x", "stop_slow_y", "stop_slow_z", "stop_slow_u", "store_perm", "unlock", "wait_til_idle", "zero_counter", "zero_position"]
                      }
                      frame False {
                        w535 = T19[] [enum."process_events"] items=["-------------------------", "about", "adjust_goto_buttons", "check_model", "close", "connect", "disable_all", "disable_step_n_loop", "enable_all", "enabled_state_change", "enable_step_n_loop", "exit", "get_device_id", "get_device_name", "get_digital_inputs", "get_digital_outputs", "get_firmware_ver", "get_high_speed", "get_high_speed_global", "get_low_speed", "get_low_speed_global", "get_non_volatile_var", "get_on_fly_speed_mode", "get_polarity", "get_product_id", "get_sspd_mode", "get_step_n_params", "get_volatile_var", "goto_x", "goto_y", "goto_z", "goto_u", "goto_interp", "home_x", "home_y", "home_z", "home_u", "init", "init_ui", "jog_x", "jog_y", "jog_z", "jog_u", "lock", "move_arc", "move_circular", "process_events", "run_standalone", "select_device", "stop_standalone", "set_device_name", "set_digital_outputs", "set_encoder_x", "set_encoder_y", "set_encoder_z", "set_encoder_u", "set_high_speed", "set_low_speed", "set_non_volatile_var", "set_on_fly_position", "set_on_fly_speed", "set_on_fly_speed_mode", "set_polarity", "set_pulse_x", "set_pulse_y", "set_pulse_z", "set_pulse_u", "set_step_n_params", "set_volatile_var", "stop_imm_x", "stop_imm_y", "stop_imm_z", "stop_imm_u", "stop_slow_x", "stop_slow_y", "stop_slow_z", "stop_slow_u", "store_perm", "unlock", "wait_til_idle", "zero_counter", "zero_position"]
                        n182 = One Button Dialog(message="One or more items must\nbe checked before\nattempting to write\nparameters to memory.") -> ()  [unwired: 1 in, 1 out]
                      }
                    }
                  }
                  event Value Change {
                    w537 = T19[] [enum."get_step_n_params", enum."process_events"] items=["-------------------------", "about", "adjust_goto_buttons", "check_model", "close", "connect", "disable_all", "disable_step_n_loop", "enable_all", "enabled_state_change", "enable_step_n_loop", "exit", "get_device_id", "get_device_name", "get_digital_inputs", "get_digital_outputs", "get_firmware_ver", "get_high_speed", "get_high_speed_global", "get_low_speed", "get_low_speed_global", "get_non_volatile_var", "get_on_fly_speed_mode", "get_polarity", "get_product_id", "get_sspd_mode", "get_step_n_params", "get_volatile_var", "goto_x", "goto_y", "goto_z", "goto_u", "goto_interp", "home_x", "home_y", "home_z", "home_u", "init", "init_ui", "jog_x", "jog_y", "jog_z", "jog_u", "lock", "move_arc", "move_circular", "process_events", "run_standalone", "select_device", "stop_standalone", "set_device_name", "set_digital_outputs", "set_encoder_x", "set_encoder_y", "set_encoder_z", "set_encoder_u", "set_high_speed", "set_low_speed", "set_non_volatile_var", "set_on_fly_position", "set_on_fly_speed", "set_on_fly_speed_mode", "set_polarity", "set_pulse_x", "set_pulse_y", "set_pulse_z", "set_pulse_u", "set_step_n_params", "set_volatile_var", "stop_imm_x", "stop_imm_y", "stop_imm_z", "stop_imm_u", "stop_slow_x", "stop_slow_y", "stop_slow_z", "stop_slow_u", "store_perm", "unlock", "wait_til_idle", "zero_counter", "zero_position"]
                    n183 = event-data() -> ()  [unwired: 1 in, 6 out]
                  }
                  event "sspd_set_mode": Value Change {
                    w539 = T19[] [enum."set_on_fly_speed_mode", enum."store_perm", enum."get_on_fly_speed_mode", enum."process_events"] items=["-------------------------", "about", "adjust_goto_buttons", "check_model", "close", "connect", "disable_all", "disable_step_n_loop", "enable_all", "enabled_state_change", "enable_step_n_loop", "exit", "get_device_id", "get_device_name", "get_digital_inputs", "get_digital_outputs", "get_firmware_ver", "get_high_speed", "get_high_speed_global", "get_low_speed", "get_low_speed_global", "get_non_volatile_var", "get_on_fly_speed_mode", "get_polarity", "get_product_id", "get_sspd_mode", "get_step_n_params", "get_volatile_var", "goto_x", "goto_y", "goto_z", "goto_u", "goto_interp", "home_x", "home_y", "home_z", "home_u", "init", "init_ui", "jog_x", "jog_y", "jog_z", "jog_u", "lock", "move_arc", "move_circular", "process_events", "run_standalone", "select_device", "stop_standalone", "set_device_name", "set_digital_outputs", "set_encoder_x", "set_encoder_y", "set_encoder_z", "set_encoder_u", "set_high_speed", "set_low_speed", "set_non_volatile_var", "set_on_fly_position", "set_on_fly_speed", "set_on_fly_speed_mode", "set_polarity", "set_pulse_x", "set_pulse_y", "set_pulse_z", "set_pulse_u", "set_step_n_params", "set_volatile_var", "stop_imm_x", "stop_imm_y", "stop_imm_z", "stop_imm_u", "stop_slow_x", "stop_slow_y", "stop_slow_z", "stop_slow_u", "store_perm", "unlock", "wait_til_idle", "zero_counter", "zero_position"]
                    n184 = event-data() -> ()  [unwired: 1 in, 6 out]
                  }
                  event "t_set_position": Value Change {
                    w541 = T19[] [enum."set_on_fly_position", enum."process_events"] items=["-------------------------", "about", "adjust_goto_buttons", "check_model", "close", "connect", "disable_all", "disable_step_n_loop", "enable_all", "enabled_state_change", "enable_step_n_loop", "exit", "get_device_id", "get_device_name", "get_digital_inputs", "get_digital_outputs", "get_firmware_ver", "get_high_speed", "get_high_speed_global", "get_low_speed", "get_low_speed_global", "get_non_volatile_var", "get_on_fly_speed_mode", "get_polarity", "get_product_id", "get_sspd_mode", "get_step_n_params", "get_volatile_var", "goto_x", "goto_y", "goto_z", "goto_u", "goto_interp", "home_x", "home_y", "home_z", "home_u", "init", "init_ui", "jog_x", "jog_y", "jog_z", "jog_u", "lock", "move_arc", "move_circular", "process_events", "run_standalone", "select_device", "stop_standalone", "set_device_name", "set_digital_outputs", "set_encoder_x", "set_encoder_y", "set_encoder_z", "set_encoder_u", "set_high_speed", "set_low_speed", "set_non_volatile_var", "set_on_fly_position", "set_on_fly_speed", "set_on_fly_speed_mode", "set_polarity", "set_pulse_x", "set_pulse_y", "set_pulse_z", "set_pulse_u", "set_step_n_params", "set_volatile_var", "stop_imm_x", "stop_imm_y", "stop_imm_z", "stop_imm_u", "stop_slow_x", "stop_slow_y", "stop_slow_z", "stop_slow_u", "store_perm", "unlock", "wait_til_idle", "zero_counter", "zero_position"]
                    n185 = event-data() -> ()  [unwired: 1 in, 6 out]
                  }
                  event "sspd_set_speed": Value Change {
                    w543 = T19[] [enum."set_on_fly_speed", enum."process_events"] items=["-------------------------", "about", "adjust_goto_buttons", "check_model", "close", "connect", "disable_all", "disable_step_n_loop", "enable_all", "enabled_state_change", "enable_step_n_loop", "exit", "get_device_id", "get_device_name", "get_digital_inputs", "get_digital_outputs", "get_firmware_ver", "get_high_speed", "get_high_speed_global", "get_low_speed", "get_low_speed_global", "get_non_volatile_var", "get_on_fly_speed_mode", "get_polarity", "get_product_id", "get_sspd_mode", "get_step_n_params", "get_volatile_var", "goto_x", "goto_y", "goto_z", "goto_u", "goto_interp", "home_x", "home_y", "home_z", "home_u", "init", "init_ui", "jog_x", "jog_y", "jog_z", "jog_u", "lock", "move_arc", "move_circular", "process_events", "run_standalone", "select_device", "stop_standalone", "set_device_name", "set_digital_outputs", "set_encoder_x", "set_encoder_y", "set_encoder_z", "set_encoder_u", "set_high_speed", "set_low_speed", "set_non_volatile_var", "set_on_fly_position", "set_on_fly_speed", "set_on_fly_speed_mode", "set_polarity", "set_pulse_x", "set_pulse_y", "set_pulse_z", "set_pulse_u", "set_step_n_params", "set_volatile_var", "stop_imm_x", "stop_imm_y", "stop_imm_z", "stop_imm_u", "stop_slow_x", "stop_slow_y", "stop_slow_z", "stop_slow_u", "store_perm", "unlock", "wait_til_idle", "zero_counter", "zero_position"]
                    n186 = event-data() -> ()  [unwired: 1 in, 6 out]
                  }
                  event "goto_x", "goto_y", "goto_z", "goto_u": Value Change {
                    w545 = T19[] [enum."adjust_goto_buttons", enum."process_events"] items=["-------------------------", "about", "adjust_goto_buttons", "check_model", "close", "connect", "disable_all", "disable_step_n_loop", "enable_all", "enabled_state_change", "enable_step_n_loop", "exit", "get_device_id", "get_device_name", "get_digital_inputs", "get_digital_outputs", "get_firmware_ver", "get_high_speed", "get_high_speed_global", "get_low_speed", "get_low_speed_global", "get_non_volatile_var", "get_on_fly_speed_mode", "get_polarity", "get_product_id", "get_sspd_mode", "get_step_n_params", "get_volatile_var", "goto_x", "goto_y", "goto_z", "goto_u", "goto_interp", "home_x", "home_y", "home_z", "home_u", "init", "init_ui", "jog_x", "jog_y", "jog_z", "jog_u", "lock", "move_arc", "move_circular", "process_events", "run_standalone", "select_device", "stop_standalone", "set_device_name", "set_digital_outputs", "set_encoder_x", "set_encoder_y", "set_encoder_z", "set_encoder_u", "set_high_speed", "set_low_speed", "set_non_volatile_var", "set_on_fly_position", "set_on_fly_speed", "set_on_fly_speed_mode", "set_polarity", "set_pulse_x", "set_pulse_y", "set_pulse_z", "set_pulse_u", "set_step_n_params", "set_volatile_var", "stop_imm_x", "stop_imm_y", "stop_imm_z", "stop_imm_u", "stop_slow_x", "stop_slow_y", "stop_slow_z", "stop_slow_u", "store_perm", "unlock", "wait_til_idle", "zero_counter", "zero_position"]
                    n187 = event-data() -> ()  [unwired: 1 in, 6 out]
                  }
                  event "goto_interp": Value Change {
                    w547 = T19[] [enum."goto_interp", enum."process_events"] items=["-------------------------", "about", "adjust_goto_buttons", "check_model", "close", "connect", "disable_all", "disable_step_n_loop", "enable_all", "enabled_state_change", "enable_step_n_loop", "exit", "get_device_id", "get_device_name", "get_digital_inputs", "get_digital_outputs", "get_firmware_ver", "get_high_speed", "get_high_speed_global", "get_low_speed", "get_low_speed_global", "get_non_volatile_var", "get_on_fly_speed_mode", "get_polarity", "get_product_id", "get_sspd_mode", "get_step_n_params", "get_volatile_var", "goto_x", "goto_y", "goto_z", "goto_u", "goto_interp", "home_x", "home_y", "home_z", "home_u", "init", "init_ui", "jog_x", "jog_y", "jog_z", "jog_u", "lock", "move_arc", "move_circular", "process_events", "run_standalone", "select_device", "stop_standalone", "set_device_name", "set_digital_outputs", "set_encoder_x", "set_encoder_y", "set_encoder_z", "set_encoder_u", "set_high_speed", "set_low_speed", "set_non_volatile_var", "set_on_fly_position", "set_on_fly_speed", "set_on_fly_speed_mode", "set_polarity", "set_pulse_x", "set_pulse_y", "set_pulse_z", "set_pulse_u", "set_step_n_params", "set_volatile_var", "stop_imm_x", "stop_imm_y", "stop_imm_z", "stop_imm_u", "stop_slow_x", "stop_slow_y", "stop_slow_z", "stop_slow_u", "store_perm", "unlock", "wait_til_idle", "zero_counter", "zero_position"]
                    n188 = event-data() -> ()  [unwired: 1 in, 6 out]
                  }
                  event "dig_outs": Value Change {
                    w549 = T19[] [enum."set_digital_outputs", enum."process_events"] items=["-------------------------", "about", "adjust_goto_buttons", "check_model", "close", "connect", "disable_all", "disable_step_n_loop", "enable_all", "enabled_state_change", "enable_step_n_loop", "exit", "get_device_id", "get_device_name", "get_digital_inputs", "get_digital_outputs", "get_firmware_ver", "get_high_speed", "get_high_speed_global", "get_low_speed", "get_low_speed_global", "get_non_volatile_var", "get_on_fly_speed_mode", "get_polarity", "get_product_id", "get_sspd_mode", "get_step_n_params", "get_volatile_var", "goto_x", "goto_y", "goto_z", "goto_u", "goto_interp", "home_x", "home_y", "home_z", "home_u", "init", "init_ui", "jog_x", "jog_y", "jog_z", "jog_u", "lock", "move_arc", "move_circular", "process_events", "run_standalone", "select_device", "stop_standalone", "set_device_name", "set_digital_outputs", "set_encoder_x", "set_encoder_y", "set_encoder_z", "set_encoder_u", "set_high_speed", "set_low_speed", "set_non_volatile_var", "set_on_fly_position", "set_on_fly_speed", "set_on_fly_speed_mode", "set_polarity", "set_pulse_x", "set_pulse_y", "set_pulse_z", "set_pulse_u", "set_step_n_params", "set_volatile_var", "stop_imm_x", "stop_imm_y", "stop_imm_z", "stop_imm_u", "stop_slow_x", "stop_slow_y", "stop_slow_z", "stop_slow_u", "store_perm", "unlock", "wait_til_idle", "zero_counter", "zero_position"]
                    n189 = event-data() -> ()  [unwired: 1 in, 6 out]
                  }
                  event Menu Selection (User) {
                    n190 = event-data() -> ("ItemTag"=w552:string)  [unwired: 1 in, 6 out]
                    n191 = To Lower Case(string=w552) -> (all lower case string=w551:string)
                    n192 = case shown="\"exit\"" w551 {
                      tunnel: w554 -> [w556 w558]
                      tunnel: [w556 w558] -> w553
                      tunnel: [w555 w557] -> w550
                      frame "exit" {
                        w555 = T19[] [enum."disable_all", enum."close"] items=["-------------------------", "about", "adjust_goto_buttons", "check_model", "close", "connect", "disable_all", "disable_step_n_loop", "enable_all", "enabled_state_change", "enable_step_n_loop", "exit", "get_device_id", "get_device_name", "get_digital_inputs", "get_digital_outputs", "get_firmware_ver", "get_high_speed", "get_high_speed_global", "get_low_speed", "get_low_speed_global", "get_non_volatile_var", "get_on_fly_speed_mode", "get_polarity", "get_product_id", "get_sspd_mode", "get_step_n_params", "get_volatile_var", "goto_x", "goto_y", "goto_z", "goto_u", "goto_interp", "home_x", "home_y", "home_z", "home_u", "init", "init_ui", "jog_x", "jog_y", "jog_z", "jog_u", "lock", "move_arc", "move_circular", "process_events", "run_standalone", "select_device", "stop_standalone", "set_device_name", "set_digital_outputs", "set_encoder_x", "set_encoder_y", "set_encoder_z", "set_encoder_u", "set_high_speed", "set_low_speed", "set_non_volatile_var", "set_on_fly_position", "set_on_fly_speed", "set_on_fly_speed_mode", "set_polarity", "set_pulse_x", "set_pulse_y", "set_pulse_z", "set_pulse_u", "set_step_n_params", "set_volatile_var", "stop_imm_x", "stop_imm_y", "stop_imm_z", "stop_imm_u", "stop_slow_x", "stop_slow_y", "stop_slow_z", "stop_slow_u", "store_perm", "unlock", "wait_til_idle", "zero_counter", "zero_position"]
                      }
                      frame "about", Default {
                        w557 = T19[] [enum."about", enum."process_events"] items=["-------------------------", "about", "adjust_goto_buttons", "check_model", "close", "connect", "disable_all", "disable_step_n_loop", "enable_all", "enabled_state_change", "enable_step_n_loop", "exit", "get_device_id", "get_device_name", "get_digital_inputs", "get_digital_outputs", "get_firmware_ver", "get_high_speed", "get_high_speed_global", "get_low_speed", "get_low_speed_global", "get_non_volatile_var", "get_on_fly_speed_mode", "get_polarity", "get_product_id", "get_sspd_mode", "get_step_n_params", "get_volatile_var", "goto_x", "goto_y", "goto_z", "goto_u", "goto_interp", "home_x", "home_y", "home_z", "home_u", "init", "init_ui", "jog_x", "jog_y", "jog_z", "jog_u", "lock", "move_arc", "move_circular", "process_events", "run_standalone", "select_device", "stop_standalone", "set_device_name", "set_digital_outputs", "set_encoder_x", "set_encoder_y", "set_encoder_z", "set_encoder_u", "set_high_speed", "set_low_speed", "set_non_volatile_var", "set_on_fly_position", "set_on_fly_speed", "set_on_fly_speed_mode", "set_polarity", "set_pulse_x", "set_pulse_y", "set_pulse_z", "set_pulse_u", "set_step_n_params", "set_volatile_var", "stop_imm_x", "stop_imm_y", "stop_imm_z", "stop_imm_u", "stop_slow_x", "stop_slow_y", "stop_slow_z", "stop_slow_u", "store_perm", "unlock", "wait_til_idle", "zero_counter", "zero_position"]
                      }
                    }
                  }
                }
              }
              frame "run_standalone" {
                n193 = call "send_receive_command.vi"("reference (in)"=w563, "ASCII Command (in)"="SR0=1", "error in (no error)"=w564) -> ("reference (out)"=w560:refnum<class "_Controller.lvclass">, "error out"=w559:errorcluster)  [unwired: 12 in, 3 out]
              }
              frame "stop_standalone" {
                n194 = call "send_receive_command.vi"("reference (in)"=w569, "ASCII Command (in)"="SR0=0", "error in (no error)"=w570) -> ("reference (out)"=w568:refnum<class "_Controller.lvclass">, "error out"=w567:errorcluster)  [unwired: 12 in, 3 out]
              }
              frame "set_device_name" {
                n195 = call "getModel.vi"("error in (no error)"=w579, "reference (in)"=w576) -> ("error out"=w578:errorcluster, "model"=w577:T20, "reference (out)"=w575:refnum<class "_Controller.lvclass">)  [unwired: 7 in]
                n196 = case shown="\"PMX-4EX-SA\"" w577 {
                  selector: w577 -> [w596 w600]
                  tunnel: ["" "4EX"] -> w574
                  tunnel: [FALSE TRUE] -> w572
                  tunnel: [w596 w600] -> w571
                  frame Default {
                  }
                  frame "PMX-4EX-SA" {
                  }
                }
                n197 = case shown="True" w572 {
                  tunnel: [w583 w595] -> w582
                  tunnel: [w587 w594] -> w581
                  tunnel: w578 -> [w583 w593]
                  tunnel: w575 -> [w587 w592]
                  tunnel: w574 -> [_ w590]
                  tunnel: "device_name_id_to_set" -> [_ w589]
                  tunnel: w571 -> [w585 _]
                  frame False {
                    n198 = Format Into String(format string="Set Device Name for \ndevice type '%s' is not\nsupported in this app", w585) -> (resulting string=w584:string)  [unwired: 2 in, 1 out]
                    n199 = One Button Dialog(message=w584) -> ()  [unwired: 1 in, 1 out]
                  }
                  frame True {
                    n200 = Format Into String(format string="DN=%s%02d", w590, w589) -> (resulting string=w588:string)  [unwired: 2 in, 1 out]
                    n201 = call "send_receive_command.vi"("reference (in)"=w592, "ASCII Command (in)"=w588, "error in (no error)"=w593) -> ("reference (out)"=w594:refnum<class "_Controller.lvclass">, "error out"=w595:errorcluster)  [unwired: 12 in, 3 out]
                  }
                }
              }
              frame "set_digital_outputs" {
                w604 = T27[] [enum."DIG_OUT_1", enum."DIG_OUT_2", enum."DIG_OUT_3", enum."DIG_OUT_4", enum."DIG_OUT_5", enum."DIG_OUT_6", enum."DIG_OUT_7", enum."DIG_OUT_8"] items=["DIG_OUT_1", "DIG_OUT_2", "DIG_OUT_3", "DIG_OUT_4", "DIG_OUT_5", "DIG_OUT_6", "DIG_OUT_7", "DIG_OUT_8"]
                n202 = Cluster To Array(cluster="dig_outs") -> (array=w603:bool[])
                n203 = for {
                  shift-right: [w614] -> w608
                  shift-left: w609 -> [w615]
                  shift-right: [w612] -> w606
                  shift-left: w607 -> [w613]
                  tunnel: w604 -> [w611] mode=indexing
                  tunnel: w603 -> [w610] mode=indexing
                  n204 = call "setDigitalOutput.vi"("Controller in"=w615, "digital_output_ch"=w611, "dig_out_value"=w610, "error in (no error)"=w613) -> ("Controller out"=w614:refnum<class "_Controller.lvclass">, "error out"=w612:errorcluster)  [unwired: 12 in, 2 out]
                }
              }
              frame "set_encoder_x".."set_encoder_u" {
                n205 = case shown="\"set_encoder_u\"" w617 {
                  tunnel: [w624 w627 w630 w633] -> w616
                  frame "set_encoder_x", Default {
                    n206 = Format Into String(format string="EX=%d", "encoder_set_val_x") -> (resulting string=w624:string)  [unwired: 2 in, 1 out]
                  }
                  frame "set_encoder_y" {
                    n207 = Format Into String(format string="EY=%d", "encoder_set_val_y") -> (resulting string=w627:string)  [unwired: 2 in, 1 out]
                  }
                  frame "set_encoder_z" {
                    n208 = Format Into String(format string="EZ=%d", "encoder_set_val_z") -> (resulting string=w630:string)  [unwired: 2 in, 1 out]
                  }
                  frame "set_encoder_u" {
                    n209 = Format Into String(format string="EZ=%d", "encoder_set_val_u") -> (resulting string=w633:string)  [unwired: 2 in, 1 out]
                  }
                }
                n210 = call "send_receive_command.vi"("reference (in)"=w620, "ASCII Command (in)"=w616, "error in (no error)"=w622) -> ("reference (out)"=w619:refnum<class "_Controller.lvclass">, "error out"=w621:errorcluster)  [unwired: 12 in, 3 out]
              }
              frame "set_high_speed" {
                n211 = Build Array("X.high_speed", "Y.high_speed", "Z.high_speed") -> (w639:i32[])
                n212 = for {
                  tunnel: w644 -> [w651]
                  tunnel: w643 -> [w650]
                  tunnel: [w649] -> w642
                  tunnel: [w648] -> w641
                  tunnel: string[] ["HSX=%d", "HSY=%d", "HSZ=%d"] -> [w647] mode=indexing
                  tunnel: w639 -> [w646] mode=indexing
                  n213 = Format Into String(format string=w647, w646) -> (resulting string=w645:string)  [unwired: 2 in, 1 out]
                  n214 = call "send_receive_command.vi"("reference (in)"=w650, "ASCII Command (in)"=w645, "error in (no error)"=w651) -> ("reference (out)"=w649:refnum<class "_Controller.lvclass">, "error out"=w648:errorcluster)  [unwired: 12 in, 3 out]
                }
              }
              frame "set_low_speed" {
                n215 = Build Array("X.low_speed", "Y.low_speed", "Z.low_speed") -> (w653:i32[])
                n216 = for {
                  tunnel: w661 -> [w668]
                  tunnel: w660 -> [w667]
                  tunnel: [w666] -> w659
                  tunnel: [w665] -> w658
                  tunnel: string[] ["LSX=%d", "LSY=%d", "LSZ=%d"] -> [w664] mode=indexing
                  tunnel: w653 -> [w663] mode=indexing
                  n217 = Format Into String(format string=w664, w663) -> (resulting string=w662:string)  [unwired: 2 in, 1 out]
                  n218 = call "send_receive_command.vi"("reference (in)"=w667, "ASCII Command (in)"=w662, "error in (no error)"=w668) -> ("reference (out)"=w666:refnum<class "_Controller.lvclass">, "error out"=w665:errorcluster)  [unwired: 12 in, 3 out]
                }
              }
              frame "set_non_volatile_var" {
                n219 = Number To Decimal String(number="non_vol_var_write") -> (decimal integer string=w672:string)  [unwired: 1 in]
                n220 = call-dynamic "setVariableStatus.vi"("Controller in"=w671, "var_number"="non_vol_var_num", "var_value"=w672, "error in (no error)"=w675) -> ("Controller out"=w670:refnum<class "_Controller.lvclass">, "error out"=w669:errorcluster)  [unwired: 12 in, 2 out]
              }
              frame "set_on_fly_position" {
                n221 = call-dynamic "setOnTheFlyPositionChange.vi"("Controller in"=w681, "axis (for multi-axis applications only)"="t_axis", "target_position"="t_position", "error in (no error)"=w683) -> ("Controller out"=w680:refnum<class "_Controller.lvclass">, "error out"=w682:errorcluster)  [unwired: 12 in, 2 out]
              }
              frame "set_on_fly_speed" {
                n222 = local read "sspd_axis"() -> (w685:T8)
                n223 = call-dynamic "setOnTheFlySpeed.vi"("Controller in"=w688, "axis"=w685, "speed"="sspd_speed", "error in (no error)"=w690) -> ("Controller out"=w687:refnum<class "_Controller.lvclass">, "error out"=w689:errorcluster)  [unwired: 12 in, 2 out]
              }
              frame "set_on_fly_speed_mode" {
                n224 = Format Into String(format string="SSPDM%s=%d", "sspd_axis", "sspd_mode") -> (resulting string=w696:string)  [unwired: 2 in, 1 out]
                n225 = call "send_receive_command.vi"("reference (in)"=w695, "ASCII Command (in)"=w696, "error in (no error)"=w698) -> ("reference (out)"=w694:refnum<class "_Controller.lvclass">, "error out"=w697:errorcluster)  [unwired: 12 in, 3 out]
              }
              frame "set_polarity" {
                n226 = Bundle By Name(cluster=T15 {"item"=enum."DIRECTION", "status"=FALSE} ("items_group"), "item"="polarity_option", "status"="polarity_val") -> (w705:T15)
                n227 = Build Array(w705) -> (w704:T15[])
                n228 = call-dynamic "setPolarity.vi"("Controller in"=w710, "polarity_items (in)"=w704, "axis (in)"="polarity_axis", "error in (no error)"=w709) -> ("Controller out"=w700:refnum<class "_Controller.lvclass">, "error out"=w701:errorcluster)  [unwired: 12 in, 2 out]
              }
              frame "set_pulse_x".."set_pulse_u" {
                n229 = case shown="\"set_pulse_x\", Default" w712 {
                  tunnel: [w718 w722 w725 w728] -> w711
                  frame "set_pulse_x", Default {
                    n230 = Format Into String(format string="PX=%d", "pulse_set_val_x") -> (resulting string=w718:string)  [unwired: 2 in, 1 out]
                  }
                  frame "set_pulse_y" {
                    n231 = Format Into String(format string="PY=%d", "pulse_set_val_y") -> (resulting string=w722:string)  [unwired: 2 in, 1 out]
                  }
                  frame "set_pulse_z" {
                    n232 = Format Into String(format string="PZ=%d", "pulse_set_val_z") -> (resulting string=w725:string)  [unwired: 2 in, 1 out]
                  }
                  frame "set_pulse_u" {
                    n233 = Format Into String(format string="PU=%d", "pulse_set_val_u") -> (resulting string=w728:string)  [unwired: 2 in, 1 out]
                  }
                }
                n234 = call "send_receive_command.vi"("reference (in)"=w715, "ASCII Command (in)"=w711, "error in (no error)"=w717) -> ("reference (out)"=w714:refnum<class "_Controller.lvclass">, "error out"=w716:errorcluster)  [unwired: 12 in, 3 out]
              }
              frame "set_step_n_params" {
                w739 = T29 {"step_N_loop_ratio"=0.0, "tolerance (encoder counts)"=0, "error_range"=0, "max_num_correction_attempts"=0, "enabled?"=FALSE}  # step_n_params
                w741 = T30 {"set_ratio?"=FALSE, "set_tolerance?"=FALSE, "set_err_range?"=FALSE, "set_correct_attempts?"=FALSE}  # set_params?
                n235 = Bundle By Name(cluster=w739, "step_N_loop_ratio"="step_n_ratio", "tolerance (encoder counts)"="step_n_tolerance", "error_range"="step_n_err_range", "max_num_correction_attempts"="step_n_max_corr") -> (w738:T29)
                n236 = Bundle By Name(cluster=w741, "set_ratio?"="set_n_ratio?", "set_tolerance?"="set_n_tolerance?", "set_err_range?"="set_n_err_range?", "set_correct_attempts?"="set_n_correct_attempts") -> (w740:T30)
                n237 = local read "step_n_axis"() -> (w742:T8)
                n238 = call-dynamic "setStepNLoopParams.vi"("Controller in"=w745, "axis (only applicable to multi-axis applications)"=w742, "set_params?"=w740, "step_n_params"=w738, "error in (no error)"=w747) -> ("Controller out"=w744:refnum<class "_Controller.lvclass">, "error out"=w746:errorcluster)  [unwired: 11 in, 2 out]
              }
              frame "set_volatile_var" {
                n239 = Number To Decimal String(number="vol_var_write") -> (decimal integer string=w753:string)  [unwired: 1 in]
                n240 = call-dynamic "setVariableStatus.vi"("Controller in"=w752, "var_number"="vol_var_num", "var_value"=w753, "error in (no error)"=w754) -> ("Controller out"=w748:refnum<class "_Controller.lvclass">, "error out"=w749:errorcluster)  [unwired: 12 in, 2 out]
              }
              frame "stop_imm_x".."stop_imm_u" {
                n241 = case shown="\"stop_imm_u\"" w757 {
                  tunnel: ["ABORTX" "ABORTY" "ABORTZ" "ABORTU"] -> w756
                  frame "stop_imm_x", Default {
                  }
                  frame "stop_imm_y" {
                  }
                  frame "stop_imm_z" {
                  }
                  frame "stop_imm_u" {
                  }
                }
                n242 = call "send_receive_command.vi"("reference (in)"=w760, "ASCII Command (in)"=w756, "error in (no error)"=w762) -> ("reference (out)"=w759:refnum<class "_Controller.lvclass">, "error out"=w761:errorcluster)  [unwired: 12 in, 3 out]
              }
              frame "stop_slow_x".."stop_slow_u" {
                n243 = case shown="\"stop_slow_x\", Default" w768 {
                  tunnel: ["STOPX" "STOPY" "STOPZ" "STOPU"] -> w767
                  frame "stop_slow_x", Default {
                  }
                  frame "stop_slow_y" {
                  }
                  frame "stop_slow_z" {
                  }
                  frame "stop_slow_u" {
                  }
                }
                n244 = call "send_receive_command.vi"("reference (in)"=w771, "ASCII Command (in)"=w767, "error in (no error)"=w773) -> ("reference (out)"=w770:refnum<class "_Controller.lvclass">, "error out"=w772:errorcluster)  [unwired: 12 in, 3 out]
              }
              frame "store_perm" {
                n245 = call "storePerm.vi"("_Controller in"=w781, "error in (no error)"=w779) -> ("_Controller out"=w780:refnum<class "_Controller.lvclass">, "error out"=w778:errorcluster)  [unwired: 16 in]
              }
              frame "wait_til_idle" {
                n246 = while {
                  shift-right: [w794] -> w784
                  shift-left: w787 -> [w801]
                  shift-right: [w802] -> w785
                  shift-left: w786 -> [w803]
                  stop <- w791 stop-if-true
                  w795 = motor_status."IDLE" ("X.motion_state")
                  n247 = call-dynamic "getStatus.vi"("reference (in)"=w803, "error in (no error)"=w801) -> ("reference (out)"=w802:refnum<class "_Controller.lvclass">, "full_state"=w800:T16, "error out"=w794:errorcluster)  [unwired: 14 in, 1 out]
                  n248 = Unbundle By Name(w800) -> ("X.motion_state"=w796:T2, "Y.motion_state"=w789:T2, "Z.motion_state"=w788:T2)
                  n249 = Equal?(x=w796, y=w795) -> (x = y?=w798:bool)
                  n250 = Equal?(x=w788, y=w795) -> (x = y?=w797:bool)
                  n251 = Equal?(x=w789, y=w795) -> (x = y?=w799:bool)
                  n252 = Unbundle By Name(w794) -> ("status"=w792:bool)
                  n253 = Compound Arithmetic op=AND(w798, w799, w797) -> (w793:bool)
                  n254 = Or(x=w793, y=w792) -> (x .or. y?=w791:bool)
                  n255 = Wait (ms)(milliseconds to wait=u32 20) -> ()  [unwired: 1 out]
                }
              }
              frame "zero_counter" {
                n256 = for {
                  tunnel: w809 -> [w814]
                  tunnel: w808 -> [w813]
                  tunnel: [w812] -> w807
                  tunnel: [w811] -> w806
                  tunnel: string[] ["EX=0", "EY=0", "EZ=0"] -> [w810] mode=indexing
                  n257 = call "send_receive_command.vi"("reference (in)"=w813, "ASCII Command (in)"=w810, "error in (no error)"=w814) -> ("reference (out)"=w812:refnum<class "_Controller.lvclass">, "error out"=w811:errorcluster)  [unwired: 12 in, 3 out]
                }
              }
              frame "zero_position" {
                n258 = for {
                  tunnel: w820 -> [w825]
                  tunnel: w819 -> [w824]
                  tunnel: [w823] -> w818
                  tunnel: [w822] -> w817
                  tunnel: string[] ["PX=0", "PY=0", "PZ=0", "PU=0"] -> [w821] mode=indexing
                  n259 = call "send_receive_command.vi"("reference (in)"=w824, "ASCII Command (in)"=w821, "error in (no error)"=w825) -> ("reference (out)"=w823:refnum<class "_Controller.lvclass">, "error out"=w822:errorcluster)  [unwired: 12 in, 3 out]
                }
              }
            }
            n260 = case shown="No Error" errorcluster {"status"=FALSE, "code"=0, "source"=""} ("error IO") {
              selector: errorcluster {"status"=FALSE, "code"=0, "source"=""} ("error IO") -> [w111 w114]
              tunnel: [w113 w116] -> w102
              tunnel: w104 -> [w113 _]
              tunnel: [w112 w115] -> w101
              tunnel: w103 -> [w112 w115]
              tunnel: [w111 w114] -> w100
              frame No Error {
              }
              frame Error {
                w116 = T19[] [enum."close"] items=["-------------------------", "about", "adjust_goto_buttons", "check_model", "close", "connect", "disable_all", "disable_step_n_loop", "enable_all", "enabled_state_change", "enable_step_n_loop", "exit", "get_device_id", "get_device_name", "get_digital_inputs", "get_digital_outputs", "get_firmware_ver", "get_high_speed", "get_high_speed_global", "get_low_speed", "get_low_speed_global", "get_non_volatile_var", "get_on_fly_speed_mode", "get_polarity", "get_product_id", "get_sspd_mode", "get_step_n_params", "get_volatile_var", "goto_x", "goto_y", "goto_z", "goto_u", "goto_interp", "home_x", "home_y", "home_z", "home_u", "init", "init_ui", "jog_x", "jog_y", "jog_z", "jog_u", "lock", "move_arc", "move_circular", "process_events", "run_standalone", "select_device", "stop_standalone", "set_device_name", "set_digital_outputs", "set_encoder_x", "set_encoder_y", "set_encoder_z", "set_encoder_u", "set_high_speed", "set_low_speed", "set_non_volatile_var", "set_on_fly_position", "set_on_fly_speed", "set_on_fly_speed_mode", "set_polarity", "set_pulse_x", "set_pulse_y", "set_pulse_z", "set_pulse_u", "set_step_n_params", "set_volatile_var", "stop_imm_x", "stop_imm_y", "stop_imm_z", "stop_imm_u", "stop_slow_x", "stop_slow_y", "stop_slow_z", "stop_slow_u", "store_perm", "unlock", "wait_til_idle", "zero_counter", "zero_position"]
              }
            }
            n261 = Empty Array?(array=w102) -> (empty?=w99:bool)
            n262 = Unbundle By Name(w100) -> ("status"=w98:bool)
            n263 = Or(x=w99, y=w98) -> (x .or. y?=w97:bool)
          }
        }
        frame Error {
        }
      }
      n264 = case shown="No Error" w85 {
        selector: w85 -> [w831 w982]
        tunnel: [w830 w982] -> w88
        tunnel: w86 -> [w829 _]
        frame No Error {
          n265 = local read "exit?"() -> (w828:bool)
          n266 = case shown="False" w828 {
            tunnel: w831 -> [w835 w981]
            tunnel: [w834 w981] -> w830
            tunnel: w829 -> [w833 _]
            frame False {
              n267 = Build Array(multi_axis_read_realtime_actions."build_processes" ("actions")) -> (w832:T24[])
              n268 = while {
                shift-right: [w846] -> _
                shift-left: w832 -> [w849]
                shift-right: [w839] -> _
                shift-left: w833 -> [w838]
                shift-right: [w841] -> w834
                shift-left: w835 -> [w842]
                stop <- w840 stop-if-true
                # "Loop for Retrieving Realtime Parameters"
                n269 = Delete From Array(array=w849, index=0) -> (deleted portion=w847:T24, array with subset deleted=w845:T24[])  [unwired: 1 in]
                n270 = case shown="\"encoder_value\"" w847 {
                  tunnel: w845 -> [_ w867 w879 w896 w905 w920 w938 w972 w980]
                  tunnel: [w852 w867 w879 w896 w905 w920 w938 w972 w980] -> w846
                  tunnel: [w851 w853 w881 w897 w908 w923 w941 w976 w979] -> w841
                  tunnel: w842 -> [w851 w870 w882 w898 w909 w924 w942 w977 w979]
                  tunnel: [w850 w868 w884 w900 w906 w921 w939 w973 w978] -> w839
                  tunnel: w838 -> [w850 w869 w883 w899 w907 w922 w940 w974 w978]
                  frame "build_processes", Default {
                    w852 = T24[] [enum."motion_state", enum."snl_motion_state", enum."encoder_value", enum."position_value", enum."digital_inputs", enum."analog_inputs", enum."pulse_value", enum."build_processes"] items=["analog_inputs", "build_processes", "check_status", "encoder_value", "digital_inputs", "motion_state", "position_value", "pulse_value", "snl_motion_state"]
                  }
                  frame "analog_inputs" {
                    n271 = for {
                      N: 8 -> [_]
                      tunnel: [w877] -> w864 mode=indexing
                      shift-right: [w875] -> w853
                      shift-left: w870 -> [w876]
                      tunnel: w869 -> [w874]
                      tunnel: [w873] -> w868
                      i -> [w872]
                      n272 = Increment(x=w872) -> (x+1=w871:i32)
                      n273 = call-dynamic "readAnalogInputChannel.vi"("Controller in"=w874, "ai_channel (def=1)"=w871, "error in (no error)"=w876) -> ("Controller out"=w873:refnum<class "_Controller.lvclass">, "value (V)"=w877:dbl, "error out"=w875:errorcluster)  [unwired: 14 in]
                    }
                    n274 = Index Array(array=w864, index #1=0 ("index")) -> (element #1=w862:dbl, element #2=w861:dbl, element #3=w860:dbl, element #4=w859:dbl, element #5=w858:dbl, element #6=w857:dbl, element #7=w856:dbl, element #8=w855:dbl)  [unwired: 7 in]
                    n275 = local read "analog_inputs"() -> (w865:T13)
                    n276 = Bundle By Name(cluster=w865, "Analog Input 1"=w862, "Analog Input 2"=w861, "Analog Input 3"=w860, "Analog Input 4"=w859, "Analog Input 5"=w858, "Analog Input 6"=w857, "Analog Input 7"=w856, "Analog Input 8"=w855) -> (→"analog_inputs":T13)
                  }
                  frame "encoder_value" {
                    # "This is one of the few cases where a\n\"to more specific class\" approach is\nrequired for executing a controller\nmethod.  The Controller class does \nnot contain an abstract method for\nretrieve counter position.  Therefore,\nthere is no base class to override.  That\nsaid, the incoming Controller class\nreference must be be further specified\nas a \"Multi Axix Controller\" object\nberfore this method can execute."
                    n277 = To More Specific Class(target class=refnum<class "_MultiAxisController.lvclass"> refnum ("classes.lvlib:_MultiAxisController.lvclass"), reference=w883) -> (specific class reference=w886:refnum<class "_MultiAxisController.lvclass">)  [unwired: 1 in, 1 out]
                    n278 = call-dynamic "getCounterPosition.vi"("MultiAxisController in"=w886, "type (def = ENCODER)"=counter_type."ENCODER", "error in (no error)"=w882) -> ("MultiAxisController out"=w884:refnum<class "_MultiAxisController.lvclass">, "counter_vals (out)"=w887:T31, "error out"=w881:errorcluster)  [unwired: 14 in]
                    n279 = Unbundle By Name(w887) -> ("X"=→"X.encoder":i32, "Y"=→"Y.encoder":i32, "Z"=→"Z.encoder":i32, "U"=→"U.encoder":i32)
                  }
                  frame "pulse_value" {
                    # "This is one of the few cases where a\n\"to more specific class\" approach is\nrequired for executing a controller\nmethod.  The Controller class does \nnot contain an abstract method for\nretrieve pulse position.  Therefore,\nthere is no base class to override.  That\nsaid, the incoming Controller class\nreference must be be further specified\nas a \"Multi Axix Controller\" object\nberfore this method can execute."
                    n280 = To More Specific Class(target class=refnum<class "_MultiAxisController.lvclass"> refnum ("classes.lvlib:_MultiAxisController.lvclass"), reference=w899) -> (specific class reference=w902:refnum<class "_MultiAxisController.lvclass">)  [unwired: 1 in, 1 out]
                    n281 = call-dynamic "getCounterPosition.vi"("MultiAxisController in"=w902, "type (def = ENCODER)"=counter_type."PULSE", "error in (no error)"=w898) -> ("MultiAxisController out"=w900:refnum<class "_MultiAxisController.lvclass">, "counter_vals (out)"=w903:T31, "error out"=w897:errorcluster)  [unwired: 14 in]
                    n282 = Unbundle By Name(w903) -> ("X"=→"X.pulse":i32, "Y"=→"Y.pulse":i32, "Z"=→"Z.pulse":i32, "U"=→"U.pulse":i32)
                  }
                  frame "motion_state" {
                    n283 = call-dynamic "getStatus.vi"("reference (in)"=w907, "error in (no error)"=w909) -> ("reference (out)"=w906:refnum<class "_Controller.lvclass">, "full_state"=w913:T16, "error out"=w908:errorcluster)  [unwired: 14 in, 1 out]
                    "full_state" <- w913
                    n284 = Unbundle By Name(w913) -> ("X.motion_state"=→"X.motion_state":T2, "Y.motion_state"=→"Y.motion_state":T2, "Z.motion_state"=→"Z.motion_state":T2, "U.motion_state"=→"U.motion_state":T2)
                  }
                  frame "position_value" {
                    w925 = T8[] [enum."X", enum."Y", enum."Z", enum."U"] items=["X", "Y", "Z", "U"]
                    n285 = for {
                      tunnel: w922 -> [w931]
                      tunnel: w925 -> [w928] mode=indexing
                      tunnel: w924 -> [w930]
                      tunnel: [w927] -> w923
                      tunnel: [w926] -> w921
                      tunnel: [w929] -> w918 mode=indexing
                      n286 = call-dynamic "getCurrentPosition.vi"("reference (in)"=w931, "axis (def=X)"=w928, "error in (no error)"=w930) -> ("reference (out)"=w926:refnum<class "_Controller.lvclass">, "current_position (units)"=w929:i32, "error out"=w927:errorcluster)  [unwired: 14 in]
                    }
                    n287 = Index Array(array=w918, index #1=0 ("index")) -> (element #1=→"X.pos":i32, element #2=→"Y.pos":i32, element #3=→"Z.pos":i32, element #4=→"U.pos":i32)  [unwired: 3 in]
                  }
                  frame "snl_motion_state" {
                    w943 = T8[] [enum."X", enum."Y", enum."Z", enum."U"] items=["X", "Y", "Z", "U"]
                    n288 = for {
                      tunnel: w940 -> [w949]
                      tunnel: w943 -> [w946] mode=indexing
                      tunnel: w942 -> [w948]
                      tunnel: [w945] -> w941
                      tunnel: [w944] -> w939
                      tunnel: [w947] -> w936 mode=indexing
                      n289 = call-dynamic "getStepNLoopStatus.vi"("Controller in"=w949, "axis (for use in multi-axis applications only)"=w946, "error in (no error)"=w948) -> ("Controller out"=w944:refnum<class "_Controller.lvclass">, "status (out)"=w947:T1, "error out"=w945:errorcluster)  [unwired: 14 in]
                    }
                    n290 = Index Array(array=w936, index #1=0 ("index")) -> (element #1=→"X.SNL_motion_state":T1, element #2=→"Y.SNL_motion_state":T1, element #3=→"Z.SNL_motion_state":T1, element #4=→"U.SNL_motion_state":T1)  [unwired: 3 in]
                  }
                  frame "digital_inputs" {
                    w975 = TRUE  # get_all? (def=F)
                    n291 = call "getDigitalInputsStatus.vi"("Controller in"=w974, "get_all? (def=F)"=w975, "error in (no error)"=w977) -> ("Controller out"=w973:refnum<class "_Controller.lvclass">, "di_items"=w971:T32[], "error out"=w976:errorcluster)  [unwired: 12 in, 2 out]
                    n292 = Array Subset(array=w971, length=8) -> (w968:T32[])  [unwired: 1 in]
                    n293 = Index Array(array=w968, index #1=0 ("index")) -> (element #1=w966:T32, element #2=w964:T32, element #3=w963:T32, element #4=w962:T32, element #5=w961:T32, element #6=w960:T32, element #7=w959:T32, element #8=w958:T32)  [unwired: 7 in]
                    n294 = Unbundle By Name(w966) -> ("status"=w965:bool)
                    n295 = Unbundle By Name(w964) -> ("status"=w957:bool)
                    n296 = Unbundle By Name(w963) -> ("status"=w956:bool)
                    n297 = Unbundle By Name(w962) -> ("status"=w955:bool)
                    n298 = Unbundle By Name(w961) -> ("status"=w954:bool)
                    n299 = Unbundle By Name(w960) -> ("status"=w953:bool)
                    n300 = Unbundle By Name(w959) -> ("status"=w952:bool)
                    n301 = Unbundle By Name(w958) -> ("status"=w951:bool)
                    n302 = local read "digital_ins"() -> (w969:T12)
                    n303 = Bundle By Name(cluster=w969, "Digital Input 1"=w965, "Digital Input 2"=w957, "Digital Input 3"=w956, "Digital Input 4"=w955, "Digital Input 5"=w954, "Digital Input 6"=w953, "Digital Input 7"=w952, "Digital Input 8"=w951) -> (→"digital_ins":T12)
                  }
                  frame "check_status" {
                  }
                }
                n304 = Unbundle By Name(w841) -> ("status"=w843:bool)
                n305 = local read "exit?"() -> (w844:bool)
                n306 = Or(x=w844, y=w843) -> (x .or. y?=w840:bool)
                n307 = Wait (ms)(milliseconds to wait=u32 10) -> ()  [unwired: 1 out]
              }
            }
            frame True {
            }
          }
        }
        frame Error {
        }
      }
    }
    frame True {
    }
  }
  n308 = Merge Errors(w14, w13) -> (w7:errorcluster)
  n309 = call "getModel.vi"("error in (no error)"=w7, "reference (in)"=w6) -> ("error out"=w4:errorcluster, "model"=w5:T20, "reference (out)"=w3:refnum<class "_Controller.lvclass">)  [unwired: 7 in]
  n310 = case shown="Default" w5 {
    tunnel: w4 -> [w985 w988]
    tunnel: [w985 w987] -> w2
    tunnel: w3 -> [_ w986]
    frame "<unrecognized>" {
    }
    frame Default {
      n311 = call "close_connection.vi"("reference (in)"=w986, "error in (no error)"=w988) -> ("error out"=w987:errorcluster)  [unwired: 16 in, 1 out]
    }
  }
  n312 = flat-sequence {
    tunnel: w2 -> [w989]
    tunnel: [w989] -> w1
    frame #0 {
      n313 = Current VI's Path() -> (path=w991:path)
      n314 = call "get_exe_home_path.vi"("home_path"=w991) -> ("running in an executable?"=w990:bool)  [unwired: 6 in, 1 out]
      n315 = Quit LabVIEW(quit? (T)=w990) -> ()
    }
  }
  "Error Out" <- w1
